vi "Probe_ESR_Verification.vi"() -> ()   [LabVIEW 2020]
uses:
  Instruments/Vector Network Analyzer/Controls/Sparameter cluster.ctl
  Instruments/Vector Network Analyzer/VNA-ZNB/VNA-ZNB.lvclass
  Instruments/Vector Network Analyzer/Vector Network Analyzer.lvclass
  C:/Sandbox/Git_Sandbox/WiSpry Test Framework source code (LV20)/WiSpry Test Framework/Instruments/Instrument.lvclass
  Instruments/Vector Network Analyzer/VNA-Ag87xx/VNA-Ag87xx.lvclass
  Instruments/Vector Network Analyzer/VNA-ENA/VNA-ENA.lvclass
  C:/Sandbox/Git_Sandbox/WiSpry Test Framework source code (LV20)/WiSpry Test Framework/Instruments/Vector Network Analyzer/Vector Network Analyzer.lvclass
  Instruments/Vector Network Analyzer/VNA-FieldFox/VNA-FieldFox.lvclass
  Instruments/Instrument.lvclass/Instrument.ctl
  <vilib>/addons/HF Network Analysis/Support VIs/Read SnP File (SnP).vi
  <vilib>/addons/HF Network Analysis/NI_HFNetworkAnalysis.lvlib
  Instruments/Instrument.lvclass
panel:
  out "Shunt Resistance":cluster{"Frequencies (Hz)":dbl[], dbl[]}[](graph)
  in  "VISA resource name":refnum<visa-resource-name>="GPIB0::24::INSTR"
  in  "Min Loop Delay (ms)":u32=2000
  in  "stop":bool
  in  "VNA ports":bool[](array[boolean])=[TRUE, TRUE, FALSE, FALSE]
  out "error out":errorcluster
  in  "error in (no error)":errorcluster
  out "S parameters":T1[](array[typedef])=[{"Frequency"=100000.0, "S Parameters"=[1.00063102545-0.00317405238764i, -7.98294684912e-06+3.80004461168e-06i, -9.89227074681e-06+6.97421338234e-06i, 1.00037660372-0.00266654479791i]}, {"Frequency"=5412437.5, "S Parameters"=[0.999589465299-0.00884373938232i, 1.79466351697e-05+0.00108431519392i, -4.77312747689e-05+0.00108840175147i, 0.999264902062-0.00912969708227i]}, {"Frequency"=10724875.0, "S Parameters"=[0.999494373608-0.0176199367958i, 4.11591256995e-05+0.00213681933704i, 3.83120105072e-05+0.00214881958037i, 0.999275380418-0.0180876415298i]}, {"Frequency"=16037312.5, "S Parameters"=[0.999282063454-0.0261251603072i, 8.13206404428e-05+0.00319368968947i, 8.47417919346e-05+0.00320723135129i, 0.999053623411-0.0270577569269i]}, {"Frequency"=21349750.0, "S Parameters"=[0.99906596023-0.034829301326i, 0.000151915131114+0.00425103048761i, 0.000150636990312+0.00427010832182i, 0.998740112702-0.0358850792968i]}, {"Frequency"=26662187.5, "S Parameters"=[0.998715362497-0.0435746112421i, 0.000234659139297+0.00531483419357i, 0.000235376905721+0.00533080558281i, 0.998594136554-0.0448224191034i]}, {"Frequency"=31974625.0, "S Parameters"=[0.998281901504-0.0521668079996i, 0.000338128346419+0.00636537125827i, 0.000334413081756+0.00639109675178i, 0.998175718066-0.0537300663822i]}, {"Frequency"=37287062.5, "S Parameters"=[0.997838086619-0.0607938999828i, 0.000461144482836+0.00741328025649i, 0.000459259121093+0.00743917316995i, 0.997503941205-0.0625111061962i]}, {"Frequency"=42599500.0, "S Parameters"=[0.997301968613-0.0694104406755i, 0.000598647928574+0.00846671626162i, 0.000598991319687+0.00849745924638i, 0.996767834563-0.0713509671284i]}, {"Frequency"=47911937.5, "S Parameters"=[0.996738500175-0.0781355874827i, 0.00076500598186+0.00952078341747i, 0.000756830766138+0.00954951785153i, 0.996165848801-0.0802924359967i]}, {"Frequency"=53224375.0, "S Parameters"=[0.995935887891-0.0867413890739i, 0.000935135496371+0.0105724006276i, 0.000930398477704+0.0105994515656i, 0.995431755326-0.0891744067202i]}, {"Frequency"=58536812.5, "S Parameters"=[0.995133720611-0.0953832879489i, 0.00113382618367+0.0116128119096i, 0.00112500139336+0.0116503317168i, 0.99455094616-0.0979411527267i]}, {"Frequency"=63849250.0, "S Parameters"=[0.994282619127-0.104018437494i, 0.00134607137472+0.0126520756157i, 0.00133748264184+0.012683381439i, 0.993711947585-0.106706905878i]}, {"Frequency"=69161687.5, "S Parameters"=[0.993312980895-0.112559684303i, 0.00157379963675+0.0136973250881i, 0.0015692313252+0.0137371922269i, 0.992690963519-0.115458073775i]}, {"Frequency"=74474125.0, "S Parameters"=[0.992169037066-0.121189214253i, 0.00182431843167+0.0147267134348i, 0.00182427780941+0.014777438941i, 0.991560855793-0.124163931681i]}, {"Frequency"=79786562.5, "S Parameters"=[0.991034206753-0.129908888951i, 0.00208671197242+0.0157700205624i, 0.00208852040958+0.0158076067585i, 0.990465792271-0.13280288183i]}, {"Frequency"=85099000.0, "S Parameters"=[0.989888897268-0.138525429622i, 0.00236552862787+0.0167963759004i, 0.00237608265702+0.0168444023872i, 0.98918672108-0.141409756953i]}, {"Frequency"=90411437.5, "S Parameters"=[0.988605222646-0.147144211174i, 0.0026748304552+0.0178246861595i, 0.00268143391082+0.0178659609454i, 0.987792003195-0.150202067637i]}, {"Frequency"=95723875.0, "S Parameters"=[0.987126158904-0.155668326581i, 0.00300270219103+0.018849837706i, 0.00300633583591+0.0188876377234i, 0.98650322677-0.158733542088i]}, {"Frequency"=101036312.5, "S Parameters"=[0.985729529386-0.164429733932i, 0.003342637213+0.019866815485i, 0.00334986844833+0.0199059321685i, 0.985007567168-0.167494141546i]}, {"Frequency"=106348750.0, "S Parameters"=[0.984145047702-0.173009157642i, 0.00370726024826+0.0208751436204i, 0.00370504834329+0.0209018177297i, 0.983494178049-0.176169746823i]}, {"Frequency"=111661187.5, "S Parameters"=[0.982531329981-0.181577975756i, 0.00407539580636+0.0218759411548i, 0.00408254152419+0.0219074554705i, 0.981921526896-0.184855225871i]}, {"Frequency"=116973625.0, "S Parameters"=[0.980942320193-0.190103877786i, 0.00447690972486+0.022883152241i, 0.00446462121407+0.0228866566375i, 0.980236781773-0.193521635504i]}, {"Frequency"=122286062.5, "S Parameters"=[0.979267726477-0.19860375658i, 0.00489476368483+0.0238764594776i, 0.004886375881+0.023872559194i, 0.978522333805-0.202225294481i]}, {"Frequency"=127598500.0, "S Parameters"=[0.97745032036-0.207014881573i, 0.00531411046366+0.0248597210447i, 0.00531499623159+0.0248611893595i, 0.976598530543-0.210843463605i]}, {"Frequency"=132910937.5, "S Parameters"=[0.975642374558-0.215402303724i, 0.00576005483985+0.0258598491544i, 0.00575535538642+0.0258562889893i, 0.974718766285-0.219406816475i]}, {"Frequency"=138223375.0, "S Parameters"=[0.973779428409-0.223714838767i, 0.00620125629282+0.0268525306285i, 0.0062150730737+0.0268593271773i, 0.972777098117-0.228067706274i]}, {"Frequency"=143535812.5, "S Parameters"=[0.971864538252-0.231914322701i, 0.0066698240782+0.0278545247324i, 0.00669008917111+0.0278587055618i, 0.970740525182-0.236637927309i]}, {"Frequency"=148848250.0, "S Parameters"=[0.969858602818-0.24017398174i, 0.00714484521601+0.0288240094733i, 0.00717944034219+0.0288455550671i, 0.968579769524-0.245224863132i]}, {"Frequency"=154160687.5, "S Parameters"=[0.967651604237-0.248352144434i, 0.00765838225549+0.0297911059014i, 0.00768294313807+0.0297998019629i, 0.966448068571-0.253680445193i]}, {"Frequency"=159473125.0, "S Parameters"=[0.965543712114-0.256521744478i, 0.00818962389069+0.0307310624261i, 0.0082211800598+0.0307625609364i, 0.964159725636-0.262205556328i]}, {"Frequency"=164785562.5, "S Parameters"=[0.96335337765-0.264663605956i, 0.00876310221848+0.03166301653i, 0.00877210655779+0.0316950178866i, 0.961821785853-0.270651731496i]}, {"Frequency"=170098000.0, "S Parameters"=[0.961126337593-0.272808308947i, 0.00934062112452+0.0325851442338i, 0.00933990780437+0.032637563282i, 0.959344260473-0.279201035756i]}, {"Frequency"=175410437.5, "S Parameters"=[0.95868103847-0.280857081294i, 0.00993632555241+0.0334996882576i, 0.00992616476105+0.0335484023094i, 0.956752441906-0.287451413347i]}, {"Frequency"=180722875.0, "S Parameters"=[0.956111696266-0.288907064473i, 0.0105479433039+0.0344099917136i, 0.0105194114406+0.0344549228692i, 0.954058536085-0.295745111224i]}, {"Frequency"=186035312.5, "S Parameters"=[0.953438240007-0.297005345647i, 0.011154811883+0.035309936005i, 0.0111504453256+0.0353622915195i, 0.951369766025-0.304053743839i]}, {"Frequency"=191347750.0, "S Parameters"=[0.950854267844-0.305135135687i, 0.0118065287014+0.0362019195547i, 0.0117773805531+0.0362606828664i, 0.948445293457-0.312352376139i]}, {"Frequency"=196660187.5, "S Parameters"=[0.948163629123-0.313306920281i, 0.0124573244177+0.0371009663331i, 0.0124228215186+0.0371566342657i, 0.945697371816-0.320691681687i]}, {"Frequency"=201972625.0, "S Parameters"=[0.945510619226-0.321503691859i, 0.0131130876497+0.0379772095792i, 0.0130861846599+0.0380412858467i, 0.942752796157-0.329091441074i]}, {"Frequency"=207285062.5, "S Parameters"=[0.942720117993-0.329598124505i, 0.0138046739658+0.0388469308322i, 0.0137691724802+0.038916705868i, 0.939877390723-0.337385698885i]}, {"Frequency"=212597500.0, "S Parameters"=[0.939738477428-0.337674230529i, 0.0144851430877+0.0397092340249i, 0.0144560807582+0.0397675182765i, 0.93680182358-0.345504771036i]}, {"Frequency"=217909937.5, "S Parameters"=[0.93663277494-0.345707563034i, 0.0151908676727+0.0405526276046i, 0.0151649299722+0.0406193604774i, 0.933582875935-0.353711316818i]}, {"Frequency"=223222375.0, "S Parameters"=[0.933517598665-0.353872545933i, 0.0159174295466+0.0413924449798i, 0.0159035934482+0.0414574207915i, 0.930330599299-0.361905072381i]}, {"Frequency"=228534812.5, "S Parameters"=[0.93033297528-0.361965447476i, 0.0166747471873+0.0422192563767i, 0.0166489433405+0.0422957168236i, 0.927123433755-0.370150755983i]}, {"Frequency"=233847250.0, "S Parameters"=[0.927088808025-0.370109531166i, 0.0174401322567+0.0430328490142i, 0.0174154172761+0.0431134621313i, 0.923788961735-0.378435441607i]}, {"Frequency"=239159687.5, "S Parameters"=[0.923835292828-0.378306111926i, 0.018223140396+0.0438558269936i, 0.0182121991047+0.0439232862196i, 0.920428121155-0.386655669362i]}, {"Frequency"=244472125.0, "S Parameters"=[0.920371852944-0.386385688171i, 0.0190121292772+0.0446421698344i, 0.0190166229403+0.0447201527773i, 0.916914037433-0.394932787633i]}, {"Frequency"=249784562.5, "S Parameters"=[0.916902278884-0.394458025771i, 0.0198196055669+0.0454280145577i, 0.0198392019368+0.045505608285i, 0.913340158274-0.402934235509i]}, {"Frequency"=255097000.0, "S Parameters"=[0.913274178207-0.402331018193i, 0.02064440953+0.046201470566i, 0.0206499341348+0.0462814568028i, 0.90963607178-0.410919796982i]}, {"Frequency"=260409437.5, "S Parameters"=[0.909443454757-0.410265624646i, 0.0214646749005+0.0469362085321i, 0.0214864653688+0.0470207233435i, 0.905853045196-0.418831053746i]}, {"Frequency"=265721875.0, "S Parameters"=[0.905528988824-0.418142569854i, 0.0223150187518+0.0476575186441i, 0.0223311485529+0.0477642836673i, 0.901908982895-0.426632350287i]}, {"Frequency"=271034312.5, "S Parameters"=[0.901723584779-0.426082738643i, 0.0231902469163+0.0483790402853i, 0.0232004553339+0.0485009765555i, 0.89791245714-0.434590648877i]}, {"Frequency"=276346750.0, "S Parameters"=[0.897712427224-0.433975986603i, 0.0240742237401+0.0490802597868i, 0.0240751967848+0.0492246181039i, 0.893882999092-0.44247426666i]}, {"Frequency"=281659187.5, "S Parameters"=[0.893865687096-0.442023719168i, 0.0249623640111+0.0497794440534i, 0.0249646307093+0.0499333671103i, 0.88985726475-0.450328757258i]}, {"Frequency"=286971625.0, "S Parameters"=[0.889862751082-0.44971670209i, 0.0258712811882+0.050458713556i, 0.0258578159208+0.0506158891927i, 0.885752624932-0.458126842961i]}, {"Frequency"=292284062.5, "S Parameters"=[0.885948665325-0.45743698911i, 0.0267723294974+0.0511306857042i, 0.0267546501657+0.0512938719607i, 0.881755407578-0.465840892567i]}, {"Frequency"=297596500.0, "S Parameters"=[0.882010908203-0.464947823659i, 0.0276911929797+0.0517861331747i, 0.0276624697611+0.0519700884475i, 0.877655277138-0.473393459149i]}, {"Frequency"=302908937.5, "S Parameters"=[0.877895367719-0.472237437836i, 0.0286089085133+0.0524462839516i, 0.0285737476463+0.0526083353161i, 0.873389220201-0.480777133903i]}, {"Frequency"=308221375.0, "S Parameters"=[0.873730319648-0.479579595673i, 0.0295306670691+0.0530839527557i, 0.0295097458178+0.0532290761638i, 0.86908046-0.488190826053i]}, {"Frequency"=313533812.5, "S Parameters"=[0.869502610713-0.48687619568i, 0.0304902651296+0.0537170427797i, 0.0304502934163+0.0538338230389i, 0.864783830391-0.495718273581i]}, {"Frequency"=318846250.0, "S Parameters"=[0.86536131508-0.494041353269i, 0.0314430105507+0.0543631836035i, 0.0314343793546+0.0544412165234i, 0.86043056023-0.50297290057i]}, {"Frequency"=324158687.5, "S Parameters"=[0.861101958051-0.501219109139i, 0.0324163421203+0.0549798985744i, 0.0324408757901+0.0550453222631i, 0.855902533376-0.510362440212i]}, {"Frequency"=329471125.0, "S Parameters"=[0.856790946408-0.508440878483i, 0.0334061528754+0.0556010151243i, 0.0334443069802+0.0556165063967i, 0.851467855791-0.517830817251i]}, {"Frequency"=334783562.5, "S Parameters"=[0.852504965756-0.515638294093i, 0.0344265507048+0.0561953452312i, 0.034472083246+0.0562000701666i, 0.846852096741-0.525172965022i]}, {"Frequency"=340096000.0, "S Parameters"=[0.848223335605-0.522834872411i, 0.0354529947731+0.0567842918775i, 0.0355104835193+0.0567651452848i, 0.842287633675-0.532688661039i]}, {"Frequency"=345408437.5, "S Parameters"=[0.843776876771-0.529849159751i, 0.0364824957151+0.0573676534415i, 0.0365586722173+0.0573231992306i, 0.837600930932-0.539966617959i]}, {"Frequency"=350720875.0, "S Parameters"=[0.839192629354-0.536820222493i, 0.0375118522588+0.0579177012483i, 0.0376174747675+0.0578693578765i, 0.83270253535-0.547033038051i]}, {"Frequency"=356033312.5, "S Parameters"=[0.834445445728-0.543747254366i, 0.0385684217528+0.0584310680257i, 0.0386668668805+0.0583952036463i, 0.827662438937-0.554318170324i]}, {"Frequency"=361345750.0, "S Parameters"=[0.829592983985-0.550741502233i, 0.0396452864452+0.058929027604i, 0.0397361347819+0.0589183368508i, 0.822650176586-0.561367866726i]}, {"Frequency"=366658187.5, "S Parameters"=[0.824564699915-0.557812446697i, 0.0407427716736+0.0594142207705i, 0.0408107962368+0.0593953549477i, 0.817435327165-0.568694712837i]}, {"Frequency"=371970625.0, "S Parameters"=[0.819574977073-0.564915115575i, 0.0418456361+0.0598759028534i, 0.0418988472337+0.0599005185004i, 0.812175410235-0.575744831474i]}, {"Frequency"=377283062.5, "S Parameters"=[0.814388360027-0.572091045977i, 0.0429730034406+0.0603183945285i, 0.0429872678536+0.0603435292067i, 0.806970477432-0.582971207729i]}, {"Frequency"=382595500.0, "S Parameters"=[0.809502852485-0.579172175507i, 0.0441051368128+0.0607466496275i, 0.0440878250853+0.0608084246741i, 0.801815215926-0.59009752885i]}, {"Frequency"=387907937.5, "S Parameters"=[0.804332658222-0.586167701733i, 0.0452336363873+0.0611522577662i, 0.0451849462962+0.0612286388754i, 0.796573022135-0.596995908343i]}, {"Frequency"=393220375.0, "S Parameters"=[0.799157493995-0.593065593031i, 0.0463719042317+0.0615489642622i, 0.0462857416515+0.0616423958993i, 0.791284266201-0.603844152373i]}, {"Frequency"=398532812.5, "S Parameters"=[0.79391205451-0.599924311835i, 0.0475019510099+0.0619496720782i, 0.0474051568781+0.0620315825637i, 0.785991172982-0.610558039527i]}, {"Frequency"=403845250.0, "S Parameters"=[0.788778217704-0.606655185552i, 0.0486411719472+0.0623505265199i, 0.0485377088771+0.0624126725359i, 0.780821444863-0.617192889185i]}, {"Frequency"=409157687.5, "S Parameters"=[0.783530712615-0.613295818833i, 0.0497772098106+0.062698768358i, 0.0496945812296+0.0627570840774i, 0.775486892195-0.623623820526i]}, {"Frequency"=414470125.0, "S Parameters"=[0.77820733929-0.619992321306i, 0.050936074167+0.0630697016741i, 0.0508671483103+0.0630876636642i, 0.770152571985-0.630232778601i]}, {"Frequency"=419782562.5, "S Parameters"=[0.772836148572-0.626504467508i, 0.0521288026674+0.0633783353291i, 0.0520507657099+0.0634041388604i, 0.764596100379-0.636815902177i]}, {"Frequency"=425095000.0, "S Parameters"=[0.767424170262-0.633026435217i, 0.0533043900706+0.0637117627889i, 0.0532559275066+0.0636936884446i, 0.759130623007-0.643352525514i]}, {"Frequency"=430407437.5, "S Parameters"=[0.761997679212-0.639488959115i, 0.0545106689513+0.0639946568128i, 0.0544766884357+0.0639797172283i, 0.753587638453-0.649767373366i]}, {"Frequency"=435719875.0, "S Parameters"=[0.756472262109-0.645944466079i, 0.0557056726007+0.0642909498324i, 0.0557123249982+0.0642243999468i, 0.747934758954-0.656110691818i]}, {"Frequency"=441032312.5, "S Parameters"=[0.750790337166-0.652102929128i, 0.0569155840497+0.0645461079911i, 0.0569475623612+0.0644838826163i, 0.742218207836-0.662221655766i]}, {"Frequency"=446344750.0, "S Parameters"=[0.745143695163-0.658294914948i, 0.0581141944168+0.0647843160559i, 0.0581715513229+0.0647497455839i, 0.736110747732-0.668350272847i]}, {"Frequency"=451657187.5, "S Parameters"=[0.739234247641-0.664462186289i, 0.0593287830504+0.0650134546916i, 0.0593858728144+0.0649575650675i, 0.730268615428-0.674614490715i]}, {"Frequency"=456969625.0, "S Parameters"=[0.733338337278-0.670588208003i, 0.0605640956685+0.0652023065333i, 0.0606018030058+0.0651718625086i, 0.724181204514-0.68086071557i]}, {"Frequency"=462282062.5, "S Parameters"=[0.727323292454-0.677012939928i, 0.0617976955719+0.0653836571187i, 0.0618493121326+0.0653632907481i, 0.71801648867-0.687161677924i]}, {"Frequency"=467594500.0, "S Parameters"=[0.721180102656-0.683338511352i, 0.0630531840805+0.0655317460434i, 0.0630691552869+0.0655237723636i, 0.711877821348-0.693383927429i]}, {"Frequency"=472906937.5, "S Parameters"=[0.715056132992-0.689623185694i, 0.0643249103696+0.0656398062479i, 0.0643039251735+0.0656931443031i, 0.705594951816-0.699579704496i]}, {"Frequency"=478219375.0, "S Parameters"=[0.708901824002-0.695888362785i, 0.065576682043+0.0657625277186i, 0.0655418641159+0.065816331645i, 0.699511120301-0.705688921593i]}, {"Frequency"=483531812.5, "S Parameters"=[0.702643558904-0.702096027427i, 0.0668587222734+0.0658507852596i, 0.0667826774553+0.0659223674517i, 0.693236369102-0.711736379121i]}, {"Frequency"=488844250.0, "S Parameters"=[0.696381949504-0.708338617123i, 0.0681237179335+0.0659217670994i, 0.0680349129524+0.0660057232637i, 0.686905261408-0.717657421781i]}, {"Frequency"=494156687.5, "S Parameters"=[0.69024820324-0.71423661451i, 0.0694065706979+0.066007594938i, 0.0692901344825+0.0660990310715i, 0.680648559345-0.723562997539i]}, {"Frequency"=499469125.0, "S Parameters"=[0.683878992516-0.720069238751i, 0.0706614121248+0.0660506888409i, 0.0705352056018+0.0661621518603i, 0.674314933524-0.729302727123i]}, {"Frequency"=504781562.5, "S Parameters"=[0.67765735774-0.725764776545i, 0.071918876+0.0660959512079i, 0.0717989086346+0.0662032939569i, 0.667972849895-0.734955923686i]}, {"Frequency"=510094000.0, "S Parameters"=[0.671298841094-0.731538902354i, 0.0731693546933+0.0661270859203i, 0.0730695672455+0.066225488051i, 0.66147669786-0.740548360181i]}, {"Frequency"=515406437.5, "S Parameters"=[0.664956361856-0.737217852867i, 0.0744387117538+0.0661166831921i, 0.0743496314046+0.0662153269034i, 0.654988599127-0.746174047555i]}, {"Frequency"=520718875.0, "S Parameters"=[0.658664005375-0.742773372804i, 0.075711147919+0.066103974408i, 0.0756690720924+0.0661833406382i, 0.648442140988-0.751805839216i]}, {"Frequency"=526031312.5, "S Parameters"=[0.652239932201-0.748063076522i, 0.076996186472+0.0660559163416i, 0.0769692504695+0.0661410777289i, 0.641595507546-0.75727104644i]}, {"Frequency"=531343750.0, "S Parameters"=[0.645772802832-0.753308373537i, 0.0782781036799+0.0660001682736i, 0.0782614495057+0.0660720748261i, 0.634837568913-0.762675738101i]}, {"Frequency"=536656187.5, "S Parameters"=[0.639243540198-0.758447584388i, 0.0795380771291+0.0659074629919i, 0.079575528085+0.0659716708719i, 0.627916433614-0.767844158065i]}, {"Frequency"=541968625.0, "S Parameters"=[0.632673662842-0.763543687601i, 0.0808173461883+0.0658173179721i, 0.0808657213996+0.0658693844852i, 0.62073934413-0.773207369049i]}, {"Frequency"=547281062.5, "S Parameters"=[0.626123719122-0.768700052511i, 0.0820963974813+0.0657209933489i, 0.0821853874253+0.0657734103431i, 0.613723284936-0.778585225678i]}, {"Frequency"=552593500.0, "S Parameters"=[0.619462380416-0.773755227441i, 0.0833766785012+0.0655979258002i, 0.0834833371479+0.0656312593138i, 0.606590051175-0.783862312302i]}, {"Frequency"=557905937.5, "S Parameters"=[0.613000813159-0.778868203976i, 0.084668832196+0.0654633464949i, 0.0847912954215+0.0654930092841i, 0.599622462726-0.789366063614i]}, {"Frequency"=563218375.0, "S Parameters"=[0.606264495995-0.783970903666i, 0.0859810577266+0.065285433265i, 0.0861088243739+0.0652928574811i, 0.592390894454-0.794706534192i]}, {"Frequency"=568530812.5, "S Parameters"=[0.599654918058-0.789003711758i, 0.0872746381079+0.0650901480533i, 0.0873966460723+0.0650991877521i, 0.585242834728-0.799845997629i]}, {"Frequency"=573843250.0, "S Parameters"=[0.592907200459-0.794091240443i, 0.0885817038622+0.0648851593623i, 0.0887196137592+0.0648724994204i, 0.577981526664-0.804972752397i]}, {"Frequency"=579155687.5, "S Parameters"=[0.585980944557-0.798980962821i, 0.0898975487383+0.0646487818453i, 0.0900405466608+0.0646137883089i, 0.57074380165-0.810062255945i]}, {"Frequency"=584468125.0, "S Parameters"=[0.579113969756-0.803856885489i, 0.0911973184415+0.0644296738465i, 0.0913529867057+0.0643706386572i, 0.563589247893-0.814943683832i]}, {"Frequency"=589780562.5, "S Parameters"=[0.572218650898-0.808571802939i, 0.0925177960827+0.0641742472972i, 0.0926493258312+0.0640892654375i, 0.556427328877-0.819721753221i]}, {"Frequency"=595093000.0, "S Parameters"=[0.565252888639-0.813310430635i, 0.0938070030138+0.0638961087118i, 0.0939501356548+0.0638102737035i, 0.549129157433-0.824369434062i]}, {"Frequency"=600405437.5, "S Parameters"=[0.558260130511-0.818007086325i, 0.0950905034125+0.0636177573095i, 0.0952452132801+0.0635361352387i, 0.541881907262-0.82902027769i]}, {"Frequency"=605717875.0, "S Parameters"=[0.551383962105-0.82259900329i, 0.0963677361442+0.0633349434215i, 0.0965263194209+0.0632520565912i, 0.534817068005-0.833458140245i]}, {"Frequency"=611030312.5, "S Parameters"=[0.544501299363-0.827095526201i, 0.0976577871601+0.0630390906843i, 0.097793573854+0.06293909167i, 0.527829178505-0.837769904569i]}, {"Frequency"=616342750.0, "S Parameters"=[0.537370454041-0.831504869875i, 0.0989663259905+0.0626738407556i, 0.0990784363786+0.0625815969942i, 0.520459165976-0.842067640028i]}, {"Frequency"=621655187.5, "S Parameters"=[0.530291434527-0.83572301726i, 0.10027766324+0.062296240104i, 0.100345517323+0.0622154231724i, 0.513082454146-0.846164707614i]}, {"Frequency"=626967625.0, "S Parameters"=[0.523123672041-0.839902811715i, 0.101609076916+0.0618859968706i, 0.101638045696+0.061822712959i, 0.505564751847-0.850328107763i]}, {"Frequency"=632280062.5, "S Parameters"=[0.515847197209-0.84404704414i, 0.102931533812+0.0614691329142i, 0.102905571585+0.0613900452211i, 0.497950875324-0.854398869408i]}, {"Frequency"=637592500.0, "S Parameters"=[0.508705354697-0.848129952343i, 0.104234086297+0.0610614772917i, 0.104180095722+0.0609795636739i, 0.490397216695-0.858438578937i]}, {"Frequency"=642904937.5, "S Parameters"=[0.501420465553-0.852238275235i, 0.105564299661+0.060621857435i, 0.105466771499+0.0605304015747i, 0.48277683392-0.862660914991i]}, {"Frequency"=648217375.0, "S Parameters"=[0.494263051028-0.856279265944i, 0.106874050247+0.0601737454206i, 0.106746021727+0.0600669030824i, 0.475319289168-0.866804339773i]}, {"Frequency"=653529812.5, "S Parameters"=[0.487048039027-0.860313760594i, 0.108169091111+0.0597044215349i, 0.108030588973+0.059600832678i, 0.467704078167-0.870848136957i]}, {"Frequency"=658842250.0, "S Parameters"=[0.479739307513-0.864305904978i, 0.109494910474+0.0591891917499i, 0.109327557476+0.0590834061535i, 0.460046560179-0.874880011026i]}, {"Frequency"=664154687.5, "S Parameters"=[0.4723898478-0.868228979692i, 0.110802961896+0.058680468252i, 0.110672893101+0.0585503280393i, 0.452370240397-0.878784751825i]}, {"Frequency"=669467125.0, "S Parameters"=[0.465009728218-0.872039932738i, 0.112121744195+0.0581172327766i, 0.111990627111+0.0580107098431i, 0.44462208069-0.882748168249i]}, {"Frequency"=674779562.5, "S Parameters"=[0.457427954735-0.875872592683i, 0.11341895078+0.057527667223i, 0.11333897457+0.0574317891891i, 0.436731778027-0.886348195179i]}, {"Frequency"=680092000.0, "S Parameters"=[0.449758184396-0.879487925529i, 0.114717579508+0.0568991445274i, 0.114647297665+0.0568042666825i, 0.428868231336-0.89003818492i]}, {"Frequency"=685404437.5, "S Parameters"=[0.442079198894-0.883260295475i, 0.1159895558+0.0563031422455i, 0.115973656461+0.0561961895293i, 0.42112826238-0.893604115276i]}, {"Frequency"=690716875.0, "S Parameters"=[0.434364884014-0.88696288913i, 0.117277631417+0.0556378649597i, 0.117287635135+0.0555592240809i, 0.41312840864-0.897228949146i]}, {"Frequency"=696029312.5, "S Parameters"=[0.426698221326-0.890564220841i, 0.118512794026+0.0550056838551i, 0.118558000746+0.0549291600593i, 0.405340911629-0.900584444494i]}, {"Frequency"=701341750.0, "S Parameters"=[0.419043862782-0.89411839011i, 0.119779031829+0.0543546227086i, 0.119813636212+0.0543036595544i, 0.397662299689-0.90401720617i]}, {"Frequency"=706654187.5, "S Parameters"=[0.411321821766-0.89748210318i, 0.120998937643+0.0536402691663i, 0.121025412774+0.0536114468749i, 0.389887391833-0.907079071441i]}, {"Frequency"=711966625.0, "S Parameters"=[0.403569145007-0.900740740003i, 0.122231629229+0.052938441763i, 0.122236025504+0.0529047760896i, 0.381830567398-0.910205559899i]}, {"Frequency"=717279062.5, "S Parameters"=[0.395641374117-0.903988956131i, 0.123446782356+0.0522106604013i, 0.123453766922+0.0521693747288i, 0.373963517445-0.913074668899i]}, {"Frequency"=722591500.0, "S Parameters"=[0.387831331921-0.907230241407i, 0.124674895368+0.0514288994023i, 0.124639324717+0.0514211048994i, 0.365893722565-0.915999148861i]}, {"Frequency"=727903937.5, "S Parameters"=[0.380034461493-0.910213174666i, 0.125890087398+0.0506791707926i, 0.125814873285+0.0506447136441i, 0.357963742297-0.919020287614i]}, {"Frequency"=733216375.0, "S Parameters"=[0.37222943743-0.913351479019i, 0.127094089869+0.0498896720059i, 0.126959269552+0.0498821328295i, 0.349914632687-0.921997695758i]}, {"Frequency"=738528812.5, "S Parameters"=[0.364502994792-0.916427459124i, 0.128297782903+0.0491211442222i, 0.128134042678+0.0490829576297i, 0.342189336209-0.924948641756i]}, {"Frequency"=743841250.0, "S Parameters"=[0.356864743479-0.91933735348i, 0.129459149935+0.0483269640262i, 0.129273322397+0.0482675448199i, 0.334255270547-0.92774244258i]}, {"Frequency"=749153687.5, "S Parameters"=[0.349405407125-0.92226512687i, 0.130654438931+0.0475458103177i, 0.130473388811+0.0474953498938i, 0.326460167834-0.93053488536i]}, {"Frequency"=754466125.0, "S Parameters"=[0.341870912319-0.925026119787i, 0.131822213094+0.0467545860475i, 0.131642583377+0.046698240513i, 0.318703709334-0.933231204444i]}, {"Frequency"=759778562.5, "S Parameters"=[0.334290069046-0.927511160524i, 0.132971787354+0.0459540862484i, 0.132818146055+0.045893700235i, 0.310806866589-0.935609338275i]}, {"Frequency"=765091000.0, "S Parameters"=[0.326658317141-0.930080741749i, 0.134133596112+0.0451163263279i, 0.134030337884+0.0450541593751i, 0.302872573016-0.938038963092i]}, {"Frequency"=770403437.5, "S Parameters"=[0.318889272112-0.932536771179i, 0.135326970454+0.0442393305939i, 0.135260261728+0.0441894330365i, 0.294836522403-0.940456539207i]}, {"Frequency"=775715875.0, "S Parameters"=[0.31110115001-0.935009380681i, 0.136488653244+0.043352436968i, 0.136435415734+0.0433300137784i, 0.286735317121-0.942729106003i]}, {"Frequency"=781028312.5, "S Parameters"=[0.303187030066-0.937231078137i, 0.137635315492+0.0424341089309i, 0.137647206278+0.0424351121541i, 0.278577345409-0.944976795522i]}, {"Frequency"=786340750.0, "S Parameters"=[0.295454505339-0.939616264127i, 0.13879549029+0.0415051330053i, 0.138817872744+0.0415571861569i, 0.270421561923-0.947134037998i]}, {"Frequency"=791653187.5, "S Parameters"=[0.287553822214-0.941794469701i, 0.13993458601+0.0405965508472i, 0.139998494836+0.040626335971i, 0.262429458723-0.94922210278i]}, {"Frequency"=796965625.0, "S Parameters"=[0.279659265085-0.943845740864i, 0.141031960025+0.039645151318i, 0.141132113166+0.0396940691225i, 0.254332360397-0.951076815641i]}, {"Frequency"=802278062.5, "S Parameters"=[0.271704175382-0.945877455128i, 0.142132806586+0.0386755003422i, 0.142235464911+0.03872967897i, 0.246247395847-0.952856962908i]}, {"Frequency"=807590500.0, "S Parameters"=[0.263808126146-0.947856639006i, 0.143250841601+0.0377017619258i, 0.143355607501+0.0377765985504i, 0.238041281306-0.954671462047i]}, {"Frequency"=812902937.5, "S Parameters"=[0.255822005378-0.949662366132i, 0.144346402016+0.0367181143106i, 0.144412531857+0.0367325274008i, 0.229685215586-0.956291110613i]}, {"Frequency"=818215375.0, "S Parameters"=[0.247703632343-0.951633272918i, 0.145462222438+0.0356511197499i, 0.1454651801+0.0357008644356i, 0.221305092611-0.95801092555i]}, {"Frequency"=823527812.5, "S Parameters"=[0.239645841085-0.953542600096i, 0.146522429769+0.0346328657989i, 0.146534610694+0.034628126227i, 0.213053410669-0.959791930291i]}, {"Frequency"=828840250.0, "S Parameters"=[0.231607003512-0.955444388361i, 0.147593089707+0.0335640760988i, 0.147563031924+0.0335228918968i, 0.204689490621-0.961463012338i]}, {"Frequency"=834152687.5, "S Parameters"=[0.223600745045-0.957414482021i, 0.148678137706+0.0325243396646i, 0.148625846506+0.032429941883i, 0.196561143212-0.963183326779i]}, {"Frequency"=839465125.0, "S Parameters"=[0.215666605825-0.959258163384i, 0.149713421079+0.0314326411463i, 0.14968707016+0.0313311861147i, 0.18820707522-0.964685126725i]}, {"Frequency"=844777562.5, "S Parameters"=[0.20782623822-0.960892930389i, 0.150784166152+0.030364099139i, 0.150721844274+0.0302515539173i, 0.180141420047-0.966277859997i]}, {"Frequency"=850090000.0, "S Parameters"=[0.200051077849-0.962375855075i, 0.151836080788+0.0292660601734i, 0.151768323969+0.0291558805843i, 0.171860245176-0.96744266787i]}, {"Frequency"=855402437.5, "S Parameters"=[0.192192510447-0.963826810986i, 0.152893747077+0.0281769870832i, 0.152807848892+0.0280449464101i, 0.163594587411-0.968754188247i]}, {"Frequency"=860714875.0, "S Parameters"=[0.184130320494-0.965170412097i, 0.153925065254+0.0270457634222i, 0.153848299479+0.0268871586158i, 0.155326758135-0.969824893287i]}, {"Frequency"=866027312.5, "S Parameters"=[0.176105513979-0.966378467951i, 0.154967212215+0.0259007219175i, 0.15486962542+0.0257270975193i, 0.146873700226-0.970996784025i]}, {"Frequency"=871339750.0, "S Parameters"=[0.168009770535-0.967701303539i, 0.156005220252+0.0247016964851i, 0.155917083469+0.0245531320403i, 0.138366349179-0.972056859775i]}, {"Frequency"=876652187.5, "S Parameters"=[0.159769508311-0.968834074513i, 0.15701474064+0.0234670197131i, 0.15693957835+0.0233125299611i, 0.129776118286-0.97297240355i]}, {"Frequency"=881964625.0, "S Parameters"=[0.151361369802-0.969847690592i, 0.158003996432+0.0222189546446i, 0.157940461774+0.0220294887817i, 0.121240263033-0.973687103112i]}, {"Frequency"=887277062.5, "S Parameters"=[0.142906701936-0.970787784384i, 0.158995908119+0.0209336762908i, 0.158927958953+0.02073982447i, 0.112567945121-0.974534410108i]}, {"Frequency"=892589500.0, "S Parameters"=[0.134562169644-0.97162719436i, 0.159978141666+0.0196183262033i, 0.159862552665+0.0194497166122i, 0.103918708708-0.975093251918i]}, {"Frequency"=897901937.5, "S Parameters"=[0.1260309028-0.97243567182i, 0.160890435737+0.0183012042795i, 0.160826310571+0.0181466414902i, 0.0952860647617-0.975559367784i]}, {"Frequency"=903214375.0, "S Parameters"=[0.117476278726-0.973241566019i, 0.161805041466+0.0170145325663i, 0.161705075543+0.0168317971531i, 0.0865753303627-0.97616745311i]}, {"Frequency"=908526812.5, "S Parameters"=[0.108736486073-0.973961479698i, 0.162693296387+0.0156513956653i, 0.162606289854+0.0154790172238i, 0.0779405228756-0.976576887798i]}, {"Frequency"=913839250.0, "S Parameters"=[0.100272543994-0.974810293781i, 0.163515863658+0.0142714356309i, 0.163463154889+0.0141232257608i, 0.0693137148197-0.97712993772i]}, {"Frequency"=919151687.5, "S Parameters"=[0.0916710723802-0.975546262852i, 0.164381987123+0.0128979635354i, 0.164288205657+0.0127186595611i, 0.0608190504754-0.977691747644i]}, {"Frequency"=924464125.0, "S Parameters"=[0.0831020003206-0.976241126626i, 0.165215705143+0.0115028593748i, 0.165126251386+0.0113491368025i, 0.0522746479709-0.978225406778i]}, {"Frequency"=929776562.5, "S Parameters"=[0.0747987569421-0.976948478972i, 0.166037366743+0.0101117733998i, 0.165968524275+0.00996911318224i, 0.0439541539833-0.978673649746i]}, {"Frequency"=935089000.0, "S Parameters"=[0.0665417384361-0.97738055295i, 0.166806617476+0.00873726047156i, 0.166765719161+0.00857444081628i, 0.0358017507244-0.978864720395i]}, {"Frequency"=940401437.5, "S Parameters"=[0.0584765941064-0.977817589043i, 0.167602897837+0.00734309019331i, 0.167567295043+0.0071963036243i, 0.0275523899039-0.978821340425i]}, {"Frequency"=945713875.0, "S Parameters"=[0.050411393978-0.977985188409i, 0.16834248994+0.00597810763871i, 0.168302515992+0.00582322513678i, 0.0194221735938-0.978722323246i]}, {"Frequency"=951026312.5, "S Parameters"=[0.0424877742179-0.978319302501i, 0.1691187338+0.00460311532489i, 0.16907170463+0.00447966566943i, 0.0112377031173-0.978748783543i]}, {"Frequency"=956338750.0, "S Parameters"=[0.0347224526448-0.978423068998i, 0.169844299405+0.00324527958117i, 0.169809214581+0.00312777203096i, 0.00312844680329-0.978631921843i]}, {"Frequency"=961651187.5, "S Parameters"=[0.0268893354297-0.978588896895i, 0.170595941125+0.00186607084483i, 0.17049248574+0.00177602001469i, -0.00494445208392-0.97841022052i]}, {"Frequency"=966963625.0, "S Parameters"=[0.019002863679-0.978527803423i, 0.171323823221+0.000465740509664i, 0.171189790807+0.000380798046211i, -0.0131372833982-0.97821111944i]}, {"Frequency"=972276062.5, "S Parameters"=[0.0111768488751-0.978387565435i, 0.172042195218-0.00100079724546i, 0.171845605321-0.00104965348644i, -0.0213856457888-0.977658173329i]}, {"Frequency"=977588500.0, "S Parameters"=[0.003141906885-0.978230389379i, 0.172777855462-0.00246787462386i, 0.172549211973-0.0025161066966i, -0.0297193631821-0.97712937043i]}, {"Frequency"=982900937.5, "S Parameters"=[-0.00482389513468-0.977869725153i, 0.173479771423-0.00393692683027i, 0.173203118037-0.00401489255514i, -0.0380452199843-0.976618668474i]}, {"Frequency"=988213375.0, "S Parameters"=[-0.0127424409323-0.977566447696i, 0.174170748331-0.00546043952312i, 0.173858505125-0.0054543721585i, -0.0464334289088-0.975832012928i]}, {"Frequency"=993525812.5, "S Parameters"=[-0.0208597685201-0.97706663055i, 0.174882966922-0.0069511534676i, 0.174496386159-0.00696069450891i, -0.0549095952186-0.975207249647i]}, {"Frequency"=998838250.0, "S Parameters"=[-0.0290397744921-0.97653894567i, 0.175537030817-0.00847393639668i, 0.175164943311-0.00846769505805i, -0.0633644395629-0.974428363247i]}, {"Frequency"=1004150687.5, "S Parameters"=[-0.0372430015913-0.976133384975i, 0.176155845926-0.00996730944919i, 0.175803173236-0.00998689203082i, -0.0718420014254-0.97371542929i]}, {"Frequency"=1009463125.0, "S Parameters"=[-0.0456139392387-0.975606535102i, 0.176797889222-0.0115210405176i, 0.176436931363-0.0115328799408i, -0.0803430180295-0.973070278956i]}, {"Frequency"=1014775562.5, "S Parameters"=[-0.0537776278667-0.975187892351i, 0.177353131903-0.0130957739647i, 0.177097029014-0.0130699143057i, -0.0887209952443-0.972201575433i]}, {"Frequency"=1020088000.0, "S Parameters"=[-0.0621171275905-0.974650035298i, 0.177950685899-0.0146933108401i, 0.177709348692-0.0146309909555i, -0.0970268460481-0.971425315364i]}, {"Frequency"=1025400437.5, "S Parameters"=[-0.0702903732027-0.973878080505i, 0.178458330232-0.0162988900562i, 0.178335752097-0.0162220420094i, -0.105204831502-0.970256528632i]}, {"Frequency"=1030712875.0, "S Parameters"=[-0.0785473414386-0.972978434409i, 0.178987374416-0.0179051235305i, 0.178926612594-0.0177820573783i, -0.113519593325-0.969115121756i]}, {"Frequency"=1036025312.5, "S Parameters"=[-0.086721548962-0.9722339253i, 0.179490561916-0.0195102490205i, 0.179504633267-0.0193477914736i, -0.121848433377-0.967845114249i]}, {"Frequency"=1041337750.0, "S Parameters"=[-0.0948706265247-0.971156939769i, 0.180007509858-0.0211481068918i, 0.180016140497-0.0209528003977i, -0.130109289143-0.966696387574i]}, {"Frequency"=1046650187.5, "S Parameters"=[-0.102893854439-0.970306264188i, 0.180460476247-0.0227136210812i, 0.180531053609-0.0224914255151i, -0.138020671656-0.965355346431i]}, {"Frequency"=1051962625.0, "S Parameters"=[-0.110870658769-0.969258354766i, 0.180918118253-0.0242808579739i, 0.181005954062-0.024036881757i, -0.146110366514-0.963982839728i]}, {"Frequency"=1057275062.5, "S Parameters"=[-0.118978987652-0.968110126176i, 0.181359838379-0.0258536260174i, 0.181409799594-0.0256395781014i, -0.154142267698-0.962707295173i]}, {"Frequency"=1062587500.0, "S Parameters"=[-0.126877511106-0.967067497416i, 0.181761030666-0.0274681499271i, 0.181800381643-0.0272906905124i, -0.162234690795-0.961020853611i]}, {"Frequency"=1067899937.5, "S Parameters"=[-0.134850427445-0.965721698628i, 0.182182377257-0.029096299118i, 0.182172106095-0.0289451156502i, -0.17021355985-0.95940750093i]}, {"Frequency"=1073212375.0, "S Parameters"=[-0.14289506813-0.964232229607i, 0.18257364283-0.0307226075298i, 0.182526760809-0.0306851675265i, -0.178183647077-0.957550211151i]}, {"Frequency"=1078524812.5, "S Parameters"=[-0.150901496095-0.962605660377i, 0.182982795646-0.0323711347196i, 0.182867564436-0.0324422315964i, -0.186295732755-0.955881505355i]}, {"Frequency"=1083837250.0, "S Parameters"=[-0.158995026306-0.961096060584i, 0.183336282582-0.0340295048432i, 0.183180276288-0.0341447147549i, -0.19432431561-0.953874398519i]}, {"Frequency"=1089149687.5, "S Parameters"=[-0.167106616731-0.959466935109i, 0.183683067166-0.0356715394231i, 0.183509977277-0.0358854119567i, -0.202296390188-0.952029888861i]}, {"Frequency"=1094462125.0, "S Parameters"=[-0.175285245659-0.957809095021i, 0.184036190999-0.037336488037i, 0.183837705056-0.0376174789181i, -0.210308770732-0.949980534816i]}, {"Frequency"=1099774562.5, "S Parameters"=[-0.183398413231-0.956332635258i, 0.184362773446-0.0389642876932i, 0.184152857512-0.0393010171889i, -0.218281304526-0.948221594681i]}, {"Frequency"=1105087000.0, "S Parameters"=[-0.191346530534-0.954735004124i, 0.184684530329-0.0406149025374i, 0.184499774315-0.0409037148774i, -0.226235631603-0.946288956413i]}, {"Frequency"=1110399437.5, "S Parameters"=[-0.199479622388-0.952888618135i, 0.18496191602-0.0423195154362i, 0.184783437096-0.042620352038i, -0.234168808567-0.944306564111i]}, {"Frequency"=1115711875.0, "S Parameters"=[-0.207466765137-0.950952702969i, 0.185208466755-0.0440401238837i, 0.185046411314-0.0442623397753i, -0.242041574539-0.942146806154i]}, {"Frequency"=1121024312.5, "S Parameters"=[-0.215494288496-0.948833721577i, 0.185409540345-0.0457564882315i, 0.185304412177-0.0459646804074i, -0.249768270689-0.939691213715i]}, {"Frequency"=1126336750.0, "S Parameters"=[-0.223574778834-0.946889691061i, 0.18558728759-0.0474898025428i, 0.185503199448-0.0476038908332i, -0.257595808153-0.937372840518i]}, {"Frequency"=1131649187.5, "S Parameters"=[-0.231364981183-0.944670890997i, 0.185786861169-0.0492352501802i, 0.185720813851-0.0492836904434i, -0.265439396571-0.934967984221i]}, {"Frequency"=1136961625.0, "S Parameters"=[-0.239240819836-0.942441695561i, 0.18595498039-0.0509542313904i, 0.185869009874-0.0509344631961i, -0.273118512005-0.932613613018i]}, {"Frequency"=1142274062.5, "S Parameters"=[-0.247163915028-0.940178398956i, 0.186103627066-0.0526630953833i, 0.186027421612-0.0525873568168i, -0.281008834518-0.930060436845i]}, {"Frequency"=1147586500.0, "S Parameters"=[-0.254929253237-0.938051150661i, 0.186233297762-0.0543310701697i, 0.186164576547-0.0542247378545i, -0.288699457263-0.927363084599i]}, {"Frequency"=1152898937.5, "S Parameters"=[-0.262508546911-0.935613589036i, 0.186319626838-0.0560558619116i, 0.186233854544-0.0559395490441i, -0.296275863759-0.924730349431i]}, {"Frequency"=1158211375.0, "S Parameters"=[-0.270112284945-0.933138345773i, 0.18643342254-0.0577502168723i, 0.186338126819-0.0576705294178i, -0.304035357842-0.922029695919i]}, {"Frequency"=1163523812.5, "S Parameters"=[-0.277747813977-0.930770921704i, 0.186484741992-0.0594832795185i, 0.186422181809-0.059409804576i, -0.311410094041-0.919115735017i]}, {"Frequency"=1168836250.0, "S Parameters"=[-0.285081381204-0.928204834866i, 0.186597499519-0.0612550285402i, 0.186452880461-0.0612230894272i, -0.319243487593-0.916254885645i]}, {"Frequency"=1174148687.5, "S Parameters"=[-0.292744221967-0.925593717609i, 0.18662549039-0.0629910319603i, 0.186502028863-0.0630417189718i, -0.326873342663-0.91315601401i]}, {"Frequency"=1179461125.0, "S Parameters"=[-0.30024302925-0.922931258608i, 0.186673192953-0.0647585601166i, 0.186549900719-0.064866562934i, -0.334692992965-0.910123636021i]}, {"Frequency"=1184773562.5, "S Parameters"=[-0.307854052699-0.920219318803i, 0.18669791396-0.0664957670304i, 0.186551921174-0.0666761010081i, -0.342426230961-0.907238627677i]}, {"Frequency"=1190086000.0, "S Parameters"=[-0.31531507764-0.917828236708i, 0.18673502561-0.0682766370839i, 0.18657135552-0.068472793408i, -0.350109020506-0.90419376968i]}, {"Frequency"=1195398437.5, "S Parameters"=[-0.32266270496-0.915198314845i, 0.186715871673-0.0700318567235i, 0.186556824599-0.0702477297747i, -0.357735994491-0.901154415447i]}, {"Frequency"=1200710875.0, "S Parameters"=[-0.329872390906-0.912355820783i, 0.186673246798-0.0717445391365i, 0.186522302467-0.0719891094297i, -0.365082221167-0.898007580571i]}, {"Frequency"=1206023312.5, "S Parameters"=[-0.337110468749-0.909560855447i, 0.18659291719-0.0735134775419i, 0.1864659508-0.0737105293505i, -0.372583208058-0.894700671771i]}, {"Frequency"=1211335750.0, "S Parameters"=[-0.344377489331-0.906562081765i, 0.186516030489-0.0753142645009i, 0.186351465404-0.0754228182721i, -0.380101755493-0.891271325629i]}, {"Frequency"=1216648187.5, "S Parameters"=[-0.351681346781-0.903744212944i, 0.186404120225-0.0771137642948i, 0.186229537476-0.0771956508478i, -0.387626723951-0.887778602011i]}, {"Frequency"=1221960625.0, "S Parameters"=[-0.35893878944-0.900559319674i, 0.1862653006-0.078885107735i, 0.186069203786-0.078921708408i, -0.395021580098-0.884369491087i]}, {"Frequency"=1227273062.5, "S Parameters"=[-0.366231826432-0.897397621332i, 0.186124101399-0.0806983585234i, 0.185894575472-0.0806711106029i, -0.40245580164-0.880732884259i]}, {"Frequency"=1232585500.0, "S Parameters"=[-0.37348926647-0.894156750998i, 0.185937105463-0.0824833112907i, 0.185670312652-0.0823971011374i, -0.409706664202-0.877117743407i]}, {"Frequency"=1237897937.5, "S Parameters"=[-0.380921309838-0.890793676613i, 0.185754580769-0.0843116351714i, 0.185455930729-0.0841851985815i, -0.417191688069-0.873356838645i]}, {"Frequency"=1243210375.0, "S Parameters"=[-0.38805687314-0.887504479799i, 0.185568707648-0.0860931635351i, 0.185232718951-0.0859275203019i, -0.424522338524-0.869547622111i]}, {"Frequency"=1248522812.5, "S Parameters"=[-0.395279766413-0.884247285274i, 0.185355017297-0.0878671349441i, 0.185010522445-0.0876910171962i, -0.431593295878-0.86583423286i]}, {"Frequency"=1253835250.0, "S Parameters"=[-0.40237003206-0.880689830187i, 0.185119954767-0.0895877450197i, 0.184793426154-0.0894230102492i, -0.438685924628-0.862047127031i]}, {"Frequency"=1259147687.5, "S Parameters"=[-0.40963000602-0.877075031994i, 0.184823635088-0.0913639836105i, 0.184521591693-0.0911672851262i, -0.445786059124-0.858108679916i]}, {"Frequency"=1264460125.0, "S Parameters"=[-0.416760936454-0.873273107918i, 0.184512084445-0.093146495255i, 0.184278639204-0.0929541724264i, -0.452679801834-0.854117458969i]}, {"Frequency"=1269772562.5, "S Parameters"=[-0.424235225776-0.869628820326i, 0.184164425383-0.0949241408868i, 0.184003430671-0.0947002064333i, -0.45968435116-0.850257155117i]}, {"Frequency"=1275085000.0, "S Parameters"=[-0.431465420483-0.865670710202i, 0.183800801403-0.0967131941666i, 0.183722308854-0.0964925399612i, -0.466772712905-0.846327310339i]}, {"Frequency"=1280397437.5, "S Parameters"=[-0.438745804713-0.861969432331i, 0.183439249649-0.0984999178918i, 0.183426476567-0.0982699380398i, -0.473651023068-0.842404523371i]}, {"Frequency"=1285709875.0, "S Parameters"=[-0.445978981909-0.85805907789i, 0.183032917729-0.100281727189i, 0.183067107115-0.100070346488i, -0.48044390275-0.838446592255i]}, {"Frequency"=1291022312.5, "S Parameters"=[-0.453060197564-0.854151303388i, 0.182634881234-0.102085637315i, 0.182715357598-0.101801955601i, -0.487149010904-0.834376594669i]}, {"Frequency"=1296334750.0, "S Parameters"=[-0.460172021543-0.850138479278i, 0.182194277659-0.103821864335i, 0.182328099234-0.103575552808i, -0.493733321669-0.830245043476i]}, {"Frequency"=1301647187.5, "S Parameters"=[-0.467271060797-0.846062257303i, 0.181752950068-0.105559530513i, 0.181886814389-0.105299909781i, -0.500298089329-0.826029006145i]}, {"Frequency"=1306959625.0, "S Parameters"=[-0.47421195208-0.841983836006i, 0.181276735405-0.107318320699i, 0.181418726464-0.107062246878i, -0.507054705592-0.821601424621i]}, {"Frequency"=1312272062.5, "S Parameters"=[-0.481015790942-0.837866103426i, 0.180783070961-0.109048968336i, 0.180945113621-0.108855683414i, -0.513626129586-0.817264161573i]}, {"Frequency"=1317584500.0, "S Parameters"=[-0.487930573326-0.833614890603i, 0.180255645944-0.110788206501i, 0.180373188904-0.11065038382i, -0.520194417178-0.812892877706i]}, {"Frequency"=1322896937.5, "S Parameters"=[-0.494775071372-0.82921625512i, 0.179732274639-0.112541662873i, 0.179767313546-0.112488517928i, -0.52676047493-0.808238640844i]}, {"Frequency"=1328209375.0, "S Parameters"=[-0.501603595576-0.825072679811i, 0.179178341415-0.114300122436i, 0.179201588812-0.114301561051i, -0.5334327775-0.803517221753i]}, {"Frequency"=1333521812.5, "S Parameters"=[-0.508313159371-0.820839571625i, 0.178617100533-0.116057104899i, 0.178629078432-0.116120504323i, -0.540098772841-0.798830503114i]}, {"Frequency"=1338834250.0, "S Parameters"=[-0.51480699753-0.816538017258i, 0.17804740543-0.117774936492i, 0.178033743372-0.117892542883i, -0.546659694321-0.794231333512i]}, {"Frequency"=1344146687.5, "S Parameters"=[-0.52132230033-0.812240631966i, 0.177482465208-0.119461458284i, 0.177425408735-0.119625579272i, -0.553063799052-0.78935089492i]}, {"Frequency"=1349459125.0, "S Parameters"=[-0.527619046441-0.807846947732i, 0.176884837794-0.121122956131i, 0.176853085806-0.121338390931i, -0.559467280262-0.784708194233i]}, {"Frequency"=1354771562.5, "S Parameters"=[-0.53399569692-0.80348504912i, 0.176274613593-0.122764127419i, 0.176244396661-0.122958774872i, -0.565764191309-0.779835348785i]}, {"Frequency"=1360084000.0, "S Parameters"=[-0.540292352547-0.799026921216i, 0.175668508388-0.124446412274i, 0.175648354353-0.124616149871i, -0.572113502418-0.775213967437i]}, {"Frequency"=1365396437.5, "S Parameters"=[-0.546572839127-0.7945960518i, 0.17504647593-0.126085999614i, 0.175054485261-0.126194230621i, -0.578476524535-0.770327394807i]}, {"Frequency"=1370708875.0, "S Parameters"=[-0.552833506558-0.790197389188i, 0.174384218204-0.12777726607i, 0.174413756171-0.127817109688i, -0.584668268487-0.76562656605i]}, {"Frequency"=1376021312.5, "S Parameters"=[-0.558996429641-0.785766512304i, 0.173733037938-0.129436629976i, 0.173747788495-0.129429862139i, -0.590819406954-0.760651904539i]}, {"Frequency"=1381333750.0, "S Parameters"=[-0.565093728119-0.781044633171i, 0.173040081602-0.131109256574i, 0.173086637344-0.131036113818i, -0.596855778687-0.755789190304i]}, {"Frequency"=1386646187.5, "S Parameters"=[-0.571244684912-0.776516418137i, 0.172362244546-0.132787549356i, 0.172395954648-0.132670743472i, -0.602870498265-0.75067318267i]}, {"Frequency"=1391958625.0, "S Parameters"=[-0.577257897364-0.771820183119i, 0.171653512245-0.134451049662i, 0.171718382268-0.13431063908i, -0.608913092267-0.745633843351i]}, {"Frequency"=1397271062.5, "S Parameters"=[-0.583196947891-0.767113463081i, 0.170935807545-0.136134454169i, 0.170978592825-0.135918416516i, -0.61494128952-0.740440806028i]}, {"Frequency"=1402583500.0, "S Parameters"=[-0.589004380507-0.76246928701i, 0.170209602758-0.13781693077i, 0.170250769787-0.137563123394i, -0.62075752102-0.73510981167i]}, {"Frequency"=1407895937.5, "S Parameters"=[-0.594902598895-0.757624991948i, 0.16943461603-0.139424632441i, 0.169495429047-0.139249210341i, -0.626675639475-0.729898097293i]}, {"Frequency"=1413208375.0, "S Parameters"=[-0.600851292858-0.752653499798i, 0.168653952477-0.141123437052i, 0.168688282615-0.140981645257i, -0.632632187156-0.724358859929i]}, {"Frequency"=1418520812.5, "S Parameters"=[-0.60670439877-0.747705480044i, 0.16783471398-0.142815339444i, 0.16789748829-0.142753154156i, -0.638476012355-0.718903271304i]}, {"Frequency"=1423833250.0, "S Parameters"=[-0.612530611194-0.742713476536i, 0.167037327555-0.144508253004i, 0.167074108807-0.144519047161i, -0.644421560985-0.713353674723i]}, {"Frequency"=1429145687.5, "S Parameters"=[-0.618309458885-0.737540647977i, 0.166177963329-0.146202768199i, 0.166239098996-0.146245918058i, -0.650258641864-0.70774085542i]}, {"Frequency"=1434458125.0, "S Parameters"=[-0.623959831002-0.73250110765i, 0.165346404874-0.147887499937i, 0.165386180974-0.147997953653i, -0.656025412437-0.70221046072i]}, {"Frequency"=1439770562.5, "S Parameters"=[-0.629797170625-0.727303121944i, 0.164489799587-0.149562599747i, 0.164523499353-0.149717702713i, -0.661690960132-0.696537348294i]}, {"Frequency"=1445083000.0, "S Parameters"=[-0.635498892784-0.722124864455i, 0.163580897641-0.151197487555i, 0.163646055958-0.151405346872i, -0.667383566886-0.691018895147i]}, {"Frequency"=1450395437.5, "S Parameters"=[-0.641195274328-0.716825327786i, 0.162659006902-0.152765751514i, 0.162768605427-0.152998841544i, -0.672941441109-0.685320702569i]}, {"Frequency"=1455707875.0, "S Parameters"=[-0.64679428973-0.711450476277i, 0.161757836314-0.154400174063i, 0.161841575274-0.154567373352i, -0.678505967575-0.679760084158i]}, {"Frequency"=1461020312.5, "S Parameters"=[-0.652566188608-0.706179564649i, 0.160798174511-0.155989161256i, 0.160885490646-0.156095841345i, -0.683908324213-0.674123019363i]}, {"Frequency"=1466332750.0, "S Parameters"=[-0.65807960988-0.700579696492i, 0.159823232026-0.15760012031i, 0.159863124854-0.15764271261i, -0.689265053837-0.668602240146i]}, {"Frequency"=1471645187.5, "S Parameters"=[-0.66379991479-0.695054784956i, 0.158804894989-0.159212319338i, 0.158835478545-0.159179456592i, -0.694519360333-0.662950456966i]}, {"Frequency"=1476957625.0, "S Parameters"=[-0.6694048882-0.689471405366i, 0.157800070312-0.160799826209i, 0.15778858643-0.160733689428i, -0.699640450558-0.657006804387i]}, {"Frequency"=1482270062.5, "S Parameters"=[-0.674990884635-0.683776999416i, 0.156761110553-0.162390365574i, 0.156705052313-0.162238540549i, -0.704885358665-0.651295667668i]}, {"Frequency"=1487582500.0, "S Parameters"=[-0.680529009434-0.678053108732i, 0.155700251175-0.163946430988i, 0.15567528752-0.163760153528i, -0.709913457916-0.645428528354i]}, {"Frequency"=1492894937.5, "S Parameters"=[-0.685961777492-0.672300992084i, 0.154617775389-0.165530224975i, 0.154562354478-0.165323314899i, -0.714937588939-0.639580745423i]}, {"Frequency"=1498207375.0, "S Parameters"=[-0.691287309283-0.666561458518i, 0.153555067689-0.167099422991i, 0.153481667045-0.166868996571i, -0.719998558489-0.633592951848i]}, {"Frequency"=1503519812.5, "S Parameters"=[-0.696705538784-0.660667244236i, 0.152439816847-0.168622200746i, 0.152404999104-0.16839205995i, -0.724953735908-0.627539686515i]}, {"Frequency"=1508832250.0, "S Parameters"=[-0.70202997644-0.654988625556i, 0.151348252496-0.170177303764i, 0.151326090904-0.169966314417i, -0.729998983437-0.621328708196i]}, {"Frequency"=1514144687.5, "S Parameters"=[-0.7072562977-0.649123877807i, 0.150186379283-0.171745327i, 0.15020834471-0.171557704694i, -0.735088754238-0.61507541087i]}, {"Frequency"=1519457125.0, "S Parameters"=[-0.712393508855-0.643258562635i, 0.148989191647-0.173300899891i, 0.149032204112-0.173138082407i, -0.740154872329-0.608627143605i]}, {"Frequency"=1524769562.5, "S Parameters"=[-0.717391757356-0.637272605891i, 0.147744496198-0.174813932903i, 0.147874819901-0.174660095024i, -0.745137460482-0.602205150853i]}, {"Frequency"=1530082000.0, "S Parameters"=[-0.722407093297-0.631373145921i, 0.146462196421-0.17631654849i, 0.146688194159-0.176196672808i, -0.750108054201-0.59561047901i]}, {"Frequency"=1535394437.5, "S Parameters"=[-0.727165558984-0.625381171789i, 0.145200046703-0.177797518942i, 0.145451292167-0.177666397519i, -0.755244203596-0.58904538455i]}, {"Frequency"=1540706875.0, "S Parameters"=[-0.73200490707-0.619788800781i, 0.143960047312-0.179239113356i, 0.144261632977-0.179088450815i, -0.760173582903-0.582415612387i]}, {"Frequency"=1546019312.5, "S Parameters"=[-0.736717927138-0.614056547397i, 0.142713206996-0.180610519234i, 0.143027344143-0.180503923424i, -0.765020162505-0.575896343394i]}, {"Frequency"=1551331750.0, "S Parameters"=[-0.741219732982-0.608320470377i, 0.141432823548-0.181979655874i, 0.141797266871-0.181817637775i, -0.769727000405-0.569345742783i]}, {"Frequency"=1556644187.5, "S Parameters"=[-0.745678107568-0.602733149406i, 0.140135775762-0.183308746277i, 0.140551168167-0.18318355437i, -0.774433398491-0.562641548562i]}, {"Frequency"=1561956625.0, "S Parameters"=[-0.750170529737-0.596917422313i, 0.138855099876-0.184644376138i, 0.13923283364-0.184530035565i, -0.778864377871-0.556075035965i]}, {"Frequency"=1567269062.5, "S Parameters"=[-0.754537892404-0.59113133679i, 0.137527141915-0.185973459897i, 0.137902004519-0.185852197413i, -0.783461775684-0.549434632561i]}, {"Frequency"=1572581500.0, "S Parameters"=[-0.758873974481-0.585386027947i, 0.136243801166-0.187312828746i, 0.136587593901-0.18718559321i, -0.787814789585-0.542913094443i]}, {"Frequency"=1577893937.5, "S Parameters"=[-0.763101698937-0.579514197821i, 0.134927981168-0.188669734934i, 0.135247668393-0.188548032819i, -0.792185005477-0.536284649616i]}, {"Frequency"=1583206375.0, "S Parameters"=[-0.767329547864-0.573687043728i, 0.133581875402-0.189962495684i, 0.13391599059-0.189866483468i, -0.796423246623-0.529686754686i]}, {"Frequency"=1588518812.5, "S Parameters"=[-0.771652692625-0.567708353014i, 0.132292342955-0.191277640838i, 0.132573990315-0.191231572781i, -0.800666633769-0.523058801586i]}, {"Frequency"=1593831250.0, "S Parameters"=[-0.775858688381-0.561724305154i, 0.130972893774-0.192644175414i, 0.131240752266-0.192612164672i, -0.804767333351-0.516373707421i]}, {"Frequency"=1599143687.5, "S Parameters"=[-0.780075100076-0.55572890889i, 0.129688685048-0.193911801667i, 0.129960525865-0.193940835452i, -0.808809227693-0.509832813518i]}, {"Frequency"=1604456125.0, "S Parameters"=[-0.784233379536-0.549679850891i, 0.128393691882-0.195229980995i, 0.128631214655-0.195241278381i, -0.812821353323-0.503296180657i]}, {"Frequency"=1609768562.5, "S Parameters"=[-0.788333685693-0.543394659055i, 0.127005103086-0.196493937275i, 0.127281663986-0.196532163481i, -0.816633621081-0.496583160223i]}, {"Frequency"=1615081000.0, "S Parameters"=[-0.7924502322-0.537054960022i, 0.125612340762-0.19781057544i, 0.12591899386-0.197815760116i, -0.820451769813-0.489716143635i]}, {"Frequency"=1620393437.5, "S Parameters"=[-0.796546373599-0.530618450235i, 0.124171930727-0.199137120784i, 0.124485787752-0.199098493216i, -0.824469450161-0.48283558273i]}, {"Frequency"=1625705875.0, "S Parameters"=[-0.800509534559-0.524116223043i, 0.12271723714-0.200416196758i, 0.123041529675-0.200358815672i, -0.828104370906-0.475951282305i]}, {"Frequency"=1631018312.5, "S Parameters"=[-0.804586248686-0.517570516664i, 0.121306660781-0.201700388043i, 0.121564036638-0.20160510559i, -0.831879645866-0.469200622571i]}, {"Frequency"=1636330750.0, "S Parameters"=[-0.808558502159-0.511020943718i, 0.119844958703-0.202936865262i, 0.120110591676-0.202838403271i, -0.835578491371-0.462409726403i]}, {"Frequency"=1641643187.5, "S Parameters"=[-0.81255901956-0.504320188087i, 0.118355840741-0.20416160722i, 0.118618560709-0.204021890974i, -0.839235168273-0.455629608131i]}, {"Frequency"=1646955625.0, "S Parameters"=[-0.816420312178-0.497681779347i, 0.116849491793-0.205371632857i, 0.117091985118-0.205196162587i, -0.842693086503-0.448749812815i]}, {"Frequency"=1652268062.5, "S Parameters"=[-0.820254939626-0.491100382505i, 0.115364771666-0.206519589258i, 0.115648879433-0.206344102137i, -0.846134075648-0.442091228179i]}, {"Frequency"=1657580500.0, "S Parameters"=[-0.824079217224-0.484336210841i, 0.113859123756-0.20767055969i, 0.114134194336-0.207508651557i, -0.849486694699-0.435279879619i]}, {"Frequency"=1662892937.5, "S Parameters"=[-0.827845353532-0.477770683878i, 0.112377795669-0.208813758068i, 0.112655887179-0.20866298377i, -0.852793253158-0.428644218416i]}, {"Frequency"=1668205375.0, "S Parameters"=[-0.831603096174-0.470925226688i, 0.110795698093-0.209947204711i, 0.11111201248-0.209812745899i, -0.856036358481-0.421828839083i]}, {"Frequency"=1673517812.5, "S Parameters"=[-0.835296912945-0.464049135976i, 0.109254019542-0.211082771906i, 0.109577357876-0.210984991625i, -0.859130689184-0.415131366841i]}, {"Frequency"=1678830250.0, "S Parameters"=[-0.838983257056-0.457165927485i, 0.10769697355-0.21217318369i, 0.108046525251-0.212169748408i, -0.862226602-0.408345551335i]}, {"Frequency"=1684142687.5, "S Parameters"=[-0.842565343429-0.450227312259i, 0.106128294201-0.213307651306i, 0.106540447107-0.213309951939i, -0.865327249871-0.401534156431i]}, {"Frequency"=1689455125.0, "S Parameters"=[-0.846159449847-0.443317304794i, 0.104636216627-0.214426782436i, 0.105032852378-0.214449156231i, -0.86834819179-0.3947653936i]}, {"Frequency"=1694767562.5, "S Parameters"=[-0.849590269728-0.436500798753i, 0.103115323106-0.215510796731i, 0.103514257338-0.215542720894i, -0.871276206628-0.387976239857i]}, {"Frequency"=1700080000.0, "S Parameters"=[-0.852996200014-0.429642739968i, 0.101534781236-0.2165624753i, 0.101979294585-0.216629167123i, -0.874110055786-0.381109125435i]}, {"Frequency"=1705392437.5, "S Parameters"=[-0.85640183511-0.422814352264i, 0.0999225300463-0.217612528414i, 0.100375438687-0.21767180411i, -0.876897233491-0.374091442284i]}, {"Frequency"=1710704875.0, "S Parameters"=[-0.859471027111-0.415890890879i, 0.0983218058728-0.218676887306i, 0.0987562039159-0.218672357863i, -0.879681889471-0.367079352845i]}, {"Frequency"=1716017312.5, "S Parameters"=[-0.862585222199-0.408913872016i, 0.0967019815475-0.219705974018i, 0.0971052471411-0.2196599297i, -0.882357021178-0.360080324992i]}, {"Frequency"=1721329750.0, "S Parameters"=[-0.865727654475-0.402038747068i, 0.0950522093109-0.22072923585i, 0.0954319804688-0.22065990265i, -0.88497911145-0.352851022689i]}, {"Frequency"=1726642187.5, "S Parameters"=[-0.868632367524-0.395094120055i, 0.093355908422-0.221720077185i, 0.0936832810444-0.221590758427i, -0.887758791721-0.345518257264i]}, {"Frequency"=1731954625.0, "S Parameters"=[-0.871675270172-0.388343699003i, 0.0916633260916-0.22269902134i, 0.0919683923425-0.222517684707i, -0.890396285996-0.338115896542i]}, {"Frequency"=1737267062.5, "S Parameters"=[-0.874564777798-0.381446212285i, 0.0899860455924-0.223636608075i, 0.0902284397957-0.223434505734i, -0.893018323413-0.330775242898i]}, {"Frequency"=1742579500.0, "S Parameters"=[-0.877371752145-0.374675517046i, 0.088310290044-0.224538581542i, 0.088512679822-0.224344364701i, -0.89554436464-0.323421931525i]}, {"Frequency"=1747891937.5, "S Parameters"=[-0.88008347742-0.367987712214i, 0.0865473971666-0.225468807873i, 0.0868126513463-0.225192639316i, -0.898145536231-0.316173413569i]}, {"Frequency"=1753204375.0, "S Parameters"=[-0.882711374262-0.361502604622i, 0.0849062537181-0.226331571338i, 0.0851422656713-0.226053263945i, -0.900477570276-0.308848330914i]}, {"Frequency"=1758516812.5, "S Parameters"=[-0.885280956689-0.354838410864i, 0.0832215674014-0.227204173043i, 0.0834639875591-0.226913360186i, -0.902839310881-0.301586121441i]}, {"Frequency"=1763829250.0, "S Parameters"=[-0.887798198288-0.348223791384i, 0.0814847396466-0.228043376419i, 0.0818032613599-0.227764661785i, -0.905150693928-0.294078097343i]}, {"Frequency"=1769141687.5, "S Parameters"=[-0.890287146952-0.341618052686i, 0.0797443136348-0.228906399774i, 0.0801256458906-0.228624212543i, -0.907444414712-0.286613732649i]}, {"Frequency"=1774454125.0, "S Parameters"=[-0.892740031547-0.33484822677i, 0.0780518872629-0.22972440202i, 0.0785071338826-0.229503614739i, -0.909547320243-0.279193236088i]}, {"Frequency"=1779766562.5, "S Parameters"=[-0.895051992819-0.328172071539i, 0.0763660416604-0.230602782659i, 0.0768880964948-0.230336398754i, -0.911724317811-0.271744804995i]}, {"Frequency"=1785079000.0, "S Parameters"=[-0.897387454966-0.321463465138i, 0.0746421230506-0.231433187227i, 0.0752725056224-0.231165567008i, -0.913694511007-0.264277913494i]}, {"Frequency"=1790391437.5, "S Parameters"=[-0.89972177071-0.314646425689i, 0.0729281344668-0.232256531126i, 0.073577248399-0.232021246038i, -0.915669031713-0.256789789368i]}, {"Frequency"=1795703875.0, "S Parameters"=[-0.901880767445-0.30781290928i, 0.0711789925563-0.233074251558i, 0.071874095598-0.232809561688i, -0.917575737915-0.249371198147i]}, {"Frequency"=1801016312.5, "S Parameters"=[-0.903991451117-0.301108256146i, 0.069471882557-0.233835069382i, 0.0702153795293-0.233626396826i, -0.919331698489-0.241983474266i]}, {"Frequency"=1806328750.0, "S Parameters"=[-0.906047639273-0.294166083607i, 0.0677541122998-0.234634211266i, 0.0684870252365-0.234376298317i, -0.920987718547-0.23454046735i]}, {"Frequency"=1811641187.5, "S Parameters"=[-0.908148184116-0.28719741958i, 0.0659858211205-0.235396903251i, 0.0667239707027-0.235138476774i, -0.922718607814-0.227033090912i]}, {"Frequency"=1816953625.0, "S Parameters"=[-0.910074077852-0.280017002426i, 0.0641838656073-0.236128152462i, 0.0648509910006-0.235908494332i, -0.924260619724-0.219500274183i]}, {"Frequency"=1822266062.5, "S Parameters"=[-0.912106795256-0.272759429227i, 0.0623297390759-0.236887562254i, 0.0630036432985-0.23665730604i, -0.926016540255-0.211835263214i]}, {"Frequency"=1827578500.0, "S Parameters"=[-0.91413019479-0.265447816329i, 0.0604901276334-0.237610871459i, 0.0610994509695-0.237412638132i, -0.927607028927-0.204285855025i]}, {"Frequency"=1832890937.5, "S Parameters"=[-0.916092362566-0.258156512189i, 0.0586206779619-0.238329455099i, 0.059198748592-0.238129155307i, -0.929199848406-0.196609397386i]}, {"Frequency"=1838203375.0, "S Parameters"=[-0.918020930161-0.250750311281i, 0.0567275990624-0.239010407955i, 0.0572807454886-0.238803159993i, -0.930782283392-0.189153207529i]}, {"Frequency"=1843515812.5, "S Parameters"=[-0.919879059819-0.243367779206i, 0.0548698874198-0.239677973842i, 0.0554203471985-0.239480008903i, -0.932257936782-0.181587684438i]}, {"Frequency"=1848828250.0, "S Parameters"=[-0.921682450689-0.235925758201i, 0.0529697003705-0.240264281835i, 0.0535109909771-0.240138030582i, -0.933548419215-0.173985131214i]}, {"Frequency"=1854140687.5, "S Parameters"=[-0.92350580052-0.228572531352i, 0.0510854068463-0.240850975443i, 0.0516498738345-0.240697978335i, -0.93485153732-0.166561596206i]}, {"Frequency"=1859453125.0, "S Parameters"=[-0.925148834619-0.221274980999i, 0.0491914056608-0.241438200632i, 0.0497926624211-0.241278267985i, -0.936121987227-0.159116570877i]}, {"Frequency"=1864765562.5, "S Parameters"=[-0.926775127925-0.213751028374i, 0.0473371544918-0.241946298008i, 0.0479381921599-0.241818881502i, -0.937278586376-0.151697418688i]}, {"Frequency"=1870078000.0, "S Parameters"=[-0.928507317065-0.206168905911i, 0.0454203409628-0.242428279494i, 0.0460838023878-0.242342860752i, -0.938289946583-0.144228789188i]}, {"Frequency"=1875390437.5, "S Parameters"=[-0.929995355471-0.198702010565i, 0.0435487935651-0.242911878133i, 0.0442409392482-0.242815886186i, -0.939343087667-0.136827915451i]}, {"Frequency"=1880702875.0, "S Parameters"=[-0.93142468063-0.191358865011i, 0.0416326742196-0.243393146034i, 0.0424256877506-0.243239782006i, -0.940201798661-0.12946595862i]}, {"Frequency"=1886015312.5, "S Parameters"=[-0.932984624704-0.183791626641i, 0.03976604058-0.243823822821i, 0.0405588600171-0.243704351964i, -0.94126124719-0.121991870196i]}, {"Frequency"=1891327750.0, "S Parameters"=[-0.93428893768-0.176367077654i, 0.0378994468387-0.244291476152i, 0.0387242190444-0.244151882159i, -0.941994162302-0.11482644961i]}, {"Frequency"=1896640187.5, "S Parameters"=[-0.935407297722-0.16892009577i, 0.0361104361457-0.244719393861i, 0.0368996364639-0.244508979092i, -0.942630499157-0.107670121255i]}, {"Frequency"=1901952625.0, "S Parameters"=[-0.936582048829-0.161639972161i, 0.0342648626303-0.245091767662i, 0.0350653504763-0.24487432065i, -0.943204830908-0.100362147965i]}, {"Frequency"=1907265062.5, "S Parameters"=[-0.937691132469-0.154210399756i, 0.0324322995417-0.245475344314i, 0.0332194311936-0.245262015438i, -0.943712746738-0.0931102819837i]}, {"Frequency"=1912577500.0, "S Parameters"=[-0.938771208673-0.146794253282i, 0.030581008472-0.245857623078i, 0.0313134012255-0.245666941686i, -0.944374740193-0.0857055186915i]}, {"Frequency"=1917889937.5, "S Parameters"=[-0.939830381907-0.13944846405i, 0.0286755976581-0.246230817184i, 0.0293933102474-0.246028198912i, -0.944951895089-0.0783306638949i]}, {"Frequency"=1923202375.0, "S Parameters"=[-0.940848724402-0.132026701257i, 0.0267472076707-0.246604988769i, 0.0274706500113-0.246385240283i, -0.945524375779-0.0708222045938i]}, {"Frequency"=1928514812.5, "S Parameters"=[-0.941891621194-0.124755327229i, 0.0248286238844-0.246965498487i, 0.0255076029565-0.246788810641i, -0.946093357447-0.0633640271318i]}, {"Frequency"=1933827250.0, "S Parameters"=[-0.942715513235-0.117417359975i, 0.0229009334403-0.247330386681i, 0.0235698093421-0.247143648711i, -0.946356001177-0.055831703701i]}, {"Frequency"=1939139687.5, "S Parameters"=[-0.943526202436-0.110178487099i, 0.0209509805235-0.24762706834i, 0.0216047634367-0.24750593106i, -0.946692607181-0.0482098698813i]}, {"Frequency"=1944452125.0, "S Parameters"=[-0.944358525052-0.103027844524i, 0.0190332547126-0.247927853798i, 0.0196689830345-0.24782981762i, -0.947005160837-0.0406104025464i]}, {"Frequency"=1949764562.5, "S Parameters"=[-0.945103508841-0.0961195448046i, 0.017130582281-0.248194829206i, 0.0177819599644-0.248090268004i, -0.947281099263-0.033119369168i]}, {"Frequency"=1955077000.0, "S Parameters"=[-0.945658429885-0.0891354734119i, 0.0152358375287-0.248418287456i, 0.0158970664925-0.248327342037i, -0.947440057878-0.0256605511127i]}, {"Frequency"=1960389437.5, "S Parameters"=[-0.946240083247-0.0820038758641i, 0.0133295704583-0.248609188433i, 0.0140120291248-0.248554535471i, -0.947419868755-0.0181263330309i]}, {"Frequency"=1965701875.0, "S Parameters"=[-0.946789543377-0.0749617183656i, 0.0114274206065-0.248782390828i, 0.012102664567-0.248679411399i, -0.947356684067-0.0105402392678i]}, {"Frequency"=1971014312.5, "S Parameters"=[-0.947262895625-0.0680396875416i, 0.00955071649532-0.248956646394i, 0.0102415800258-0.248823334306i, -0.947422441857-0.00306102600926i]}, {"Frequency"=1976326750.0, "S Parameters"=[-0.947523717999-0.0610214662626i, 0.00766057025508-0.249134116075i, 0.00834305524689-0.248955494611i, -0.947171068434+0.00435378457907i]}, {"Frequency"=1981639187.5, "S Parameters"=[-0.947813784009-0.0539290650295i, 0.0058058293127-0.249277242384i, 0.00649202852103-0.249050752314i, -0.946896722271+0.0115566334556i]}, {"Frequency"=1986951625.0, "S Parameters"=[-0.947891252491-0.0468103565773i, 0.00398624313645-0.24942677305i, 0.00461694394321-0.249141807605i, -0.946585195307+0.0188110795858i]}, {"Frequency"=1992264062.5, "S Parameters"=[-0.948188516087-0.0397611048835i, 0.0021494465482-0.249534093711i, 0.00276671682482-0.249239415912i, -0.946253386534+0.026131650018i]}, {"Frequency"=1997576500.0, "S Parameters"=[-0.948191192152-0.0325731012259i, 0.000335236162813-0.249677094319i, 0.000941687043056-0.249366653586i, -0.94586162976+0.0332109496928i]}, {"Frequency"=2002888937.5, "S Parameters"=[-0.94839777785-0.0254174600818i, -0.00152105685869-0.249819850446i, -0.000887125704363-0.249501070701i, -0.94559509056+0.0403349234486i]}, {"Frequency"=2008201375.0, "S Parameters"=[-0.948437962892-0.0181408412764i, -0.00333239316688-0.249987893814i, -0.00272442150402-0.249613506483i, -0.945256375346+0.0474799009667i]}, {"Frequency"=2013513812.5, "S Parameters"=[-0.948588458597-0.0109092618979i, -0.00522854493993-0.250135874517i, -0.00455829111822-0.249764424683i, -0.944907230005+0.05463440513i]}, {"Frequency"=2018826250.0, "S Parameters"=[-0.948589929421-0.00353541792833i, -0.00721467048416-0.250242724423i, -0.00647842387625-0.249853523667i, -0.944545610147+0.0617638374486i]}, {"Frequency"=2024138687.5, "S Parameters"=[-0.948514037909+0.00393910044833i, -0.0091516123707-0.25034383646i, -0.00841019415373-0.249950510505i, -0.944055099632+0.0691012735074i]}, {"Frequency"=2029451125.0, "S Parameters"=[-0.948488793468+0.0114806814349i, -0.0111187733253-0.250394182384i, -0.0103303086273-0.250009461509i, -0.943337273691+0.0763724302754i]}, {"Frequency"=2034763562.5, "S Parameters"=[-0.948456090427+0.0188453899983i, -0.013109141028-0.25046067171i, -0.0122340241327-0.250040750663i, -0.942776499891+0.0837475690384i]}, {"Frequency"=2040076000.0, "S Parameters"=[-0.948105893506+0.0260613240234i, -0.0150404578667-0.250502505429i, -0.014171056949-0.250112602777i, -0.942041394835+0.0910055332484i]}, {"Frequency"=2045388437.5, "S Parameters"=[-0.947727562159+0.0334550583039i, -0.0170104523755-0.250524430339i, -0.0160522835601-0.250123304739i, -0.94117151982+0.0983392415451i]}, {"Frequency"=2050700875.0, "S Parameters"=[-0.947428926141+0.0407105760358i, -0.0188779067769-0.250479935472i, -0.0179554631396-0.250078176099i, -0.94023313241+0.10551152112i]}, {"Frequency"=2056013312.5, "S Parameters"=[-0.947059121995+0.048035520439i, -0.0208020107571-0.250401393124i, -0.0198852683502-0.250030111865i, -0.939222148139+0.112678871068i]}, {"Frequency"=2061325750.0, "S Parameters"=[-0.946571008213+0.0552271817511i, -0.022708762762-0.250324433229i, -0.021836532598-0.249969123899i, -0.938229741728+0.120014324402i]}, {"Frequency"=2066638187.5, "S Parameters"=[-0.946126780125+0.0625566961645i, -0.0246433670464-0.250234314163i, -0.0237727769488-0.249906090609i, -0.937083292973+0.127387555971i]}, {"Frequency"=2071950625.0, "S Parameters"=[-0.945225760149+0.069755459509i, -0.0265621584162-0.250095645362i, -0.0257443601723-0.249804950301i, -0.935862859047+0.134594821151i]}, {"Frequency"=2077263062.5, "S Parameters"=[-0.944348659076+0.076972153884i, -0.0284697540754-0.249967780641i, -0.0276988267746-0.249673491846i, -0.934711753482+0.141806246045i]}, {"Frequency"=2082575500.0, "S Parameters"=[-0.94359363+0.0844193896083i, -0.0304093973066-0.249833796001i, -0.0296518975462-0.249539054016i, -0.93332595244+0.149136029526i]}, {"Frequency"=2087887937.5, "S Parameters"=[-0.9427477837+0.0918534428229i, -0.0323155200565-0.24962936327i, -0.031634513879-0.249399230228i, -0.932007402774+0.156427422235i]}, {"Frequency"=2093200375.0, "S Parameters"=[-0.941918550934+0.0993239003972i, -0.0342569601597-0.249493954989i, -0.033559923857-0.249199486067i, -0.930777321043+0.163725925475i]}, {"Frequency"=2098512812.5, "S Parameters"=[-0.941116029022+0.106637500094i, -0.0361963154431-0.249296753534i, -0.0355188078641-0.249032892124i, -0.929560986242+0.171110862715i]}, {"Frequency"=2103825250.0, "S Parameters"=[-0.940265261325+0.113970822473i, -0.0380704663985-0.249057251249i, -0.0374058796973-0.248754765843i, -0.928261055641+0.17824140362i]}, {"Frequency"=2109137687.5, "S Parameters"=[-0.939415687373+0.121131520553i, -0.04002402139-0.248830766474i, -0.039298764717-0.248497308609i, -0.926761113495+0.185394276194i]}, {"Frequency"=2114450125.0, "S Parameters"=[-0.93844041914+0.128580247818i, -0.041957858345-0.248527371598i, -0.0412239631304-0.248138545897i, -0.925312101187+0.192597340669i]}, {"Frequency"=2119762562.5, "S Parameters"=[-0.937477564365+0.135863344211i, -0.0439383532672-0.248188489891i, -0.0430797359236-0.247831887651i, -0.923758824542+0.199832448702i]}, {"Frequency"=2125075000.0, "S Parameters"=[-0.936352096992+0.143114122783i, -0.0458398312483-0.247898415834i, -0.0450046304245-0.247460404167i, -0.922161021613+0.207050944059i]}, {"Frequency"=2130387437.5, "S Parameters"=[-0.935151094212+0.150294179781i, -0.04771871813-0.247546226114i, -0.0468105737319-0.247098729179i, -0.920494989966+0.214178594991i]}, {"Frequency"=2135699875.0, "S Parameters"=[-0.934035741588+0.157439815691i, -0.0495606475351-0.247187217206i, -0.0485991713443-0.246765611092i, -0.918618023121+0.221366918761i]}, {"Frequency"=2141012312.5, "S Parameters"=[-0.93272733952+0.164565959223i, -0.0514067513923-0.246842723833i, -0.0504427148402-0.246380220638i, -0.916891294275+0.228311108484i]}, {"Frequency"=2146324750.0, "S Parameters"=[-0.931559975804+0.171556981034i, -0.0532145713017-0.246512072448i, -0.0522183830174-0.246035012479i, -0.915149125627+0.235422132352i]}, {"Frequency"=2151637187.5, "S Parameters"=[-0.930199078661+0.178420858136i, -0.0550175247193-0.246230097003i, -0.0540487738179-0.245706777431i, -0.913308350306+0.242297638222i]}, {"Frequency"=2156949625.0, "S Parameters"=[-0.928753093964+0.185261770982i, -0.0568431563632-0.245847722708i, -0.0558273287632-0.245421737357i, -0.911287741973+0.249395344108i]}, {"Frequency"=2162262062.5, "S Parameters"=[-0.927261876372+0.192054178018i, -0.0586459590493-0.245539363841i, -0.0576822535337-0.245052328538i, -0.909329348066+0.256378478867i]}, {"Frequency"=2167574500.0, "S Parameters"=[-0.925642651614+0.198899888799i, -0.0605153048902-0.245118761451i, -0.0595486296932-0.244659068041i, -0.90708865863+0.263574850685i]}, {"Frequency"=2172886937.5, "S Parameters"=[-0.924044506377+0.205745328196i, -0.0623905414967-0.244713300014i, -0.0614986891698-0.244307567714i, -0.904788550693+0.270646242109i]}, {"Frequency"=2178199375.0, "S Parameters"=[-0.922263428583+0.212670938554i, -0.0642685263753-0.244294149569i, -0.0634130671923-0.243908682646i, -0.902551693264+0.277726323192i]}, {"Frequency"=2183511812.5, "S Parameters"=[-0.92058832992+0.219404655516i, -0.0661455637224-0.243833748612i, -0.0652947082305-0.243499564411i, -0.900280869873+0.284966103323i]}, {"Frequency"=2188824250.0, "S Parameters"=[-0.91906630411+0.226272187182i, -0.0679730438402-0.243355275467i, -0.067164215435-0.24302697958i, -0.898061692055+0.292000141773i]}, {"Frequency"=2194136687.5, "S Parameters"=[-0.917387928987+0.232943773024i, -0.0698389039511-0.242860547819i, -0.0690806190743-0.24254898744i, -0.895812883107+0.298888535192i]}, {"Frequency"=2199449125.0, "S Parameters"=[-0.91557438181+0.239547059797i, -0.0716508887028-0.242333186035i, -0.0708887300085-0.242012220304i, -0.893580476059+0.305798273531i]}, {"Frequency"=2204761562.5, "S Parameters"=[-0.913930415766+0.246119938839i, -0.0734412034919-0.241786503128i, -0.0726910530913-0.24147405659i, -0.891058861668+0.312500341588i]}, {"Frequency"=2210074000.0, "S Parameters"=[-0.912075854431+0.252558570253i, -0.0752283076591-0.241282489706i, -0.074433441177-0.240903640868i, -0.888602930306+0.3192195563i]}, {"Frequency"=2215386437.5, "S Parameters"=[-0.910315944342+0.259105057997i, -0.0769647224501-0.240741908063i, -0.0762419125158-0.240307757085i, -0.886128236808+0.325877006579i]}, {"Frequency"=2220698875.0, "S Parameters"=[-0.908397581014+0.265677825133i, -0.0787569175061-0.240190635441i, -0.0780001382892-0.239745234157i, -0.883605052298+0.332668993186i]}, {"Frequency"=2226011312.5, "S Parameters"=[-0.906460202389+0.2722263756i, -0.0805223097083-0.239643197954i, -0.0798271114674-0.239118707351i, -0.880942577412+0.3394214603i]}, {"Frequency"=2231323750.0, "S Parameters"=[-0.904389474667+0.27891973176i, -0.0823141315007-0.239094854534i, -0.0816244920676-0.2385405546i, -0.878339008219+0.346143560958i]}, {"Frequency"=2236636187.5, "S Parameters"=[-0.902407877713+0.285527159369i, -0.0840848015626-0.238611826811i, -0.0834238262943-0.237957156703i, -0.875695923262+0.353042560207i]}, {"Frequency"=2241948625.0, "S Parameters"=[-0.900371066449+0.292244672179i, -0.0859016336265-0.238016624562i, -0.085254029114-0.237339912535i, -0.872912908685+0.35979986415i]}, {"Frequency"=2247261062.5, "S Parameters"=[-0.898038519854+0.298846512213i, -0.0876580693505-0.237406725921i, -0.0870529686355-0.236717300994i, -0.870158243499+0.366429806631i]}, {"Frequency"=2252573500.0, "S Parameters"=[-0.895807255907+0.305469689624i, -0.089430106017-0.23681968795i, -0.0888528839427-0.236107519236i, -0.867284599302+0.373157776183i]}, {"Frequency"=2257885937.5, "S Parameters"=[-0.893358298158+0.312388318193i, -0.0912768677515-0.236121824025i, -0.0906965090359-0.235445302734i, -0.86420210264+0.379990311223i]}, {"Frequency"=2263198375.0, "S Parameters"=[-0.890788396303+0.319175707918i, -0.0930672408215-0.235381673486i, -0.0924705424768-0.234744380064i, -0.860970340115+0.38683122044i]}, {"Frequency"=2268510812.5, "S Parameters"=[-0.888042370553+0.326105165857i, -0.0949089498509-0.234643673618i, -0.0942777184716-0.23400052878i, -0.857789640853+0.393651637191i]}, {"Frequency"=2273823250.0, "S Parameters"=[-0.885347304275+0.333060610134i, -0.0967170809852-0.233846954881i, -0.0960596964585-0.233222300881i, -0.854518573782+0.400397666689i]}, {"Frequency"=2279135687.5, "S Parameters"=[-0.882566983253+0.340200325388i, -0.0984933565595-0.233037673235i, -0.0978417541474-0.232392417838i, -0.851294433786+0.407064162795i]}, {"Frequency"=2284448125.0, "S Parameters"=[-0.87985891368+0.347040591393i, -0.100279593533-0.232249145879i, -0.0995362657638-0.231597259726i, -0.848243250703+0.413672323138i]}, {"Frequency"=2289760562.5, "S Parameters"=[-0.877006738196+0.353907971264i, -0.102013083352-0.231384162335i, -0.101280134769-0.230787341212i, -0.844897881117+0.420096573901i]}, {"Frequency"=2295073000.0, "S Parameters"=[-0.874325177101+0.360688924514i, -0.103768411173-0.230596138359i, -0.102968460605-0.229942368679i, -0.84172852573+0.426421014491i]}, {"Frequency"=2300385437.5, "S Parameters"=[-0.871654053488+0.367257917485i, -0.105379417404-0.229777453232i, -0.104666348199-0.229165644204i, -0.838464004231+0.432619049578i]}, {"Frequency"=2305697875.0, "S Parameters"=[-0.868971041345+0.373738910258i, -0.107036235181-0.228908335906i, -0.10629378014-0.228321228385i, -0.835257926602+0.438648181813i]}, {"Frequency"=2311010312.5, "S Parameters"=[-0.866094595967+0.380307739745i, -0.108741491947-0.228045891574i, -0.107947847678-0.227405407997i, -0.832063653962+0.444809621601i]}, {"Frequency"=2316322750.0, "S Parameters"=[-0.86330827645+0.386622614618i, -0.110358135324-0.227136087943i, -0.109630654946-0.226543435159i, -0.828725170199+0.450936917437i]}, {"Frequency"=2321635187.5, "S Parameters"=[-0.860484891779+0.393096113887i, -0.112035027608-0.226271813702i, -0.111295762372-0.225688910495i, -0.825405327199+0.457014078054i]}, {"Frequency"=2326947625.0, "S Parameters"=[-0.857683734929+0.399388642158i, -0.113648009198-0.225371831616i, -0.11293279544-0.224847701453i, -0.822063300735+0.463061016537i]}, {"Frequency"=2332260062.5, "S Parameters"=[-0.854796668496+0.405552256356i, -0.115237039593-0.224473748495i, -0.114576849284-0.223936174784i, -0.818628331794+0.469301476027i]}, {"Frequency"=2337572500.0, "S Parameters"=[-0.851656804174+0.411572896133i, -0.116833417887-0.22354185808i, -0.116153982514-0.223061182336i, -0.815146955768+0.475266185874i]}, {"Frequency"=2342884937.5, "S Parameters"=[-0.848842245524+0.417637463953i, -0.118456097592-0.222676522203i, -0.117768825372-0.222188760498i, -0.811499102714+0.481343565166i]}, {"Frequency"=2348197375.0, "S Parameters"=[-0.845702992075+0.423812458674i, -0.120018709674-0.22176840938i, -0.119389632723-0.221187947903i, -0.807810860756+0.487217512906i]}, {"Frequency"=2353509812.5, "S Parameters"=[-0.842786395806+0.429602489489i, -0.1215759003-0.22086868974i, -0.120977113812-0.220360602795i, -0.803930562888+0.493468362105i]}, {"Frequency"=2358822250.0, "S Parameters"=[-0.839536321531+0.435671052975i, -0.12320128288-0.219948842526i, -0.122522480362-0.219380244092i, -0.800159048293+0.499649198219i]}, {"Frequency"=2364134687.5, "S Parameters"=[-0.836321459624+0.441649961875i, -0.124755023564-0.218934106572i, -0.124053817709-0.218411076647i, -0.796098936338+0.505907860504i]}, {"Frequency"=2369447125.0, "S Parameters"=[-0.83308656907+0.447813919364i, -0.12632784732-0.217950825902i, -0.125648521867-0.217356250476i, -0.79221143519+0.511924572664i]}, {"Frequency"=2374759562.5, "S Parameters"=[-0.829838292475+0.453902151362i, -0.127926610871-0.216965994044i, -0.127212597238-0.216313143558i, -0.788315577639+0.518105063571i]}, {"Frequency"=2380072000.0, "S Parameters"=[-0.826597219924+0.459904607478i, -0.129534874959-0.215920598512i, -0.128780370787-0.215288932398i, -0.784294157896+0.524222861869i]}, {"Frequency"=2385384437.5, "S Parameters"=[-0.823200912877+0.465976040455i, -0.131053615424-0.214883609722i, -0.130323229279-0.214235582749i, -0.780242540205+0.530169015184i]}, {"Frequency"=2390696875.0, "S Parameters"=[-0.819770866163+0.47200059926i, -0.132630321651-0.2138397313i, -0.131878138804-0.213161120626i, -0.776139491085+0.536106974787i]}, {"Frequency"=2396009312.5, "S Parameters"=[-0.816308975251+0.477819234037i, -0.134102541828-0.212830865392i, -0.133378777426-0.21207866348i, -0.772061631+0.541965845065i]}, {"Frequency"=2401321750.0, "S Parameters"=[-0.812861507655+0.483729829901i, -0.135522346257-0.211793717714i, -0.134842959309-0.211023829559i, -0.767955154918+0.547559136118i]}, {"Frequency"=2406634187.5, "S Parameters"=[-0.80951091953+0.489468301285i, -0.137017776587-0.210743924497i, -0.136313181651-0.210035030491i, -0.763845741458+0.553259247244i]}, {"Frequency"=2411946625.0, "S Parameters"=[-0.805822395911+0.495435323552i, -0.138429988964-0.209685066704i, -0.137764269229-0.20894778774i, -0.759744547711+0.558946050043i]}, {"Frequency"=2417259062.5, "S Parameters"=[-0.802225734813+0.501080142453i, -0.139843438663-0.208610939565i, -0.139169605515-0.207932434465i, -0.755651512195+0.564624212307i]}, {"Frequency"=2422571500.0, "S Parameters"=[-0.798509125561+0.506920346574i, -0.141271779669-0.207522015766i, -0.140644856762-0.206868592983i, -0.751364513827+0.570186562352i]}, {"Frequency"=2427883937.5, "S Parameters"=[-0.794767956778+0.512740913348i, -0.14269785507-0.206438369797i, -0.142096866916-0.205786290855i, -0.747140736871+0.575619184038i]}, {"Frequency"=2433196375.0, "S Parameters"=[-0.790906042808+0.518345527319i, -0.14409242651-0.20532598532i, -0.143498276548-0.204748189398i, -0.742774121732+0.5810639864i]}, {"Frequency"=2438508812.5, "S Parameters"=[-0.786930962343+0.524038574383i, -0.145527250693-0.204186723039i, -0.144916876388-0.203637497248i, -0.7383326533+0.586536173064i]}, {"Frequency"=2443821250.0, "S Parameters"=[-0.783023401726+0.529791899792i, -0.146924425778-0.203078253731i, -0.146354621557-0.202583488107i, -0.734113399358+0.59189315494i]}, {"Frequency"=2449133687.5, "S Parameters"=[-0.779041436725+0.53547864525i, -0.148303306974-0.201942563607i, -0.147742240733-0.201445807335i, -0.72963107809+0.59729301042i]}, {"Frequency"=2454446125.0, "S Parameters"=[-0.775207473512+0.541159272114i, -0.149674533639-0.200852188682i, -0.149144860027-0.200343933852i, -0.725248020407+0.60258692524i]}, {"Frequency"=2459758562.5, "S Parameters"=[-0.77113621712+0.546900540442i, -0.15106846872-0.199692997686i, -0.150543881168-0.19915165765i, -0.720838640774+0.607949322164i]}, {"Frequency"=2465071000.0, "S Parameters"=[-0.767178431875+0.552709356099i, -0.152475840947-0.198495832412i, -0.15202625246-0.197964757448i, -0.71642624101+0.613220285504i]}, {"Frequency"=2470383437.5, "S Parameters"=[-0.7631447044+0.558396633124i, -0.153869094156-0.197298705927i, -0.15345359527-0.196756121505i, -0.711976097885+0.618508601496i]}, {"Frequency"=2475695875.0, "S Parameters"=[-0.758891335284+0.564083168319i, -0.155253582695-0.19613152327i, -0.154857898323-0.195486762331i, -0.707578754564+0.623708503442i]}, {"Frequency"=2481008312.5, "S Parameters"=[-0.754707458856+0.569774698424i, -0.156640917329-0.194913118211i, -0.156300703681-0.194194179385i, -0.702871658644+0.629009157595i]}, {"Frequency"=2486320750.0, "S Parameters"=[-0.750291758798+0.575399226109i, -0.157994380408-0.193703338111i, -0.157690588627-0.192978133405i, -0.698112063416+0.634014743472i]}, {"Frequency"=2491633187.5, "S Parameters"=[-0.746100691922+0.580954385168i, -0.15929563876-0.192448901211i, -0.159040547674-0.191684991951i, -0.693374416552+0.639016180921i]}, {"Frequency"=2496945625.0, "S Parameters"=[-0.742043021818+0.586455780796i, -0.160568090919-0.191240463047i, -0.160364704006-0.190496882493i, -0.688649326609+0.644176403481i]}, {"Frequency"=2502258062.5, "S Parameters"=[-0.737930890056+0.591743001937i, -0.161781868681-0.190077679647i, -0.161586483274-0.189277702346i, -0.684222524351+0.649030564639i]}, {"Frequency"=2507570500.0, "S Parameters"=[-0.733543084694+0.596988149508i, -0.16300588991-0.188933185654i, -0.162802563743-0.188089623618i, -0.67947495043+0.654013180216i]}, {"Frequency"=2512882937.5, "S Parameters"=[-0.729348871175+0.602387429425i, -0.164234699537-0.187675210869i, -0.164035824491-0.186843340615i, -0.674612336849+0.658910573464i]}, {"Frequency"=2518195375.0, "S Parameters"=[-0.725097409615+0.607451511191i, -0.165480564375-0.186469803225i, -0.165196933819-0.185567776968i, -0.669732165374+0.663760291075i]}, {"Frequency"=2523507812.5, "S Parameters"=[-0.720764432404+0.612510959116i, -0.166721064916-0.185217478156i, -0.166424566233-0.184326724064i, -0.664674111773+0.668561757365i]}, {"Frequency"=2528820250.0, "S Parameters"=[-0.716457312977+0.617421920839i, -0.168001867822-0.183939090491i, -0.167600379342-0.183103055066i, -0.659601426591+0.673573703194i]}, {"Frequency"=2534132687.5, "S Parameters"=[-0.712024967002+0.622472387918i, -0.169235807904-0.182634086857i, -0.168814021029-0.181853662377i, -0.654373727024+0.678370311092i]}, {"Frequency"=2539445125.0, "S Parameters"=[-0.707729060138+0.627321738976i, -0.170441938637-0.181361987604i, -0.169948370127-0.180613291569i, -0.649038942668+0.683293714467i]}, {"Frequency"=2544757562.5, "S Parameters"=[-0.703331981998+0.63221242081i, -0.171683480035-0.180130917736i, -0.171120032483-0.179357913541i, -0.643932241946+0.688223044097i]}, {"Frequency"=2550070000.0, "S Parameters"=[-0.698984902427+0.637212257998i, -0.172903921549-0.178888544279i, -0.172337798835-0.178070762125i, -0.638710550382+0.693110033917i]}, {"Frequency"=2555382437.5, "S Parameters"=[-0.694755998369+0.641884108803i, -0.174122429145-0.177625351073i, -0.173556466126-0.176842402999i, -0.633518187252+0.698042337592i]}, {"Frequency"=2560694875.0, "S Parameters"=[-0.69039204841+0.646556181752i, -0.175324309386-0.176309572297i, -0.174855584777-0.175587405648i, -0.628218874288+0.702871693114i]}, {"Frequency"=2566007312.5, "S Parameters"=[-0.685989021081+0.651385721336i, -0.176535024197-0.174978182709i, -0.176145895521-0.174250472893i, -0.62275449341+0.707587230272i]}, {"Frequency"=2571319750.0, "S Parameters"=[-0.681185169583+0.656089118025i, -0.177740845303-0.173657940094i, -0.177424214368-0.172912062759i, -0.617256612809+0.71225584904i]}, {"Frequency"=2576632187.5, "S Parameters"=[-0.676354601313+0.660789865311i, -0.178957371443-0.17227654777i, -0.178707818735-0.1715582637i, -0.611604342772+0.717052176656i]}, {"Frequency"=2581944625.0, "S Parameters"=[-0.671630685899+0.665656133524i, -0.180156150943-0.170888210914i, -0.18000468089-0.1701818106i, -0.605905556873+0.721901383632i]}, {"Frequency"=2587257062.5, "S Parameters"=[-0.666788098479+0.670377999258i, -0.181301996543-0.169522108707i, -0.181150673598-0.168826456419i, -0.6004725816+0.726506631571i]}, {"Frequency"=2592569500.0, "S Parameters"=[-0.662087542799+0.6752715012i, -0.182428990864-0.168167774281i, -0.182344078384-0.167440794297i, -0.595106560016+0.731167923622i]}, {"Frequency"=2597881937.5, "S Parameters"=[-0.657224354621+0.679999365676i, -0.183516506716-0.166739273647i, -0.183486895275-0.166052717986i, -0.589641998545+0.735671274046i]}, {"Frequency"=2603194375.0, "S Parameters"=[-0.652259868366+0.684804947347i, -0.184537930466-0.16538088753i, -0.184549799397-0.164610736287i, -0.584165606903+0.739947031766i]}, {"Frequency"=2608506812.5, "S Parameters"=[-0.647431835217+0.68947582961i, -0.185598280339-0.163872282597i, -0.185618725535-0.163127866293i, -0.578581009834+0.744320179011i]}, {"Frequency"=2613819250.0, "S Parameters"=[-0.642380663496+0.694164764922i, -0.186668884845-0.162419892876i, -0.186609840821-0.161630720064i, -0.573135714797+0.748560259178i]}, {"Frequency"=2619131687.5, "S Parameters"=[-0.637322137142+0.698706061245i, -0.187708244116-0.160974650142i, -0.187586398256-0.160117339894i, -0.567765297795+0.752749535427i]}, {"Frequency"=2624444125.0, "S Parameters"=[-0.63222952579+0.703131000074i, -0.188731122812-0.159499947938i, -0.188516089973-0.158590013766i, -0.562184540656+0.756813049749i]}, {"Frequency"=2629756562.5, "S Parameters"=[-0.627169721698+0.707765861425i, -0.189758342111-0.157992495427i, -0.189480616757-0.157047771135i, -0.556716077437+0.760903505987i]}, {"Frequency"=2635069000.0, "S Parameters"=[-0.622150391231+0.712328704527i, -0.190764344029-0.156496131456i, -0.190456767766-0.155493403135i, -0.551303557041+0.764997433384i]}, {"Frequency"=2640381437.5, "S Parameters"=[-0.617173567341+0.716833084197i, -0.191724375569-0.155002254463i, -0.191387044329-0.153999753493i, -0.545956146856+0.769012243687i]}, {"Frequency"=2645693875.0, "S Parameters"=[-0.612350799801+0.72129410353i, -0.192732526926-0.153536266433i, -0.192344515197-0.152555957046i, -0.540666681577+0.773016325525i]}, {"Frequency"=2651006312.5, "S Parameters"=[-0.607439190355+0.725410719315i, -0.193673859447-0.152123872298i, -0.193310150587-0.151103823116i, -0.535398767907+0.776852591851i]}, {"Frequency"=2656318750.0, "S Parameters"=[-0.602484361943+0.729459376816i, -0.194596926416-0.150741556795i, -0.194242455397-0.149741755486i, -0.530114137941+0.780573511862i]}, {"Frequency"=2661631187.5, "S Parameters"=[-0.597430025213+0.733593429872i, -0.195528780785-0.149276274544i, -0.195243870488-0.148323187367i, -0.524487852488+0.784237537919i]}, {"Frequency"=2666943625.0, "S Parameters"=[-0.592229221221+0.737760214131i, -0.196446878002-0.147763888718i, -0.196249960955-0.146856154207i, -0.518749976388+0.787861569115i]}, {"Frequency"=2672256062.5, "S Parameters"=[-0.586977566885+0.741823681015i, -0.197354295963-0.146312637312i, -0.197175980922-0.145443822315i, -0.51302289767+0.791561867262i]}, {"Frequency"=2677568500.0, "S Parameters"=[-0.581747207502+0.745903226457i, -0.198277909425-0.144840986092i, -0.198153759314-0.144103645944i, -0.507208139067+0.795327347955i]}, {"Frequency"=2682880937.5, "S Parameters"=[-0.576448027289+0.750078564099i, -0.199167865103-0.143348397236i, -0.199090443226-0.142635105693i, -0.501408698655+0.799109603256i]}, {"Frequency"=2688193375.0, "S Parameters"=[-0.571017613218+0.754239486791i, -0.200062310141-0.141845193901i, -0.200007911334-0.141149591406i, -0.495426229893+0.802826531902i]}, {"Frequency"=2693505812.5, "S Parameters"=[-0.565704232917+0.75835763796i, -0.200894190582-0.140354858048i, -0.20092275175-0.139699207625i, -0.489397704007+0.806441695885i]}, {"Frequency"=2698818250.0, "S Parameters"=[-0.560258964099+0.762465595921i, -0.201762938433-0.138807585289i, -0.201846760687-0.138162854088i, -0.483306310661+0.810097057117i]}, {"Frequency"=2704130687.5, "S Parameters"=[-0.554932159073+0.766390306401i, -0.202590338861-0.137283652659i, -0.202693355215-0.136638937877i, -0.477300243275+0.813629599902i]}, {"Frequency"=2709443125.0, "S Parameters"=[-0.549477775332+0.77019225279i, -0.20338137195-0.135758556282i, -0.203523375779-0.135078613954i, -0.471296974537+0.817094145874i]}, {"Frequency"=2714755562.5, "S Parameters"=[-0.543885316087+0.774056491392i, -0.204211312388-0.134166995167i, -0.204333881299-0.133433309679i, -0.465138769741+0.820600940448i]}, {"Frequency"=2720068000.0, "S Parameters"=[-0.538274448482+0.777957970472i, -0.205023096919-0.132535422874i, -0.205178204311-0.131794376555i, -0.458928890503+0.824159940246i]}, {"Frequency"=2725380437.5, "S Parameters"=[-0.532741270232+0.781858374193i, -0.205817373846-0.130979306228i, -0.205978173247-0.130160512435i, -0.452943956382+0.82770995027i]}, {"Frequency"=2730692875.0, "S Parameters"=[-0.527404361707+0.785705935151i, -0.206556082864-0.1293304654i, -0.206804965015-0.128545413549i, -0.44698276414+0.831212864738i]}, {"Frequency"=2736005312.5, "S Parameters"=[-0.522045925385+0.789394066968i, -0.20731012681-0.127829443502i, -0.207567683446-0.126925442248i, -0.441050291302+0.834570541589i]}, {"Frequency"=2741317750.0, "S Parameters"=[-0.516721182264+0.793060077258i, -0.208018261229-0.12624165661i, -0.208328395788-0.125358520669i, -0.435168572633+0.837832345023i]}, {"Frequency"=2746630187.5, "S Parameters"=[-0.511343248781+0.796544267529i, -0.208728733564-0.124672973658i, -0.209077791771-0.123783641938i, -0.429343983369+0.840924734965i]}, {"Frequency"=2751942625.0, "S Parameters"=[-0.506020321891+0.799936330939i, -0.209354003296-0.123137264592i, -0.209760591537-0.122289671308i, -0.423286573+0.843849650052i]}, {"Frequency"=2757255062.5, "S Parameters"=[-0.500593209272+0.803325717271i, -0.210025613115-0.121620374416i, -0.210417802389-0.120720150315i, -0.417267171817+0.846935947783i]}, {"Frequency"=2762567500.0, "S Parameters"=[-0.495048110785+0.806795293234i, -0.210689087005-0.120075392875i, -0.211039254671-0.119174677346i, -0.411162399972+0.84999351849i]}, {"Frequency"=2767879937.5, "S Parameters"=[-0.489533624764+0.810302910561i, -0.211347793971-0.118549586753i, -0.21169197976-0.117636244297i, -0.405040508094+0.852958005023i]}, {"Frequency"=2773192375.0, "S Parameters"=[-0.483801011766+0.813651246247i, -0.211974653506-0.116969004836i, -0.212273889208-0.116053879394i, -0.39886729192+0.855884180016i]}, {"Frequency"=2778504812.5, "S Parameters"=[-0.478117888968+0.817234385659i, -0.212612194553-0.115410205104i, -0.212951538627-0.114469973007i, -0.392687217793+0.858768752471i]}, {"Frequency"=2783817250.0, "S Parameters"=[-0.472209688911+0.820681194263i, -0.213244018596-0.113778412875i, -0.213587953735-0.112810773102i, -0.386233926202+0.861597548805i]}, {"Frequency"=2789129687.5, "S Parameters"=[-0.466434609891+0.824042640661i, -0.213917188094-0.112195626522i, -0.214188992182-0.111214795968i, -0.379913623502+0.864537689318i]}, {"Frequency"=2794442125.0, "S Parameters"=[-0.460655703696+0.827315132089i, -0.214522823041-0.110612219278i, -0.214771827896-0.109608703752i, -0.373671697402+0.867233128412i]}, {"Frequency"=2799754562.5, "S Parameters"=[-0.454719142062+0.830609292031i, -0.215114503152-0.109018626545i, -0.215338199164-0.108031398986i, -0.36725003071+0.869857963297i]}, {"Frequency"=2805067000.0, "S Parameters"=[-0.448664205774+0.833720683821i, -0.215690892631-0.107465720818i, -0.215900416384-0.10644231363i, -0.361011695454+0.872596747671i]}, {"Frequency"=2810379437.5, "S Parameters"=[-0.442576359043+0.83705141113i, -0.216240602771-0.105837826502i, -0.216503013302-0.104838895324i, -0.35474710678+0.87513252689i]}, {"Frequency"=2815691875.0, "S Parameters"=[-0.436535516982+0.840322565068i, -0.216795728634-0.104181031297i, -0.217054662873-0.103235814205i, -0.34838569809+0.877814752609i]}, {"Frequency"=2821004312.5, "S Parameters"=[-0.43054323604+0.843698286287i, -0.217299218166-0.102501106686i, -0.217670092767-0.10163071254i, -0.342236299035+0.880467916341i]}, {"Frequency"=2826316750.0, "S Parameters"=[-0.424722511435+0.84668855186i, -0.217786944853-0.100960873702i, -0.218194239952-0.100101009345i, -0.336359292029+0.883053548765i]}, {"Frequency"=2831629187.5, "S Parameters"=[-0.418662425796+0.849727754042i, -0.218283162001-0.0992672068442i, -0.218761782975-0.0984708701537i, -0.33020716975+0.885463770747i]}, {"Frequency"=2836941625.0, "S Parameters"=[-0.412646047924+0.852625722312i, -0.218679631333-0.0976531148829i, -0.219254415845-0.0969253034824i, -0.324310844702+0.887587591473i]}, {"Frequency"=2842254062.5, "S Parameters"=[-0.406723947435+0.855478135625i, -0.21914587141-0.0960799076166i, -0.219761241129-0.095392134077i, -0.318278755935+0.889742160841i]}, {"Frequency"=2847566500.0, "S Parameters"=[-0.400908914624+0.858301971183i, -0.219579999679-0.0945496008433i, -0.220195169463-0.0938928140109i, -0.312338239284+0.891902704044i]}, {"Frequency"=2852878937.5, "S Parameters"=[-0.395021867485+0.861032723501i, -0.219956199377-0.0930284795407i, -0.220607709624-0.0923357451033i, -0.306486047809+0.893907054202i]}, {"Frequency"=2858191375.0, "S Parameters"=[-0.389245977915+0.863664912305i, -0.220356040077-0.091501655841i, -0.221033672605-0.0907755830213i, -0.300534815757+0.895980003512i]}, {"Frequency"=2863503812.5, "S Parameters"=[-0.383307042754+0.866246970227i, -0.220736048033-0.0899458999938i, -0.221421469791-0.0891875970204i, -0.294495080345+0.898000973903i]}, {"Frequency"=2868816250.0, "S Parameters"=[-0.377247661661+0.868978755368i, -0.22111395371-0.0884306016438i, -0.221913343523-0.0875184378653i, -0.288393625752+0.899914338505i]}, {"Frequency"=2874128687.5, "S Parameters"=[-0.371211801997+0.871620047329i, -0.22151504934-0.0868448728911i, -0.222318589838-0.0858749069913i, -0.282001445997+0.901817893747i]}, {"Frequency"=2879441125.0, "S Parameters"=[-0.365097690314+0.874165263217i, -0.222001404672-0.0852038768002i, -0.222747342601-0.0841551239668i, -0.275559608081+0.903895830014i]}, {"Frequency"=2884753562.5, "S Parameters"=[-0.358941927865+0.876701246638i, -0.222458284319-0.0836432304236i, -0.223159657869-0.0824923889112i, -0.269060231024+0.905715191258i]}, {"Frequency"=2890066000.0, "S Parameters"=[-0.352748207647+0.879100548187i, -0.222887646499-0.0820484064499i, -0.223568577368-0.0808064289112i, -0.262599117175+0.90757442632i]}, {"Frequency"=2895378437.5, "S Parameters"=[-0.346520992234+0.881653740762i, -0.22331638537-0.0804219658735i, -0.223983826601-0.079164839613i, -0.255960465527+0.90939983048i]}, {"Frequency"=2900690875.0, "S Parameters"=[-0.340144647914+0.884049431554i, -0.223761438984-0.078775994659i, -0.224330924255-0.0775318848894i, -0.249184525055+0.911406946912i]}, {"Frequency"=2906003312.5, "S Parameters"=[-0.333901918724+0.886492118964i, -0.224115384078-0.0771486996998i, -0.224672385096-0.0759288704941i, -0.242523766904+0.913149668803i]}, {"Frequency"=2911315750.0, "S Parameters"=[-0.327734746361+0.889033477786i, -0.224521820375-0.0754734364539i, -0.225025996845-0.0743537148205i, -0.235908024267+0.91514936i]}, {"Frequency"=2916628187.5, "S Parameters"=[-0.3213272977+0.891429009722i, -0.224802861805-0.0737859552984i, -0.225341882578-0.0727276863438i, -0.229233549972+0.91695080958i]}, {"Frequency"=2921940625.0, "S Parameters"=[-0.315096134826+0.893651384517i, -0.22506767755-0.0720895677779i, -0.225638574819-0.0711672808329i, -0.22251017938+0.918655928956i]}, {"Frequency"=2927253062.5, "S Parameters"=[-0.308904765345+0.895915746803i, -0.225287923393-0.0703788810883i, -0.22592247765-0.0696080323459i, -0.21580040097+0.920338701054i]}, {"Frequency"=2932565500.0, "S Parameters"=[-0.302633766539+0.898050575555i, -0.225540919261-0.0686836882375i, -0.22612646228-0.0680415648039i, -0.20896331336+0.921869475646i]}, {"Frequency"=2937877937.5, "S Parameters"=[-0.296472074645+0.900119985528i, -0.225703123546-0.0670968788482i, -0.226355495653-0.0664744202387i, -0.202371819886+0.923384544149i]}, {"Frequency"=2943190375.0, "S Parameters"=[-0.290491263289+0.902193641281i, -0.225827224991-0.0654181156503i, -0.226534227922-0.0649336758429i, -0.195590245031+0.924811685633i]}, {"Frequency"=2948502812.5, "S Parameters"=[-0.284551610826+0.904113722698i, -0.225903189502-0.0638581180746i, -0.226669909763-0.0633624980461i, -0.189126105573+0.926231597615i]}, {"Frequency"=2953815250.0, "S Parameters"=[-0.27859093912+0.905948021796i, -0.22603009826-0.0623318965947i, -0.226852128707-0.0617780070849i, -0.182532488944+0.927547868858i]}, {"Frequency"=2959127687.5, "S Parameters"=[-0.272640005925+0.907775735678i, -0.226139615851-0.0607854355302i, -0.227029810053-0.0602206507385i, -0.175820953983+0.928753462399i]}, {"Frequency"=2964440125.0, "S Parameters"=[-0.266632910175+0.909531377887i, -0.226286809269-0.0592654423819i, -0.227254791171-0.058628267917i, -0.168984240688+0.929916107031i]}, {"Frequency"=2969752562.5, "S Parameters"=[-0.260724888391+0.911208121677i, -0.226552032466-0.0577317624781i, -0.227578204556-0.0570756212026i, -0.162304327836+0.930995271013i]}, {"Frequency"=2975065000.0, "S Parameters"=[-0.254804054213+0.912731408847i, -0.226815158261-0.0562110566036i, -0.227888309493-0.0554262704351i, -0.155643775252+0.932095429629i]}, {"Frequency"=2980377437.5, "S Parameters"=[-0.248705917979+0.914277368431i, -0.22708595365-0.0545266100643i, -0.228158103465-0.053719388845i, -0.148754972963+0.933166234204i]}, {"Frequency"=2985689875.0, "S Parameters"=[-0.242384846648+0.915854014637i, -0.227300433872-0.0528931413378i, -0.228439244308-0.051960380114i, -0.141788980516+0.93417491832i]}, {"Frequency"=2991002312.5, "S Parameters"=[-0.236002446313+0.9176386796i, -0.227497448639-0.0512334281441i, -0.22866786057-0.0502454452372i, -0.134851233592+0.935215977816i]}, {"Frequency"=2996314750.0, "S Parameters"=[-0.229633119655+0.91929871728i, -0.227729090271-0.0495526342823i, -0.228868884541-0.0486035223712i, -0.128016443331+0.936350575939i]}, {"Frequency"=3001627187.5, "S Parameters"=[-0.223186931058+0.920815506226i, -0.227921738113-0.0478527319151i, -0.229010086569-0.0469522510455i, -0.12104437216+0.937363544002i]}, {"Frequency"=3006939625.0, "S Parameters"=[-0.216703768425+0.922338410314i, -0.228060844656-0.0462138241984i, -0.229056546276-0.0453095935439i, -0.114235297688+0.938397386558i]}, {"Frequency"=3012252062.5, "S Parameters"=[-0.209986872923+0.924024210726i, -0.228119350094-0.0444813462763i, -0.229153156463-0.0436123785706i, -0.107319560356+0.939345212539i]}, {"Frequency"=3017564500.0, "S Parameters"=[-0.203276674293+0.925446355296i, -0.228153052049-0.0427711674151i, -0.229120272546-0.0419421260372i, -0.100476473298+0.940087747079i]}, {"Frequency"=3022876937.5, "S Parameters"=[-0.196445551982+0.926975929513i, -0.228127007062-0.0410245912559i, -0.229116256449-0.0402819491576i, -0.0933946345642+0.940821056798i]}, {"Frequency"=3028189375.0, "S Parameters"=[-0.18978764767+0.92853291953i, -0.228102406807-0.0393248703992i, -0.229068723072-0.0386180929333i, -0.0865199044034+0.94167949823i]}, {"Frequency"=3033501812.5, "S Parameters"=[-0.182977200426+0.929970644337i, -0.228009785389-0.0376448243584i, -0.229002602987-0.0369245497899i, -0.079701999595+0.942376488741i]}, {"Frequency"=3038814250.0, "S Parameters"=[-0.176444580428+0.931322662023i, -0.227866018424-0.0359878827023i, -0.228852112945-0.0352253942583i, -0.0730429118708+0.942989846446i]}, {"Frequency"=3044126687.5, "S Parameters"=[-0.169932795734+0.93262154577i, -0.227711331957-0.0343739537585i, -0.228760920498-0.0336164652572i, -0.0665221920287+0.943644558714i]}, {"Frequency"=3049439125.0, "S Parameters"=[-0.16354382157+0.934041302009i, -0.227584617195-0.0327921024795i, -0.228635621866-0.0320600520678i, -0.0599193360298+0.944203252762i]}, {"Frequency"=3054751562.5, "S Parameters"=[-0.157413761391+0.935310947669i, -0.227428952867-0.0312403871534i, -0.228550425843-0.0305666663221i, -0.0533456268722+0.944735504697i]}, {"Frequency"=3060064000.0, "S Parameters"=[-0.151257296433+0.936320654203i, -0.227279600328-0.0297844114162i, -0.228435686843-0.0290339069027i, -0.0470629468908+0.945177394718i]}, {"Frequency"=3065376437.5, "S Parameters"=[-0.145003642465+0.937397691956i, -0.227171031972-0.0282601624453i, -0.228346693109-0.0275573294177i, -0.0405526479358+0.945496066877i]}, {"Frequency"=3070688875.0, "S Parameters"=[-0.138732181353+0.938350822295i, -0.22707783736-0.0268043449822i, -0.228348846802-0.0259979780257i, -0.0342016087414+0.945725468058i]}, {"Frequency"=3076001312.5, "S Parameters"=[-0.132608085734+0.939249748895i, -0.227007038335-0.0252407710879i, -0.228309232728-0.0244828075831i, -0.0276934904311+0.945934664428i]}, {"Frequency"=3081313750.0, "S Parameters"=[-0.126382882085+0.940155100361i, -0.226950376978-0.0237424561233i, -0.228256085423-0.0229592833687i, -0.0212072167864+0.946192342135i]}, {"Frequency"=3086626187.5, "S Parameters"=[-0.120108523677+0.941026591366i, -0.226914763032-0.0221890097032i, -0.228218381848-0.0214685081741i, -0.01477260056+0.946435707752i]}, {"Frequency"=3091938625.0, "S Parameters"=[-0.114027384804+0.941874142079i, -0.22682084353-0.0206628813369i, -0.228143868309-0.0199944869074i, -0.00832356111885+0.946632079004i]}, {"Frequency"=3097251062.5, "S Parameters"=[-0.10772627604+0.942639094534i, -0.226683609842-0.0191727590866i, -0.228082770086-0.0184306749143i, -0.0019455608385+0.946757619458i]}, {"Frequency"=3102563500.0, "S Parameters"=[-0.101370311824+0.943248586662i, -0.226575437575-0.0176027194824i, -0.227925068439-0.0169576831876i, 0.00444346363254+0.946726714841i]}, {"Frequency"=3107875937.5, "S Parameters"=[-0.0949961828205+0.943951129315i, -0.226433864866-0.0160678635143i, -0.227766232217-0.0153778121024i, 0.0109349572799+0.946700771719i]}, {"Frequency"=3113188375.0, "S Parameters"=[-0.088410861015+0.944595832841i, -0.22622607441-0.0143956975952i, -0.227642570355-0.0137804614236i, 0.0176053309027+0.946605213992i]}, {"Frequency"=3118500812.5, "S Parameters"=[-0.0816464448404+0.945152662806i, -0.225998694673-0.0128234981284i, -0.227447100957-0.012125475168i, 0.0241442367759+0.946450180482i]}, {"Frequency"=3123813250.0, "S Parameters"=[-0.0749422353547+0.945782774972i, -0.225823614566-0.0111950833699i, -0.227271906596-0.0105054302441i, 0.0308992778147+0.946270337818i]}, {"Frequency"=3129125687.5, "S Parameters"=[-0.0681937143782+0.946262753888i, -0.22556380777-0.00954011626857i, -0.227008743837-0.00887743802076i, 0.0374710468121+0.946070164063i]}, {"Frequency"=3134438125.0, "S Parameters"=[-0.0614472816541+0.946808692374i, -0.225262360077-0.00793092917325i, -0.226793006071-0.00724692024916i, 0.0442115283049+0.945785524185i]}, {"Frequency"=3139750562.5, "S Parameters"=[-0.0546954418608+0.947242561883i, -0.225084225957-0.0063383588565i, -0.226520932438-0.00560643566818i, 0.05084078303+0.945571285296i]}, {"Frequency"=3145063000.0, "S Parameters"=[-0.0482468285456+0.947681688351i, -0.224745839023-0.00485333563993i, -0.226264961939-0.00408485639625i, 0.0573167946465+0.945231865208i]}, {"Frequency"=3150375437.5, "S Parameters"=[-0.0416954585085+0.947945089315i, -0.224474172216-0.0033398190628i, -0.225939512818-0.00259260832581i, 0.0638458587606+0.944920726487i]}, {"Frequency"=3155687875.0, "S Parameters"=[-0.0352442462783+0.948309096751i, -0.224158205218-0.00189506830445i, -0.225613713308-0.00116230791352i, 0.0701783932298+0.944395150986i]}, {"Frequency"=3161000312.5, "S Parameters"=[-0.0287983682322+0.948513698142i, -0.223879486228-0.000464128823219i, -0.225300302173+0.000252566484985i, 0.0765705890067+0.943893634076i]}, {"Frequency"=3166312750.0, "S Parameters"=[-0.0222897878854+0.948779357504i, -0.223562640663+0.000970588780805i, -0.224982140783+0.00166091134056i, 0.0829483023774+0.943393075153i]}, {"Frequency"=3171625187.5, "S Parameters"=[-0.0160035262425+0.948893597906i, -0.223235819877+0.00242632362265i, -0.224694604163+0.00303120187434i, 0.0893261386171+0.942768443409i]}, {"Frequency"=3176937625.0, "S Parameters"=[-0.00962456646699+0.94901841916i, -0.223000104249+0.00390445969955i, -0.224372239375+0.00445429038373i, 0.0955638140009+0.942222168214i]}, {"Frequency"=3182250062.5, "S Parameters"=[-0.00335732330187+0.949186426352i, -0.222708091873+0.00535707209384i, -0.224044931565+0.00578321597408i, 0.101922842178+0.941629853045i]}, {"Frequency"=3187562500.0, "S Parameters"=[0.00302192525317+0.949246640716i, -0.222400048192+0.00681438330842i, -0.223710076306+0.00721094600135i, 0.108223099592+0.940980416624i]}, {"Frequency"=3192874937.5, "S Parameters"=[0.00939079908306+0.949171527228i, -0.22207537834+0.00834648713905i, -0.223383755236+0.00865574855366i, 0.114653149462+0.94024294375i]}, {"Frequency"=3198187375.0, "S Parameters"=[0.0157004779773+0.949148598808i, -0.221761540968+0.00981007779395i, -0.223040858919+0.0100803492101i, 0.12097690689+0.939433961982i]}, {"Frequency"=3203499812.5, "S Parameters"=[0.0220599991473+0.948996411662i, -0.221425371292+0.0112344182311i, -0.222730471626+0.0115504435704i, 0.127385106497+0.938537954834i]}, {"Frequency"=3208812250.0, "S Parameters"=[0.028492526619+0.948794019825i, -0.221048419132+0.0127451586003i, -0.222363051012+0.0130329472152i, 0.133887868797+0.937627260216i]}, {"Frequency"=3214124687.5, "S Parameters"=[0.0350121664256+0.948537710543i, -0.220631833942+0.0142775148391i, -0.222036467764+0.0145730670359i, 0.140535808072+0.936609244414i]}, {"Frequency"=3219437125.0, "S Parameters"=[0.0415557110059+0.948329093772i, -0.220242733942+0.0157565480257i, -0.221735529909+0.0161195759339i, 0.147124735072+0.935555195399i]}, {"Frequency"=3224749562.5, "S Parameters"=[0.0481424467062+0.948026077476i, -0.219862350943+0.0172940365896i, -0.221453270715+0.0176782922667i, 0.15388600327+0.934538619884i]}, {"Frequency"=3230062000.0, "S Parameters"=[0.0547625810469+0.947683282798i, -0.219455384853+0.0187873020323i, -0.221086615947+0.0191953724048i, 0.160680565037+0.933428371449i]}, {"Frequency"=3235374437.5, "S Parameters"=[0.0613970263049+0.947349415668i, -0.219027711544+0.0202680450128i, -0.220744883927+0.0207068219491i, 0.167469485968+0.932193554415i]}, {"Frequency"=3240686875.0, "S Parameters"=[0.0678710037878+0.946832538075i, -0.218568795556+0.0216608995611i, -0.220328253719+0.0221597809344i, 0.174149492479+0.930954047843i]}, {"Frequency"=3245999312.5, "S Parameters"=[0.0744029841427+0.946400777296i, -0.218105046599+0.0231190325397i, -0.219919484308+0.0236243750534i, 0.180767819398+0.929793468056i]}, {"Frequency"=3251311750.0, "S Parameters"=[0.0808516976852+0.945760288966i, -0.217628269015+0.024501974086i, -0.219429030889+0.0250661705368i, 0.187368813231+0.928340236356i]}, {"Frequency"=3256624187.5, "S Parameters"=[0.0872328558042+0.945152473477i, -0.217101343488+0.0258706224646i, -0.218942265549+0.0264350405099i, 0.193941426954+0.927076719307i]}, {"Frequency"=3261936625.0, "S Parameters"=[0.0936864664997+0.944611757267i, -0.216629742462+0.0272915219423i, -0.218364619394+0.0277906973788i, 0.200475114024+0.925663771602i]}, {"Frequency"=3267249062.5, "S Parameters"=[0.100098048332+0.943980823902i, -0.216105386468+0.0286892009667i, -0.217816475958+0.0291798683389i, 0.207129923459+0.924292220298i]}, {"Frequency"=3272561500.0, "S Parameters"=[0.106467656103+0.943303605315i, -0.215547069732+0.0300962967691i, -0.217205684861+0.0305596228244i, 0.213555968672+0.922873787807i]}, {"Frequency"=3277873937.5, "S Parameters"=[0.11291647767+0.942676722827i, -0.215018549828+0.0315087847854i, -0.216602845345+0.0319757063554i, 0.220050947239+0.921337542426i]}, {"Frequency"=3283186375.0, "S Parameters"=[0.11930248483+0.94194284961i, -0.214478235445+0.0328901455309i, -0.216014350081+0.033326495924i, 0.226553965197+0.919809813825i]}, {"Frequency"=3288498812.5, "S Parameters"=[0.125541751388+0.941141715366i, -0.21396577198+0.0343037811122i, -0.215398959811+0.0346974508992i, 0.23293196196+0.918209495745i]}, {"Frequency"=3293811250.0, "S Parameters"=[0.131837850992+0.940431656467i, -0.213357228723+0.0356813473522i, -0.214823167833+0.0360715475459i, 0.239221122901+0.916632026857i]}, {"Frequency"=3299123687.5, "S Parameters"=[0.138077679796+0.939502348644i, -0.212803255985+0.0370339734086i, -0.21424508653+0.0374144295698i, 0.245541667095+0.915015654867i]}, {"Frequency"=3304436125.0, "S Parameters"=[0.144345233522+0.938561013923i, -0.212216414119+0.0383551743039i, -0.213701239633+0.0387114534867i, 0.251818574076+0.913232075502i]}, {"Frequency"=3309748562.5, "S Parameters"=[0.15063548474+0.937690429582i, -0.211666986366+0.0397046968663i, -0.213178616932+0.0400282508023i, 0.258210753958+0.911311895436i]}, {"Frequency"=3315061000.0, "S Parameters"=[0.156909235376+0.936718751194i, -0.211081993591+0.0410519435993i, -0.212672466514+0.0413463205481i, 0.264584052823+0.909542922534i]}, {"Frequency"=3320373437.5, "S Parameters"=[0.163358745844+0.935542176153i, -0.21054361638+0.0424418604192i, -0.212158863895+0.0426355278381i, 0.270967083366+0.907533943562i]}, {"Frequency"=3325685875.0, "S Parameters"=[0.169880721339+0.934419877076i, -0.209947034299+0.0437704653799i, -0.211602524699+0.0439702392858i, 0.277507246724+0.90549076839i]}, {"Frequency"=3330998312.5, "S Parameters"=[0.176322069966+0.933186811514i, -0.209389546378+0.0451533041624i, -0.211072649836+0.0452637831225i, 0.284003197277+0.903466656399i]}, {"Frequency"=3336310750.0, "S Parameters"=[0.182746932864+0.932054074301i, -0.208732787991+0.046483925371i, -0.210551453975+0.0466057239727i, 0.290424228115+0.901399799195i]}, {"Frequency"=3341623187.5, "S Parameters"=[0.189081603834+0.930685795175i, -0.208099987281+0.0477810846771i, -0.209941012664+0.0478879964332i, 0.296855761279+0.899228303346i]}, {"Frequency"=3346935625.0, "S Parameters"=[0.195376832838+0.9293563557i, -0.207487237346+0.0490721563995i, -0.209302089235+0.0491782362714i, 0.303101504154+0.897230455182i]}, {"Frequency"=3352248062.5, "S Parameters"=[0.2016766202+0.927999461527i, -0.206816279574+0.0503503957821i, -0.208661318938+0.0504308463182i, 0.309410390937+0.89499902942i]}, {"Frequency"=3357560500.0, "S Parameters"=[0.207910871518+0.926583222883i, -0.206149926048+0.0515891663128i, -0.207923725397+0.0517442438891i, 0.315641715886+0.892921696179i]}, {"Frequency"=3362872937.5, "S Parameters"=[0.21437998325+0.925155700385i, -0.205430724447+0.0528391153747i, -0.207188913512+0.0530745112771i, 0.321968432573+0.890784204083i]}, {"Frequency"=3368185375.0, "S Parameters"=[0.220645930983+0.923742233366i, -0.204739535336+0.0541290552563i, -0.206392785119+0.0543810813938i, 0.328207359688+0.888567104249i]}, {"Frequency"=3373497812.5, "S Parameters"=[0.22679824834+0.922166705219i, -0.204017270903+0.0553983618358i, -0.205667528742+0.0556567564076i, 0.334338419261+0.886388136659i]}, {"Frequency"=3378810250.0, "S Parameters"=[0.233109366142+0.920722580944i, -0.203289077051+0.0567103066734i, -0.204900109016+0.0569646834111i, 0.340420221024+0.8842188908i]}, {"Frequency"=3384122687.5, "S Parameters"=[0.239180063791+0.919169949803i, -0.202549005758+0.0579180375794i, -0.204114093934+0.0582009600529i, 0.346424845434+0.881982969641i]}, {"Frequency"=3389435125.0, "S Parameters"=[0.245325815667+0.917673831001i, -0.201814604191+0.0591635122116i, -0.203326590358+0.059436042206i, 0.352408702825+0.879695385837i]}, {"Frequency"=3394747562.5, "S Parameters"=[0.251377424083+0.916095919309i, -0.20113726191+0.0603654899174i, -0.202679933314+0.0606637149964i, 0.35819918481+0.87735863602i]}, {"Frequency"=3400060000.0, "S Parameters"=[0.257350696659+0.914463220352i, -0.200397863901+0.0615321044873i, -0.201896116027+0.0618371491038i, 0.36405636205+0.874903664958i]}, {"Frequency"=3405372437.5, "S Parameters"=[0.263191209931+0.912785148282i, -0.199696744332+0.0627112188055i, -0.201202509055+0.0629191130445i, 0.369840092933+0.872410813431i]}, {"Frequency"=3410684875.0, "S Parameters"=[0.269107369973+0.911010624797i, -0.198988678111+0.0638394737947i, -0.200530713282+0.0640221768699i, 0.375607750607+0.86991954082i]}, {"Frequency"=3415997312.5, "S Parameters"=[0.275268587307+0.909221399308i, -0.198302149003+0.065065346878i, -0.199808753311+0.0651359574914i, 0.381559175529+0.86726320603i]}, {"Frequency"=3421309750.0, "S Parameters"=[0.281315129966+0.907424157899i, -0.197554541708+0.066231048136i, -0.199102772358+0.0662618250909i, 0.387490841094+0.864524440731i]}, {"Frequency"=3426622187.5, "S Parameters"=[0.287370395582+0.905485208133i, -0.196796092754+0.0673418763474i, -0.198414362067+0.0673638556989i, 0.393404135548+0.861799441437i]}, {"Frequency"=3431934625.0, "S Parameters"=[0.29350743926+0.903548532921i, -0.196057842662+0.0685420212739i, -0.197682241611+0.0685034492453i, 0.399534267279+0.859055262672i]}, {"Frequency"=3437247062.5, "S Parameters"=[0.299646164154+0.901331153535i, -0.195302074691+0.0696517852313i, -0.196942397416+0.0695972985088i, 0.405597885277+0.855920278175i]}, {"Frequency"=3442559500.0, "S Parameters"=[0.305677299349+0.899069435304i, -0.194523539641+0.0707409561027i, -0.196097977274+0.0707324445028i, 0.411562716536+0.852960902399i]}, {"Frequency"=3447871937.5, "S Parameters"=[0.311747115769+0.896860971202i, -0.193762762769+0.0718245396277i, -0.195314389004+0.0718069965488i, 0.417577787683+0.849903540914i]}, {"Frequency"=3453184375.0, "S Parameters"=[0.317905590621+0.894644090065i, -0.192917346246+0.0729227575086i, -0.19448321162+0.0729306423957i, 0.423725842475+0.846801754479i]}, {"Frequency"=3458496812.5, "S Parameters"=[0.324003737875+0.892475611837i, -0.192088766162+0.0740168171051i, -0.193645596399+0.0740494827545i, 0.429703901084+0.843772997219i]}, {"Frequency"=3463809250.0, "S Parameters"=[0.329967215125+0.890298868887i, -0.191282350155+0.0750945332055i, -0.192829543838+0.0751588975705i, 0.435754869686+0.840687748541i]}, {"Frequency"=3469121687.5, "S Parameters"=[0.335946150256+0.888014839603i, -0.190389462881+0.0762177432403i, -0.191985086301+0.0762592164549i, 0.441792670429+0.837472224846i]}, {"Frequency"=3474434125.0, "S Parameters"=[0.341757719126+0.885805853398i, -0.18959299304+0.0772599060481i, -0.191156506612+0.0773248703216i, 0.447589465272+0.83443147046i]}, {"Frequency"=3479746562.5, "S Parameters"=[0.347528202547+0.883362876769i, -0.188754763374+0.0783323925248i, -0.190310049501+0.0783489242358i, 0.45333407242+0.831258861746i]}, {"Frequency"=3485059000.0, "S Parameters"=[0.353333521429+0.88109913725i, -0.18793333545+0.0793768091448i, -0.189536831183+0.0793609474377i, 0.459063556126+0.827986076792i]}, {"Frequency"=3490371437.5, "S Parameters"=[0.3589072292+0.87879182245i, -0.187176096632+0.0803803866898i, -0.188745180672+0.0803144319724i, 0.464702329599+0.824796130265i]}, {"Frequency"=3495683875.0, "S Parameters"=[0.36432545137+0.876326983285i, -0.186440334328+0.0813413141961i, -0.188014040409+0.0812227294126i, 0.469985293315+0.821658569627i]}, {"Frequency"=3500996312.5, "S Parameters"=[0.369834067002+0.873909394601i, -0.185693524986+0.0822838658691i, -0.187324294478+0.0821731356299i, 0.475344554528+0.818493647428i]}, {"Frequency"=3506308750.0, "S Parameters"=[0.37549688373+0.871392711712i, -0.184951317298+0.0832591537931i, -0.186576738483+0.0831258076611i, 0.480641892378+0.815266614971i]}, {"Frequency"=3511621187.5, "S Parameters"=[0.381085136204+0.868961027513i, -0.184223056607+0.0842648897397i, -0.185829952668+0.0840937404388i, 0.486051329387+0.812076148473i]}, {"Frequency"=3516933625.0, "S Parameters"=[0.386782788505+0.866311332434i, -0.183457465475+0.0852791332148i, -0.185048739295+0.0851061328409i, 0.491475225588+0.808761421419i]}, {"Frequency"=3522246062.5, "S Parameters"=[0.392477543602+0.863556651979i, -0.182673940816+0.0862692694288i, -0.184210840691+0.0861514842657i, 0.496736480273+0.805395707572i]}, {"Frequency"=3527558500.0, "S Parameters"=[0.39825221074+0.860638055839i, -0.181864241059+0.0872663329277i, -0.183399845184+0.0871582920579i, 0.50200499743+0.801892627431i]}, {"Frequency"=3532870937.5, "S Parameters"=[0.404142812532+0.85755715036i, -0.181036483191+0.0882420239759i, -0.182514430447+0.0881606539327i, 0.507304940518+0.79833186628i]}, {"Frequency"=3538183375.0, "S Parameters"=[0.41020092476+0.854492301554i, -0.180238961066+0.0891923763895i, -0.181640431772+0.0891399368895i, 0.512620817559+0.794757216673i]}, {"Frequency"=3543495812.5, "S Parameters"=[0.416177229781+0.851401842081i, -0.179405999476+0.0901208688234i, -0.180791956134+0.0900401279385i, 0.51789245229+0.791043198707i]}, {"Frequency"=3548808250.0, "S Parameters"=[0.422245837072+0.848486278634i, -0.178600423758+0.0910417953134i, -0.179975695368+0.0909882745163i, 0.523188738509+0.787549530039i]}, {"Frequency"=3554120687.5, "S Parameters"=[0.428001781615+0.845432373368i, -0.177832594247+0.091926276011i, -0.179170982921+0.0918385727463i, 0.528277922764+0.784007272641i]}, {"Frequency"=3559433125.0, "S Parameters"=[0.433786968274+0.842424285616i, -0.177094214519+0.0928479893142i, -0.178413048417+0.0927269304851i, 0.533353043501+0.780592980824i]}, {"Frequency"=3564745562.5, "S Parameters"=[0.439464064898+0.839464402945i, -0.176347886303+0.0938169231154i, -0.177685780983+0.0936470443902i, 0.538182749983+0.777180753771i]}, {"Frequency"=3570058000.0, "S Parameters"=[0.444996803007+0.836402889274i, -0.175608867313+0.0948079124483i, -0.177024837013+0.094591397527i, 0.543149618572+0.773579511538i]}, {"Frequency"=3575370437.5, "S Parameters"=[0.450250970547+0.833554625051i, -0.174923004775+0.0957828883386i, -0.176373996+0.0954884760345i, 0.548028094789+0.770044595134i]}, {"Frequency"=3580682875.0, "S Parameters"=[0.45547385794+0.830637531397i, -0.17425949799+0.0967990096288i, -0.175683354835+0.0964275482584i, 0.552848576495+0.76666286501i]}, {"Frequency"=3585995312.5, "S Parameters"=[0.460493484799+0.827878573998i, -0.173559706223+0.0978053120845i, -0.175035464465+0.0973615452524i, 0.557624807624+0.763151534804i]}, {"Frequency"=3591307750.0, "S Parameters"=[0.465306272194+0.825153422498i, -0.172859905482+0.0988055822659i, -0.174405669765+0.0983334693703i, 0.562283409865+0.759611258424i]}, {"Frequency"=3596620187.5, "S Parameters"=[0.470179320152+0.822651309183i, -0.172145732391+0.0997956529471i, -0.173761999085+0.0993135626158i, 0.56699717038+0.75615134989i]}, {"Frequency"=3601932625.0, "S Parameters"=[0.474973599187+0.820080296452i, -0.171453690602+0.100802477321i, -0.173100322001+0.100368516093i, 0.571713571381+0.752616166894i]}, {"Frequency"=3607245062.5, "S Parameters"=[0.479479213792+0.817496670852i, -0.170760258176+0.101864061625i, -0.172349098208+0.101446612673i, 0.576410625626+0.749159329379i]}, {"Frequency"=3612557500.0, "S Parameters"=[0.484120389624+0.81480286936i, -0.169995943589+0.102962661651i, -0.171548976207+0.102553510049i, 0.581179038166+0.745481914535i]}, {"Frequency"=3617869937.5, "S Parameters"=[0.488860050577+0.811843716054i, -0.169157651499+0.104098333272i, -0.170694254794+0.10372722509i, 0.586027900488+0.741591706427i]}, {"Frequency"=3623182375.0, "S Parameters"=[0.493669430352+0.808919675691i, -0.168334761663+0.105209823028i, -0.169789010336+0.104950659479i, 0.590845804242+0.737557096521i]}, {"Frequency"=3628494812.5, "S Parameters"=[0.498654922322+0.805825593168i, -0.167455144833+0.106381502586i, -0.168830790629+0.106122941753i, 0.595844781877+0.733537129259i]}, {"Frequency"=3633807250.0, "S Parameters"=[0.504021504275+0.802749014633i, -0.16650864459+0.107523884987i, -0.167848261604+0.107331918512i, 0.600951321622+0.729433266572i]}, {"Frequency"=3639119687.5, "S Parameters"=[0.509326938242+0.799680852205i, -0.165566808489+0.108712741375i, -0.166865746453+0.108500890073i, 0.606379346373+0.725357147285i]}, {"Frequency"=3644432125.0, "S Parameters"=[0.514743091075+0.796564285779i, -0.164604857781+0.109842776883i, -0.165841802574+0.109630443599i, 0.611398827595+0.721446169315i]}, {"Frequency"=3649744562.5, "S Parameters"=[0.520233958445+0.79325927637i, -0.163581674267+0.11098734274i, -0.164783958926+0.110727071584i, 0.616510904721+0.717478345447i]}, {"Frequency"=3655057000.0, "S Parameters"=[0.525743561873+0.789770881002i, -0.162525193885+0.1120986544i, -0.163717499972+0.111821782011i, 0.62150108484+0.713418462631i]}, {"Frequency"=3660369437.5, "S Parameters"=[0.531087312895+0.786189648905i, -0.161421162344+0.113129210792i, -0.162643148695+0.112817863606i, 0.626404498812+0.709193448334i]}, {"Frequency"=3665681875.0, "S Parameters"=[0.536695530243+0.782504298265i, -0.160306394411+0.114186100803i, -0.161510851179+0.11377582023i, 0.631492426333+0.704967622131i]}, {"Frequency"=3670994312.5, "S Parameters"=[0.542248611282+0.778753937273i, -0.159159467544+0.115241422768i, -0.160374879097+0.11470057407i, 0.636643582899+0.700572539056i]}, {"Frequency"=3676306750.0, "S Parameters"=[0.547829133769+0.775010540555i, -0.157994715675+0.116185085227i, -0.159201551932+0.115597629884i, 0.64148853089+0.696283036669i]}, {"Frequency"=3681619187.5, "S Parameters"=[0.55349263944+0.771083999016i, -0.156800595862+0.117081663004i, -0.158026752548+0.116465026875i, 0.646431362989+0.691950601929i]}, {"Frequency"=3686931625.0, "S Parameters"=[0.559058853242+0.76742835625i, -0.155619182813+0.117906044143i, -0.156831501779+0.11731124619i, 0.651357438954+0.687583360795i]}, {"Frequency"=3692244062.5, "S Parameters"=[0.564428367255+0.763692311589i, -0.154432035709+0.118704046906i, -0.155687318291+0.11808665745i, 0.65621052556+0.683221626173i]}, {"Frequency"=3697556500.0, "S Parameters"=[0.569582063838+0.759972557223i, -0.153303432688+0.119457852536i, -0.154576048007+0.11886151364i, 0.660899071315+0.678842018669i]}, {"Frequency"=3702868937.5, "S Parameters"=[0.574568983508+0.755990782754i, -0.15217212733+0.12021129959i, -0.153446217803+0.119637526283i, 0.665403379849+0.674281012854i]}, {"Frequency"=3708181375.0, "S Parameters"=[0.579606643+0.752010954498i, -0.151017114917+0.120930310225i, -0.152303100359+0.120448666198i, 0.6698600833+0.669638821038i]}, {"Frequency"=3713493812.5, "S Parameters"=[0.584694836299+0.748064281049i, -0.149884060378+0.121697794381i, -0.151188343978+0.121233761687i, 0.674437684342+0.664797713368i]}, {"Frequency"=3718806250.0, "S Parameters"=[0.589669121197+0.743972147293i, -0.14875820971+0.122434283724i, -0.150037193826+0.122019021186i, 0.678971961565+0.66009016724i]}, {"Frequency"=3724118687.5, "S Parameters"=[0.59488048148+0.739853519705i, -0.147638987601+0.123223371356i, -0.148862531843+0.122824929043i, 0.683617338121+0.655362374244i]}, {"Frequency"=3729431125.0, "S Parameters"=[0.600017399804+0.735991464862i, -0.146528138719+0.124026387248i, -0.147730461599+0.123616199495i, 0.688240207864+0.650635889691i]}, {"Frequency"=3734743562.5, "S Parameters"=[0.605132050145+0.732091373731i, -0.145364798292+0.124770990997i, -0.14660332962+0.124406420532i, 0.692745930371+0.645983175794i]}, {"Frequency"=3740056000.0, "S Parameters"=[0.61008054056+0.72813344386i, -0.144291716041+0.125517604249i, -0.145491889216+0.125125372427i, 0.697065668927+0.641533141311i]}, {"Frequency"=3745368437.5, "S Parameters"=[0.615038163487+0.724034794657i, -0.143163677698+0.126229982929i, -0.144379541037+0.125856157171i, 0.701275885046+0.636930354928i]}, {"Frequency"=3750680875.0, "S Parameters"=[0.619821570192+0.719944448115i, -0.142080949633+0.126946494397i, -0.143276858268+0.126469442521i, 0.705441362632+0.632396731837i]}, {"Frequency"=3755993312.5, "S Parameters"=[0.624633458687+0.715719468179i, -0.140975202208+0.127633831751i, -0.142189808618+0.127133190102i, 0.709526325602+0.627525572444i]}, {"Frequency"=3761305750.0, "S Parameters"=[0.629434067895+0.711564621896i, -0.139881844979+0.128345241951i, -0.141055880501+0.127745849174i, 0.713708748443+0.622686279352i]}, {"Frequency"=3766618187.5, "S Parameters"=[0.634254058225+0.707256353236i, -0.138797989875+0.129003980876i, -0.139924404865+0.12838154755i, 0.717859610068+0.61792257836i]}, {"Frequency"=3771930625.0, "S Parameters"=[0.639154893623+0.703172597258i, -0.13765926067+0.12961308814i, -0.138778388073+0.129008760562i, 0.72201098972+0.612989890562i]}, {"Frequency"=3777243062.5, "S Parameters"=[0.643895797242+0.699138906648i, -0.136515768961+0.130261468711i, -0.137605191013+0.129671887108i, 0.726184475222+0.607972493805i]}, {"Frequency"=3782555500.0, "S Parameters"=[0.648461306969+0.695084808164i, -0.135376325847+0.130905838722i, -0.136437946959+0.130301527386i, 0.730445273039+0.603106293091i]}, {"Frequency"=3787867937.5, "S Parameters"=[0.65269598091+0.691042104417i, -0.134232836434+0.131534732377i, -0.135239107342+0.130886652334i, 0.734470414137+0.597958688522i]}, {"Frequency"=3793180375.0, "S Parameters"=[0.656874541373+0.687014893276i, -0.133064206182+0.132110728041i, -0.134052121756+0.131497751437i, 0.738466784557+0.592748225992i]}, {"Frequency"=3798492812.5, "S Parameters"=[0.660971869642+0.68306735476i, -0.131966706593+0.132712659036i, -0.132924839215+0.132098906504i, 0.742594099892+0.587527034508i]}, {"Frequency"=3803805250.0, "S Parameters"=[0.665040399292+0.679052676912i, -0.130832121952+0.133276869872i, -0.131778975409+0.132702322452i, 0.746583574359+0.582157267045i]}, {"Frequency"=3809117687.5, "S Parameters"=[0.669049471755+0.675161410377i, -0.129679874779+0.133862306i, -0.130645969896+0.133310053729i, 0.750688809324+0.57674818688i]}, {"Frequency"=3814430125.0, "S Parameters"=[0.673144808285+0.671240724833i, -0.128575571437+0.134439429182i, -0.129505168114+0.133879254174i, 0.754953344215+0.571503322923i]}, {"Frequency"=3819742562.5, "S Parameters"=[0.677228756962+0.667409779366i, -0.127423730069+0.13503272559i, -0.128376389176+0.134492133122i, 0.759133034395+0.566189161338i]}, {"Frequency"=3825055000.0, "S Parameters"=[0.681309858151+0.663481921753i, -0.126319901254+0.135636644955i, -0.127272116222+0.135084145582i, 0.763457940643+0.561045295324i]}, {"Frequency"=3830367437.5, "S Parameters"=[0.685182720145+0.659618451444i, -0.125153443059+0.136220099902i, -0.126151924979+0.135644542501i, 0.767325947468+0.555965370819i]}, {"Frequency"=3835679875.0, "S Parameters"=[0.68916340033+0.655475251537i, -0.124098973472+0.136821174409i, -0.125081921497+0.136210478487i, 0.771332802887+0.550901352874i]}, {"Frequency"=3840992312.5, "S Parameters"=[0.693221153534+0.651132665176i, -0.122944048351+0.137419944085i, -0.123942154498+0.136803741964i, 0.775169243261+0.545607924121i]}, {"Frequency"=3846304750.0, "S Parameters"=[0.697306628029+0.646522403237i, -0.121824944116+0.137986834037i, -0.122789366388+0.13732281701i, 0.778868098604+0.540518683766i]}, {"Frequency"=3851617187.5, "S Parameters"=[0.701507829009+0.641764826867i, -0.120691247189+0.13852075495i, -0.121608574721+0.137832246973i, 0.782450679045+0.535353971979i]}, {"Frequency"=3856929625.0, "S Parameters"=[0.705839640326+0.636951030748i, -0.119509065059+0.139052361105i, -0.120421141667+0.138355346437i, 0.786148785269+0.530086998915i]}, {"Frequency"=3862242062.5, "S Parameters"=[0.710307845362+0.631925455685i, -0.118299107487+0.139559626876i, -0.119187028045+0.138861877548i, 0.78968015389+0.524901476655i]}, {"Frequency"=3867554500.0, "S Parameters"=[0.71496135568+0.626900064558i, -0.11709361968+0.140063261981i, -0.117956703518+0.139367987531i, 0.793221666316+0.519728761911i]}, {"Frequency"=3872866937.5, "S Parameters"=[0.719478674836+0.621707781381i, -0.115844424766+0.140514862613i, -0.116702237392+0.139884502527i, 0.796559627206+0.514566578135i]}, {"Frequency"=3878179375.0, "S Parameters"=[0.723896419748+0.61638884254i, -0.114624034238+0.140967480303i, -0.11541889359+0.140328652727i, 0.799937316325+0.509293509011i]}, {"Frequency"=3883491812.5, "S Parameters"=[0.7283958439+0.610940844948i, -0.113394206676+0.141409374409i, -0.114142157256+0.140815200581i, 0.803169464895+0.504044206147i]}, {"Frequency"=3888804250.0, "S Parameters"=[0.732771637015+0.605447455409i, -0.112154523675+0.141824955365i, -0.112900158844+0.141299820415i, 0.806341350727+0.498522951083i]}, {"Frequency"=3894116687.5, "S Parameters"=[0.737040917063+0.600034149083i, -0.110912999704+0.142198739334i, -0.111642021553+0.141692632259i, 0.809341379451+0.493057137543i]}, {"Frequency"=3899429125.0, "S Parameters"=[0.741604733191+0.594687732858i, -0.109715915336+0.142571747228i, -0.110406612264+0.142092761255i, 0.812649117498+0.487662851206i]}, {"Frequency"=3904741562.5, "S Parameters"=[0.745835685238+0.589537956298i, -0.108534000539+0.142917111842i, -0.109178250676+0.142400112943i, 0.816001508162+0.482300974842i]}, {"Frequency"=3910054000.0, "S Parameters"=[0.750088394983+0.584651019962i, -0.107350283893+0.143266884467i, -0.107975612309+0.142725376921i, 0.819233675665+0.477013879804i]}, {"Frequency"=3915366437.5, "S Parameters"=[0.754174712011+0.57979854514i, -0.106176136996+0.143587797932i, -0.106821892967+0.143054086265i, 0.822636430717+0.471867566512i]}, {"Frequency"=3920678875.0, "S Parameters"=[0.758082099713+0.575029967227i, -0.105006484735+0.143931864512i, -0.105630047773+0.143340435562i, 0.825829832693+0.466612193116i]}, {"Frequency"=3925991312.5, "S Parameters"=[0.761836518101+0.570146516025i, -0.10384702787+0.144279701065i, -0.104446927118+0.143635909171i, 0.828958561843+0.461226508338i]}, {"Frequency"=3931303750.0, "S Parameters"=[0.765504939888+0.565230316025i, -0.102697906303+0.144613360352i, -0.103281004899+0.14391987701i, 0.831936434121+0.455943688473i]}, {"Frequency"=3936616187.5, "S Parameters"=[0.769094999515+0.560265554293i, -0.101573024674+0.144938350618i, -0.102115034206+0.144188502204i, 0.83496447939+0.450420721073i]}, {"Frequency"=3941928625.0, "S Parameters"=[0.77272684391+0.55534723751i, -0.100418871736+0.14524070689i, -0.100951933509+0.144445284976i, 0.837975252033+0.444764659083i]}, {"Frequency"=3947241062.5, "S Parameters"=[0.77632466688+0.550490688964i, -0.0992650968707+0.145503792603i, -0.099812721352+0.144675563665i, 0.840864626651+0.43930400619i]}, {"Frequency"=3952553500.0, "S Parameters"=[0.779998647708+0.545691511535i, -0.0981287511199+0.145762682494i, -0.0987063369745+0.144914004765i, 0.843764879389+0.433892772025i]}, {"Frequency"=3957865937.5, "S Parameters"=[0.783389162236+0.540689252242i, -0.0969727624289+0.146031336441i, -0.0975551353529+0.145174988697i, 0.846647321761+0.428427628614i]}, {"Frequency"=3963178375.0, "S Parameters"=[0.786885208723+0.535683265205i, -0.0958286268493+0.146263441671i, -0.0964343502136+0.145428565134i, 0.849171660638+0.422994608358i]}, {"Frequency"=3968490812.5, "S Parameters"=[0.790240071518+0.530503397117i, -0.0946883223316+0.146483579985i, -0.0953003975696+0.145688448152i, 0.851848486417+0.417409107205i]}, {"Frequency"=3973803250.0, "S Parameters"=[0.793569654693+0.525265168413i, -0.0935309698913+0.146722706463i, -0.0941570256962+0.145975889765i, 0.854382347948+0.411790904673i]}, {"Frequency"=3979115687.5, "S Parameters"=[0.796969929501+0.519806633219i, -0.0924181988761+0.146942930038i, -0.0930395934538+0.146251414162i, 0.856805690934+0.406153281729i]}, {"Frequency"=3984428125.0, "S Parameters"=[0.800344192768+0.514404759713i, -0.0912949200982+0.147182900629i, -0.0919113685464+0.146511795502i, 0.859256272068+0.40035860948i]}, {"Frequency"=3989740562.5, "S Parameters"=[0.803880754619+0.508962902192i, -0.0901748393424+0.147386316636i, -0.0907778729415+0.146814363599i, 0.861886909247+0.394615172461i]}, {"Frequency"=3995053000.0, "S Parameters"=[0.807327931414+0.503920954056i, -0.089083107309+0.147587508803i, -0.0896651968004+0.147017232293i, 0.864486183134+0.388970699215i]}, {"Frequency"=4000365437.5, "S Parameters"=[0.810715821067+0.498997479249i, -0.088004340504+0.147774555439i, -0.0885693788158+0.147206535505i, 0.867228982003+0.383555875015i]}, {"Frequency"=4005677875.0, "S Parameters"=[0.813846784278+0.494139986446i, -0.0869392514269+0.148001028235i, -0.087446138385+0.147375104607i, 0.869893059203+0.37801245398i]}, {"Frequency"=4010990312.5, "S Parameters"=[0.816991718248+0.489222944375i, -0.0858132863592+0.148199051883i, -0.0863251052583+0.147570972449i, 0.872342348802+0.372492699669i]}, {"Frequency"=4016302750.0, "S Parameters"=[0.819859266593+0.484173244197i, -0.0847443733596+0.1484016856i, -0.085181586639+0.147720992747i, 0.874871726765+0.366988677274i]}, {"Frequency"=4021615187.5, "S Parameters"=[0.822729730909+0.479066521303i, -0.0836589899774+0.148558324885i, -0.0840608205722+0.147863135954i, 0.877255082745+0.361272877085i]}, {"Frequency"=4026927625.0, "S Parameters"=[0.825717621109+0.473908501412i, -0.0825667625824+0.148772994607i, -0.0829129772942+0.148065214336i, 0.879483137738+0.355235191237i]}, {"Frequency"=4032240062.5, "S Parameters"=[0.828621660504+0.468624292891i, -0.0814910889978+0.148933390549i, -0.0817675247966+0.148205655856i, 0.88178949544+0.349327808182i]}, {"Frequency"=4037552500.0, "S Parameters"=[0.831611679214+0.463413238004i, -0.0803865695681+0.149121503037i, -0.0806553016999+0.148341167928i, 0.884254339025+0.343371035898i]}, {"Frequency"=4042864937.5, "S Parameters"=[0.834665802248+0.458220464789i, -0.079300493479+0.149282600681i, -0.0795485345892+0.148510341003i, 0.88650500459+0.337528829209i]}, {"Frequency"=4048177375.0, "S Parameters"=[0.837483812557+0.452984996557i, -0.0782535180216+0.149453374105i, -0.0784882993047+0.148664396201i, 0.888727655271+0.331721338409i]}, {"Frequency"=4053489812.5, "S Parameters"=[0.840355006898+0.447493505157i, -0.0771902721082+0.149615990991i, -0.077438554933+0.148834432957i, 0.890816942197+0.325890254749i]}, {"Frequency"=4058802250.0, "S Parameters"=[0.843263115925+0.441948622093i, -0.0761523906175+0.149777385735i, -0.0764314258895+0.14904059604i, 0.892868219472+0.320083038363i]}, {"Frequency"=4064114687.5, "S Parameters"=[0.846011656017+0.436175233872i, -0.0750418354677+0.149977776747i, -0.0753782954983+0.149232274291i, 0.89463725522+0.313991727654i]}, {"Frequency"=4069427125.0, "S Parameters"=[0.848977061677+0.430121389979i, -0.0739490087322+0.150168417092i, -0.0743084992669+0.149445019758i, 0.896587789669+0.307868538172i]}, {"Frequency"=4074739562.5, "S Parameters"=[0.851893576695+0.423896015145i, -0.0728204534781+0.150348473874i, -0.0731955592324+0.149661225886i, 0.898468027476+0.301608791525i]}, {"Frequency"=4080052000.0, "S Parameters"=[0.855091954136+0.417629637186i, -0.0716921233522+0.150587826434i, -0.0720785945096+0.149886214989i, 0.900527506814+0.295092917289i]}, {"Frequency"=4085364437.5, "S Parameters"=[0.858339439506+0.411357338589i, -0.0705459971022+0.15076673566i, -0.0709366380217+0.150102495525i, 0.902607501726+0.288821893547i]}, {"Frequency"=4090676875.0, "S Parameters"=[0.861413589857+0.405251341082i, -0.069369550676+0.150944087049i, -0.0697761156557+0.150228894946i, 0.904804704478+0.282429845085i]}, {"Frequency"=4095989312.5, "S Parameters"=[0.864389933848+0.399224806675i, -0.0682039865506+0.151088946557i, -0.0686140057956+0.150347263115i, 0.906864405774+0.276159670934i]}, {"Frequency"=4101301750.0, "S Parameters"=[0.867106714051+0.393175863148i, -0.0670395915083+0.151168347032i, -0.0674300619153+0.15046191548i, 0.908710906913+0.270042573361i]}, {"Frequency"=4106614187.5, "S Parameters"=[0.86982806026+0.387041550335i, -0.06587179981+0.151205203495i, -0.0662221921848+0.150458144523i, 0.910568847353+0.263713403624i]}, {"Frequency"=4111926625.0, "S Parameters"=[0.872377034401+0.380780369289i, -0.06470321+0.151239250333i, -0.0650022154952+0.150499341878i, 0.912263575477+0.257159822846i]}, {"Frequency"=4117239062.5, "S Parameters"=[0.875031359393+0.374556870059i, -0.063525133257+0.151251205108i, -0.0637795664593+0.150505173222i, 0.91398040721+0.250406949952i]}, {"Frequency"=4122551500.0, "S Parameters"=[0.877602942251+0.368298818858i, -0.0623312950293+0.151233106561i, -0.0625144626089+0.150526081293i, 0.915680533569+0.243549107092i]}, {"Frequency"=4127863937.5, "S Parameters"=[0.880182407212+0.362372231098i, -0.0611375039667+0.151181256193i, -0.0613163367321+0.15051893339i, 0.917463279403+0.236706488427i]}, {"Frequency"=4133176375.0, "S Parameters"=[0.882562840992+0.356597654901i, -0.0600222326028+0.151147007267i, -0.0601111991474+0.150467256361i, 0.919408639177+0.230094048076i]}, {"Frequency"=4138488812.5, "S Parameters"=[0.884854343269+0.350888128492i, -0.0588967119818+0.151068858743i, -0.0589427356121+0.150400913536i, 0.921073498505+0.223527738587i]}, {"Frequency"=4143801250.0, "S Parameters"=[0.887224951861+0.345326909485i, -0.0578158174581+0.150950078289i, -0.0578438011988+0.150349523051i, 0.922721822959+0.217049532256i]}, {"Frequency"=4149113687.5, "S Parameters"=[0.889292841719+0.33991899162i, -0.0566955881346+0.150875903315i, -0.0567480624835+0.150240972024i, 0.924133213667+0.210668137313i]}, {"Frequency"=4154426125.0, "S Parameters"=[0.891270693714+0.334570487129i, -0.0556741645044+0.150758545589i, -0.0557250378972+0.150155029146i, 0.925487425107+0.204343383433i]}, {"Frequency"=4159738562.5, "S Parameters"=[0.89337470986+0.329049335965i, -0.054652254352+0.15065086028i, -0.0547241860529+0.150048419437i, 0.926827304433+0.19785127636i]}, {"Frequency"=4165051000.0, "S Parameters"=[0.895447258541+0.323414170622i, -0.0536076631319+0.150570365875i, -0.0537237669595+0.149914613159i, 0.92818054539+0.191413441033i]}, {"Frequency"=4170363437.5, "S Parameters"=[0.897641490669+0.317842936829i, -0.0526020934595+0.150485991647i, -0.0526921226418+0.149811198759i, 0.929689148223+0.185149296082i]}, {"Frequency"=4175675875.0, "S Parameters"=[0.899729585946+0.31227692698i, -0.0516200425453+0.150428676402i, -0.0517386090656+0.149713554239i, 0.931153496738+0.178690458335i]}, {"Frequency"=4180988312.5, "S Parameters"=[0.901831566405+0.306723194479i, -0.0505999282982+0.150360786978i, -0.0507276514617+0.14959582887i, 0.932585974193+0.172501412358i]}, {"Frequency"=4186300750.0, "S Parameters"=[0.903736970481+0.301173321119i, -0.0496286775986+0.150286146162i, -0.0497414070795+0.149498757904i, 0.933824099369+0.166524992989i]}, {"Frequency"=4191613187.5, "S Parameters"=[0.905412376554+0.295396806057i, -0.0486764932719+0.150200580253i, -0.0487466402852+0.149378101256i, 0.934878540389+0.160562169243i]}, {"Frequency"=4196925625.0, "S Parameters"=[0.907128708844+0.289547656359i, -0.0476695044032+0.150121666697i, -0.0477817080823+0.14929280924i, 0.935747086493+0.154562046741i]}, {"Frequency"=4202238062.5, "S Parameters"=[0.908750358203+0.283550377972i, -0.0467107119855+0.150006104818i, -0.0467892371764+0.149205240381i, 0.936414102852+0.148635814125i]}, {"Frequency"=4207550500.0, "S Parameters"=[0.910349840512+0.277195556671i, -0.0457234766078+0.14990198322i, -0.0457669151056+0.149145453557i, 0.937027681866+0.142583189522i]}, {"Frequency"=4212862937.5, "S Parameters"=[0.912123711848+0.271018504727i, -0.0447350239787+0.149803744851i, -0.0448013747537+0.149040454001i, 0.937631854728+0.136359381329i]}, {"Frequency"=4218175375.0, "S Parameters"=[0.913945290692+0.264710615256i, -0.0437536236277+0.14971282195i, -0.0438350700686+0.149028107144i, 0.938306746927+0.130249384665i]}, {"Frequency"=4223487812.5, "S Parameters"=[0.915684977203+0.258335792156i, -0.0427354751907+0.149670316754i, -0.0428154808879+0.149004238155i, 0.939049678476+0.12405621918i]}, {"Frequency"=4228800250.0, "S Parameters"=[0.917331920439+0.252060919781i, -0.0417377350606+0.149558032697i, -0.0418197050445+0.148940871798i, 0.939813430449+0.118194957746i]}, {"Frequency"=4234112687.5, "S Parameters"=[0.919081515816+0.245607261962i, -0.0407689929668+0.149502633179i, -0.0408162954376+0.148926860241i, 0.940541058144+0.112064633546i]}, {"Frequency"=4239425125.0, "S Parameters"=[0.920732718418+0.239192210253i, -0.0397524357831+0.14944981993i, -0.0398215173139+0.14891571935i, 0.941296770645+0.105985979282i]}, {"Frequency"=4244737562.5, "S Parameters"=[0.92240746578+0.232957226216i, -0.0387704876977+0.149407226622i, -0.0388440934554+0.148876528342i, 0.941877948071+0.0998916583037i]}, {"Frequency"=4250050000.0, "S Parameters"=[0.923982157741+0.226584355623i, -0.0377725822546+0.14938260934i, -0.0378635859352+0.148845486434i, 0.942520085857+0.0938562659606i]}, {"Frequency"=4255362437.5, "S Parameters"=[0.92566806218+0.220219168048i, -0.036733900411+0.14933979273i, -0.0368646695858+0.148825691606i, 0.943163992474+0.087683228664i]}, {"Frequency"=4260674875.0, "S Parameters"=[0.927324305382+0.213808531156i, -0.0356762692828+0.149319342589i, -0.0357488475904+0.148766104318i, 0.944031937212+0.081434682371i]}, {"Frequency"=4265987312.5, "S Parameters"=[0.929021903095+0.207531781821i, -0.0345542670009+0.149227810953i, -0.0346329526144+0.148667721316i, 0.944859567929+0.0750899833063i]}, {"Frequency"=4271299750.0, "S Parameters"=[0.9306633358+0.201266075211i, -0.0334074089092+0.14912100425i, -0.0335111653755+0.148559603771i, 0.945570128724+0.0687906679269i]}, {"Frequency"=4276612187.5, "S Parameters"=[0.932107878526+0.194974285787i, -0.0323006853506+0.148951461496i, -0.0323392511555+0.148361746729i, 0.946375067754+0.06273134678i]}, {"Frequency"=4281924625.0, "S Parameters"=[0.933418353233+0.188577080252i, -0.0311444784759+0.148725502081i, -0.0311943277104+0.14815431759i, 0.946970557152+0.0567579595623i]}, {"Frequency"=4287237062.5, "S Parameters"=[0.934736313373+0.182246543402i, -0.0300334769517+0.148497418976i, -0.0300542607486+0.14790815101i, 0.947325751867+0.0507034144837i]}, {"Frequency"=4292549500.0, "S Parameters"=[0.93598029322+0.175827032369i, -0.0289597016882+0.148191265917i, -0.0289316408843+0.147584226216i, 0.947686949694+0.0446628824584i]}, {"Frequency"=4297861937.5, "S Parameters"=[0.937183465588+0.169409910041i, -0.0278942105481+0.147867777953i, -0.0278396031471+0.147295658792i, 0.947802148331+0.0385371263697i]}, {"Frequency"=4303174375.0, "S Parameters"=[0.938437221127+0.163018909042i, -0.0268345631308+0.14753934143i, -0.0267977045377+0.146988418664i, 0.948053864453+0.0324571281467i]}, {"Frequency"=4308486812.5, "S Parameters"=[0.939654680596+0.15665123596i, -0.0258590391548+0.147221171866i, -0.0257966380878+0.146664632303i, 0.948301567633+0.0264106405853i]}, {"Frequency"=4313799250.0, "S Parameters"=[0.940753956646+0.150251796326i, -0.0248511587458+0.146867256157i, -0.0247796202607+0.146359013339i, 0.94859364073+0.0202820335105i]}, {"Frequency"=4319111687.5, "S Parameters"=[0.941837536083+0.143843094285i, -0.0239016976211+0.14651324319i, -0.0238326756793+0.145996939578i, 0.948794391582+0.0141621379308i]}, {"Frequency"=4324424125.0, "S Parameters"=[0.942916917543+0.137460922715i, -0.0229399386712+0.146174353556i, -0.0228716711786+0.14566768758i, 0.948880540739+0.00803226062228i]}, {"Frequency"=4329736562.5, "S Parameters"=[0.943900494564+0.13106514041i, -0.0219804744497+0.145863342423i, -0.021931306975+0.145337009966i, 0.948911232981+0.0017421134033i]}, {"Frequency"=4335049000.0, "S Parameters"=[0.944857776074+0.124732098737i, -0.0210712282112+0.145523810457i, -0.0210083722526+0.145005973279i, 0.94894332141-0.00453282812385i]}, {"Frequency"=4340361437.5, "S Parameters"=[0.945690834833+0.118455486505i, -0.0201533299102+0.145169779856i, -0.0200894807611+0.144662757648i, 0.948934561145-0.0107578617853i]}, {"Frequency"=4345673875.0, "S Parameters"=[0.946512578332+0.112225496186i, -0.0192354494342+0.144878908222i, -0.0191848245286+0.14434309239i, 0.948765903272-0.0172811229952i]}, {"Frequency"=4350986312.5, "S Parameters"=[0.947258421994+0.106142664704i, -0.0183467512398+0.144552761319i, -0.0182998162195+0.144039689523i, 0.948680410845-0.0236924006431i]}, {"Frequency"=4356298750.0, "S Parameters"=[0.948023173437+0.100134500101i, -0.0174512603853+0.144203107463i, -0.0174195238977+0.143715712684i, 0.948512538731-0.0301597337526i]}, {"Frequency"=4361611187.5, "S Parameters"=[0.948636922216+0.094261337171i, -0.0165603333242+0.143852695211i, -0.016502226644+0.143365772486i, 0.948418965829-0.0365449761777i]}, {"Frequency"=4366923625.0, "S Parameters"=[0.949320052968+0.0883935226201i, -0.0156681977641+0.143514322562i, -0.0156275914684+0.143042102552i, 0.948123599283-0.0430028324032i]}, {"Frequency"=4372236062.5, "S Parameters"=[0.949800839567+0.0824289785239i, -0.0147831743161+0.143130164549i, -0.0147394615483+0.14269626772i, 0.947778117387-0.0493950389654i]}, {"Frequency"=4377548500.0, "S Parameters"=[0.950214925755+0.0764712149342i, -0.0139227166815+0.142746173141i, -0.0138582917062+0.142350139647i, 0.947311002687-0.055792371225i]}, {"Frequency"=4382860937.5, "S Parameters"=[0.950588861071+0.0704410714646i, -0.0130887038433+0.142382217614i, -0.0129763732253+0.142029538838i, 0.946769525297-0.0623171112408i]}, {"Frequency"=4388173375.0, "S Parameters"=[0.950992330639+0.0644130428504i, -0.0122606107989+0.14200362428i, -0.0121519280611+0.141676403705i, 0.946211031965-0.068805339929i]}, {"Frequency"=4393485812.5, "S Parameters"=[0.951376465135+0.0583484429243i, -0.0114354693304+0.141651480274i, -0.011323363864+0.141359088306i, 0.945644754923-0.0752806252567i]}, {"Frequency"=4398798250.0, "S Parameters"=[0.951664752317+0.0522124333985i, -0.0106194655683+0.141314154409i, -0.0105036572128+0.141000067695i, 0.945102223568-0.0816216232165i]}, {"Frequency"=4404110687.5, "S Parameters"=[0.951994934234+0.0461026273143i, -0.0098503358985+0.14093393645i, -0.00971060755067+0.140647297279i, 0.944547438158-0.0878120787759i]}, {"Frequency"=4409423125.0, "S Parameters"=[0.952133744042+0.0397560604146i, -0.00905442358361+0.140553103703i, -0.00891196040108+0.140275065123i, 0.943946353422-0.0940572296063i]}, {"Frequency"=4414735562.5, "S Parameters"=[0.952379876009+0.0333309535545i, -0.00830326975206+0.140212155047i, -0.00813171256282+0.139929151841i, 0.943282779327-0.100224428505i]}, {"Frequency"=4420048000.0, "S Parameters"=[0.952557731135+0.0267057280161i, -0.00751958950035+0.139890658526i, -0.00732621493888+0.139603262987i, 0.942653382024-0.106505940796i]}, {"Frequency"=4425360437.5, "S Parameters"=[0.952669974603+0.0201007225109i, -0.00676922958257+0.13960121243i, -0.00649908168296+0.139264886267i, 0.941962623816-0.112575283277i]}, {"Frequency"=4430672875.0, "S Parameters"=[0.952652974509+0.0132294177987i, -0.00595144308275+0.139308835956i, -0.00564390610553+0.138923306265i, 0.941168752263-0.118774406243i]}, {"Frequency"=4435985312.5, "S Parameters"=[0.952725943504+0.00643367729874i, -0.00513267037642+0.139015975387i, -0.0048106510777+0.138612378518i, 0.940314811217-0.124965508407i]}, {"Frequency"=4441297750.0, "S Parameters"=[0.95274241751-0.000313969150566i, -0.00433024124054+0.138710998297i, -0.00397654647849+0.138242276995i, 0.93958529972-0.131090944119i]}, {"Frequency"=4446610187.5, "S Parameters"=[0.95260175505-0.00715024074228i, -0.00349417457254+0.138399926912i, -0.00317347695889+0.137919062842i, 0.938752036714-0.137162559991i]}, {"Frequency"=4451922625.0, "S Parameters"=[0.95247493163-0.0137733427494i, -0.0026913886949+0.138098472032i, -0.00236577646838+0.13758513455i, 0.937926229068-0.143106824405i]}, {"Frequency"=4457235062.5, "S Parameters"=[0.952440574967-0.0204468643089i, -0.00182068227345+0.137770782246i, -0.00153843757877+0.137287764837i, 0.937070497583-0.149053667269i]}, {"Frequency"=4462547500.0, "S Parameters"=[0.952298405733-0.0271099440516i, -0.00092555619956+0.137396267914i, -0.00065203376853+0.13694205752i, 0.93598649598-0.155027121319i]}, {"Frequency"=4467859937.5, "S Parameters"=[0.952118700813-0.0336395468013i, -2.81139298593e-05+0.13697674168i, 0.000195897784946+0.136603569803i, 0.934931235442-0.161026165935i]}, {"Frequency"=4473172375.0, "S Parameters"=[0.951966577658-0.0401309982118i, 0.000832048015369+0.136590777372i, 0.00103272062412+0.136238221144i, 0.933799004903-0.16721430597i]}, {"Frequency"=4478484812.5, "S Parameters"=[0.951679679808-0.0464924339438i, 0.00170167723125+0.136158808216i, 0.00187948609725+0.13584784936i, 0.932668326373-0.173400589207i]}, {"Frequency"=4483797250.0, "S Parameters"=[0.951503872076-0.0528005805264i, 0.00255867693957+0.13574196581i, 0.002708648005+0.135479494566i, 0.931380090002-0.179642800931i]}, {"Frequency"=4489109687.5, "S Parameters"=[0.951362785414-0.0588972013349i, 0.00336644057385+0.135346554557i, 0.00349778514797+0.135100291322i, 0.930241719352-0.185800871161i]}, {"Frequency"=4494422125.0, "S Parameters"=[0.95108932788-0.0650733794219i, 0.0041924770536+0.134932253625i, 0.00431179238652+0.134688545508i, 0.929064253316-0.192001735563i]}, {"Frequency"=4499734562.5, "S Parameters"=[0.950843009171-0.0710486362823i, 0.00498230235385+0.134516651839i, 0.00511410825226+0.1343107831i, 0.927938872763-0.198174855045i]}, {"Frequency"=4505047000.0, "S Parameters"=[0.950462397104-0.0769122726115i, 0.00576285135114+0.134100633787i, 0.00589141384667+0.13389369484i, 0.926667757008-0.204304522392i]}, {"Frequency"=4510359437.5, "S Parameters"=[0.950071219315-0.0830186501916i, 0.0065639555728+0.133672474182i, 0.00674353014459+0.133461799966i, 0.925520884128-0.210557206315i]}, {"Frequency"=4515671875.0, "S Parameters"=[0.949590489473-0.0891619858612i, 0.0073527588188+0.133219704921i, 0.00757718232025+0.133008950805i, 0.924178950486-0.216856601649i]}, {"Frequency"=4520984312.5, "S Parameters"=[0.949085469744-0.0953339352583i, 0.00815666000023+0.132794139416i, 0.0084268243097+0.132570912458i, 0.922880005174-0.2232742038i]}, {"Frequency"=4526296750.0, "S Parameters"=[0.948477577071-0.101624595491i, 0.00900889513227+0.132357569631i, 0.00929288102047+0.132108299291i, 0.92146230598-0.229614081735i]}, {"Frequency"=4531609187.5, "S Parameters"=[0.947665413596-0.108131349272i, 0.00986151451447+0.131888688694i, 0.010162766862+0.13163142036i, 0.920053106739-0.235968662525i]}, {"Frequency"=4536921625.0, "S Parameters"=[0.94678989897-0.11458182645i, 0.0106885679992+0.131381089105i, 0.0109942499455+0.131115401359i, 0.918503096892-0.242251580319i]}, {"Frequency"=4542234062.5, "S Parameters"=[0.946019432962-0.121277004031i, 0.0115203068752+0.130860302643i, 0.0118529705666+0.130590957384i, 0.916935463416-0.248548712291i]}, {"Frequency"=4547546500.0, "S Parameters"=[0.945119475022-0.12800910953i, 0.0123254963088+0.130314208661i, 0.012683728004+0.130030539255i, 0.915332874409-0.254792019107i]}, {"Frequency"=4552858937.5, "S Parameters"=[0.944180431749-0.134590197198i, 0.0131173275558+0.129718071141i, 0.013464891001+0.129455936478i, 0.913504700251-0.26090626442i]}, {"Frequency"=4558171375.0, "S Parameters"=[0.943252121084-0.141364738289i, 0.0139300787704+0.129118387008i, 0.0142481276022+0.12886974337i, 0.911801979583-0.26716498063i]}, {"Frequency"=4563483812.5, "S Parameters"=[0.942342797214-0.148109083308i, 0.014742271568+0.128500295475i, 0.0150173664096+0.128273415855i, 0.90995128635-0.273472300003i]}, {"Frequency"=4568796250.0, "S Parameters"=[0.941384072675-0.154744799491i, 0.0154788185042+0.127858340755i, 0.0157312735418+0.127667081547i, 0.907924516272-0.279710126789i]}, {"Frequency"=4574108687.5, "S Parameters"=[0.940443309994-0.16124256243i, 0.0162001270465+0.127196502339i, 0.0164443990031+0.127032340566i, 0.905952390272-0.285935868005i]}, {"Frequency"=4579421125.0, "S Parameters"=[0.939395856024-0.167756894479i, 0.0169107502605+0.126562533768i, 0.0171461078647+0.126393393268i, 0.903974138072-0.292350571505i]}, {"Frequency"=4584733562.5, "S Parameters"=[0.938330677294-0.173992585419i, 0.017568639349+0.125907882803i, 0.0177928396754+0.125723481667i, 0.9018523083-0.298642091289i]}, {"Frequency"=4590046000.0, "S Parameters"=[0.937418466057-0.180084697267i, 0.0181989697054+0.125264786i, 0.0184294745635+0.125083977521i, 0.899853926055-0.304904739691i]}, {"Frequency"=4595358437.5, "S Parameters"=[0.936359512757-0.186105650839i, 0.018765955858+0.124653669039i, 0.0190047546707+0.124454822611i, 0.897835978393-0.311050510291i]}, {"Frequency"=4600670875.0, "S Parameters"=[0.935417150199-0.191873905356i, 0.0193002558932+0.124056331235i, 0.0195336878839+0.123882313427i, 0.895739105815-0.317140643412i]}, {"Frequency"=4605983312.5, "S Parameters"=[0.934396155512-0.197514997214i, 0.0198185900188+0.123487889201i, 0.0200831364801+0.123337097968i, 0.893685308986-0.323092341117i]}, {"Frequency"=4611295750.0, "S Parameters"=[0.933317562026-0.203068018435i, 0.0203593542052+0.122960190033i, 0.0206200146969+0.122787253871i, 0.891759605535-0.329159543125i]}, {"Frequency"=4616608187.5, "S Parameters"=[0.932119090145-0.208573886855i, 0.0209192722709+0.122402904961i, 0.0211987420677+0.122288689077i, 0.889681655222-0.33509191894i]}, {"Frequency"=4621920625.0, "S Parameters"=[0.930591745164-0.214206407928i, 0.0215045970631+0.121898745823i, 0.021783286424+0.121756283701i, 0.887497229236-0.340810384969i]}, {"Frequency"=4627233062.5, "S Parameters"=[0.929065969517-0.21997725022i, 0.0220694063028+0.121339205318i, 0.0223702023141+0.121232741021i, 0.885337881986-0.346469181807i]}, {"Frequency"=4632545500.0, "S Parameters"=[0.927591711462-0.225778104039i, 0.0226741552761+0.120782322499i, 0.0229603049198+0.120722448416i, 0.883069479406-0.352120233479i]}, {"Frequency"=4637857937.5, "S Parameters"=[0.926015204605-0.23181868331i, 0.0232770118261+0.120247205607i, 0.0235687695362+0.120185069331i, 0.880876852143-0.357747355705i]}, {"Frequency"=4643170375.0, "S Parameters"=[0.924409179617-0.237950006994i, 0.0238941384246+0.119695270367i, 0.0242013157889+0.119655090529i, 0.878742204714-0.363222957803i]}, {"Frequency"=4648482812.5, "S Parameters"=[0.922787538851-0.244062476627i, 0.0244833494702+0.119141002582i, 0.024780805137+0.119099078577i, 0.876506703795-0.368685846518i]}, {"Frequency"=4653795250.0, "S Parameters"=[0.921094865689-0.250331217305i, 0.0250747849198+0.118599090668i, 0.0253749440774+0.118586624494i, 0.874226103357-0.374034298335i]}, {"Frequency"=4659107687.5, "S Parameters"=[0.919310305144-0.256560694958i, 0.0256692832598+0.118035106013i, 0.0259823040963+0.118001237694i, 0.871874135343-0.379387491788i]}, {"Frequency"=4664420125.0, "S Parameters"=[0.917315599913-0.263026723165i, 0.0262607637213+0.117470634571i, 0.0265951926219+0.117439319892i, 0.869401413627-0.384875245507i]}, {"Frequency"=4669732562.5, "S Parameters"=[0.915451973043-0.269509449147i, 0.0268792515825+0.116886632764i, 0.0272306617991+0.116822704915i, 0.866780928471-0.390413611485i]}, {"Frequency"=4675045000.0, "S Parameters"=[0.913597870117-0.276054909749i, 0.0274632543118+0.116293122952i, 0.0278673750127+0.116235939861i, 0.864061734543-0.396009658056i]}, {"Frequency"=4680357437.5, "S Parameters"=[0.911612852529-0.28254408864i, 0.0280633757674+0.11568519651i, 0.0285002326805+0.115611300888i, 0.86125099075-0.401824299246i]}, {"Frequency"=4685669875.0, "S Parameters"=[0.909703433041-0.288976602927i, 0.0286360506874+0.115111841077i, 0.0291050410293+0.115026978224i, 0.858404274134-0.407718512202i]}, {"Frequency"=4690982312.5, "S Parameters"=[0.907924789336-0.295220597919i, 0.029173009797+0.114490092713i, 0.0296785266379+0.114400307143i, 0.855509030969-0.41362316422i]}, {"Frequency"=4696294750.0, "S Parameters"=[0.906193829209-0.301441187574i, 0.0297346066756+0.113875691138i, 0.0302482982257+0.113746527321i, 0.852478738544-0.419817968881i]}, {"Frequency"=4701607187.5, "S Parameters"=[0.90448277238-0.307352257911i, 0.0302591547072+0.113231673167i, 0.0307511426605+0.113098757719i, 0.849428229538-0.42581590421i]}, {"Frequency"=4706919625.0, "S Parameters"=[0.902548154432-0.313086491939i, 0.0307776929549+0.112585646623i, 0.0312491297251+0.1124626107i, 0.846350137032-0.43184901894i]}, {"Frequency"=4712232062.5, "S Parameters"=[0.900516389757-0.318843105105i, 0.0312704553171+0.111931250126i, 0.031697740978+0.111779894467i, 0.843166733268-0.437995301534i]}, {"Frequency"=4717544500.0, "S Parameters"=[0.898412720756-0.324544617956i, 0.0317990921911+0.111236974952i, 0.0321469019759+0.111107904985i, 0.839690224846-0.444165717582i]}, {"Frequency"=4722856937.5, "S Parameters"=[0.896177219326-0.330438396877i, 0.0322879437543+0.110576692458i, 0.0325913393152+0.110430473765i, 0.836387283059-0.450489191688i]}, {"Frequency"=4728169375.0, "S Parameters"=[0.89417325403-0.336177383599i, 0.0327745623505+0.109842771025i, 0.0330274620703+0.109729071505i, 0.83292414276-0.456714871312i]}, {"Frequency"=4733481812.5, "S Parameters"=[0.892121910882-0.341941980197i, 0.0332114792236+0.109152687849i, 0.0334219413806+0.109058643719i, 0.829623495554-0.462953601605i]}, {"Frequency"=4738794250.0, "S Parameters"=[0.889982470455-0.347686518168i, 0.0336289128043+0.108476354677i, 0.0337909884926+0.108399159558i, 0.826352608219-0.469054286178i]}, {"Frequency"=4744106687.5, "S Parameters"=[0.887822486355-0.353209335658i, 0.0339722280131+0.107847151453i, 0.034123260326+0.10776374481i, 0.823121010945-0.474916873033i]}, {"Frequency"=4749419125.0, "S Parameters"=[0.885332408719-0.358778687915i, 0.0343338370213+0.107247889546i, 0.034500167699+0.107151069537i, 0.819934661526-0.480671190453i]}, {"Frequency"=4754731562.5, "S Parameters"=[0.882873744747-0.364472819322i, 0.0346755584075+0.106626767638i, 0.0348541027507+0.106529674959i, 0.81641875337-0.486198538836i]}, {"Frequency"=4760044000.0, "S Parameters"=[0.880183111272-0.370212331275i, 0.035026553234+0.105994621349i, 0.0352215758966+0.105932996534i, 0.813006401762-0.49170050825i]}, {"Frequency"=4765356437.5, "S Parameters"=[0.877377861619-0.375937839683i, 0.035339210295+0.10543260374i, 0.035580397888+0.105378236171i, 0.809510037324-0.497215753126i]}, {"Frequency"=4770668875.0, "S Parameters"=[0.874433275364-0.381809144402i, 0.0356976934519+0.104875174732i, 0.0359646493446+0.104842471927i, 0.805981228134-0.502566823277i]}, {"Frequency"=4775981312.5, "S Parameters"=[0.871536735724-0.387909168782i, 0.0360654462972+0.104329301633i, 0.0364039802868+0.104322705633i, 0.802504293909-0.507823122621i]}, {"Frequency"=4781293750.0, "S Parameters"=[0.868664505904-0.394055974406i, 0.0364310389975+0.103785716648i, 0.036796528618+0.10380246776i, 0.79886498823-0.513065156205i]}, {"Frequency"=4786606187.5, "S Parameters"=[0.865838561013-0.400049649088i, 0.0368158310364+0.103280147198i, 0.037209649244+0.103310136101i, 0.795393418017-0.518315263624i]}, {"Frequency"=4791918625.0, "S Parameters"=[0.863053466579-0.405957393568i, 0.0372154000018+0.10278585014i, 0.0376180696976+0.102842400037i, 0.792051147754-0.523346632506i]}, {"Frequency"=4797231062.5, "S Parameters"=[0.860066264272-0.411531365802i, 0.0376016339101+0.102287857449i, 0.0380050505957+0.102335942698i, 0.788628032057-0.528431582273i]}, {"Frequency"=4802543500.0, "S Parameters"=[0.857084901438-0.417261185933i, 0.0379998783936+0.10179883242i, 0.038394293787+0.101842504167i, 0.785110252527-0.533317762979i]}, {"Frequency"=4807855937.5, "S Parameters"=[0.854057457699-0.423141036992i, 0.0384275697372+0.101300402364i, 0.0388069668331+0.101334862883i, 0.781575253971-0.53816598991i]}, {"Frequency"=4813168375.0, "S Parameters"=[0.851198028864-0.429008838956i, 0.0389129382338+0.100761831709i, 0.0392742346806+0.100815349119i, 0.777890068559-0.543341209097i]}, {"Frequency"=4818480812.5, "S Parameters"=[0.848413261467-0.435020429669i, 0.0394254424234+0.100198195153i, 0.0397549623089+0.100240915344i, 0.774294249555-0.548584590449i]}, {"Frequency"=4823793250.0, "S Parameters"=[0.845678130389-0.440701197394i, 0.0399124497752+0.0996155722056i, 0.0402170767081+0.0996442067979i, 0.770873049139-0.553835486974i]}, {"Frequency"=4829105687.5, "S Parameters"=[0.843060214119-0.44651825706i, 0.040435644457+0.0989930346797i, 0.0407131346589+0.0990374709746i, 0.767394611355-0.55901468948i]}, {"Frequency"=4834418125.0, "S Parameters"=[0.840312092999-0.452002567931i, 0.0409179865766+0.0983568833593i, 0.0411693935749+0.0983777410816i, 0.76406706436-0.564104462184i]}, {"Frequency"=4839730562.5, "S Parameters"=[0.837396996461-0.457427125215i, 0.0413683379196+0.0977044282327i, 0.041630146141+0.097736598021i, 0.760699895823-0.569107956617i]}, {"Frequency"=4845043000.0, "S Parameters"=[0.834454475945-0.462886329825i, 0.0418455886361+0.097044574952i, 0.0420914965511+0.0970802364893i, 0.757350609238-0.573852802963i]}, {"Frequency"=4850355437.5, "S Parameters"=[0.831503515099-0.468181192944i, 0.0422861223013+0.0963848925939i, 0.0425355971825+0.0963972035026i, 0.753896982233-0.578680829739i]}, {"Frequency"=4855667875.0, "S Parameters"=[0.828414480353-0.473674891047i, 0.042693617187+0.0956893322915i, 0.0429657771573+0.0957197310346i, 0.750322517664-0.583391740646i]}, {"Frequency"=4860980312.5, "S Parameters"=[0.825231235062-0.47909573668i, 0.0430765620433+0.0949595302027i, 0.0433846188449+0.0950145125975i, 0.746800278835-0.587930864664i]}, {"Frequency"=4866292750.0, "S Parameters"=[0.82212076351-0.484730801567i, 0.0434265692836+0.0942442614469i, 0.0437480917669+0.0942918108823i, 0.743211214024-0.592606031415i]}, {"Frequency"=4871605187.5, "S Parameters"=[0.819044585227-0.490372448966i, 0.0437849402091+0.093524841585i, 0.0441255651086+0.0935984530213i, 0.739727792677-0.59723270424i]}, {"Frequency"=4876917625.0, "S Parameters"=[0.815943139068-0.495717490545i, 0.0441294673578+0.0928086278193i, 0.0444654782688+0.0928626903591i, 0.736138291752-0.602009260946i]}, {"Frequency"=4882230062.5, "S Parameters"=[0.812821685958-0.501089940855i, 0.044422252049+0.0920926799865i, 0.044736556576+0.0921486567199i, 0.732590226089-0.606747606734i]}, {"Frequency"=4887542500.0, "S Parameters"=[0.809542099784-0.506360804962i, 0.0447162665484+0.0914079173523i, 0.0450100568752+0.0914770708585i, 0.728894479025-0.61115837848i]}, {"Frequency"=4892854937.5, "S Parameters"=[0.805938576906-0.5115304857i, 0.0450118902134+0.0907076461189i, 0.0453013850689+0.0907801889512i, 0.724840458255-0.615600602919i]}, {"Frequency"=4898167375.0, "S Parameters"=[0.802387787169-0.516794810273i, 0.0453317727793+0.0900018873846i, 0.0455832321185+0.0900967413971i, 0.720690606692-0.620083679719i]}, {"Frequency"=4903479812.5, "S Parameters"=[0.799030298559-0.522139862222i, 0.0456505313592+0.089272605334i, 0.0458821989806+0.0893964067307i, 0.716259417754-0.624699870018i]}, {"Frequency"=4908792250.0, "S Parameters"=[0.795724398604-0.527567682205i, 0.0459500166063+0.0885073805001i, 0.0461630830491+0.0886833478222i, 0.712079744776-0.629580123154i]}, {"Frequency"=4914104687.5, "S Parameters"=[0.792408853825-0.532811265018i, 0.0462205934247+0.0877766214147i, 0.0464362487378+0.0879430965782i, 0.707827971035-0.634548381709i]}, {"Frequency"=4919417125.0, "S Parameters"=[0.78923579359-0.53788733426i, 0.046444205886+0.0869958560738i, 0.0466764149603+0.0871788833013i, 0.703655520131-0.639498630312i]}, {"Frequency"=4924729562.5, "S Parameters"=[0.785889563419-0.542869210882i, 0.0466468481905+0.0862453715611i, 0.0468819593306+0.0864512449024i, 0.699381073582-0.644339308043i]}, {"Frequency"=4930042000.0, "S Parameters"=[0.782364525558-0.547784353124i, 0.0468403138297+0.0854938735344i, 0.0471099717721+0.0857287650061i, 0.694912128787-0.649083686454i]}, {"Frequency"=4935354437.5, "S Parameters"=[0.778597817252-0.552610890856i, 0.0469965684515+0.084764199992i, 0.0473024656875+0.0849924792654i, 0.690264236334-0.65385704999i]}, {"Frequency"=4940666875.0, "S Parameters"=[0.77465330083-0.557619671036i, 0.0471211896909+0.0840572782708i, 0.0474481384068+0.0842871378078i, 0.685575704411-0.658570290289i]}, {"Frequency"=4945979312.5, "S Parameters"=[0.77063659941-0.562666752983i, 0.0472063415399+0.0834070733879i, 0.0475566702102+0.0836207669137i, 0.680939046268-0.663315112949i]}, {"Frequency"=4951291750.0, "S Parameters"=[0.766449270701-0.567809641582i, 0.0472782666995+0.0827805937714i, 0.0476419934184+0.0829857083441i, 0.67602040803-0.667841100167i]}, {"Frequency"=4956604187.5, "S Parameters"=[0.762247807811-0.573159730536i, 0.0473545652641+0.0821717364093i, 0.047760396812+0.0823564089443i, 0.671316893753-0.672384869483i]}, {"Frequency"=4961916625.0, "S Parameters"=[0.758227333553-0.57860666374i, 0.0474403107246+0.0816026695718i, 0.0478383099143+0.0817566802102i, 0.666671444981-0.677095584326i]}, {"Frequency"=4967229062.5, "S Parameters"=[0.753994518627-0.583902294496i, 0.0475632591332+0.0810687262993i, 0.047923362334+0.0811668845894i, 0.66204008127-0.681709746955i]}, {"Frequency"=4972541500.0, "S Parameters"=[0.74952319809-0.589130082723i, 0.0476955384426+0.0805693751085i, 0.0480356239204+0.0805997449566i, 0.657515845167-0.686006051006i]}, {"Frequency"=4977853937.5, "S Parameters"=[0.744812616062-0.594317756348i, 0.0478981908299+0.0800722425472i, 0.0481862118637+0.0800486422045i, 0.65290423097-0.690072202689i]}, {"Frequency"=4983166375.0, "S Parameters"=[0.739972360601-0.599702850547i, 0.0481573003607+0.0795169215166i, 0.0484128835538+0.0794936243645i, 0.648072201216-0.694082416661i]}, {"Frequency"=4988478812.5, "S Parameters"=[0.735205316283-0.605152169288i, 0.0484377529109+0.0789578303154i, 0.0486543127979+0.0789368940809i, 0.643061491435-0.698236238659i]}, {"Frequency"=4993791250.0, "S Parameters"=[0.730682724736-0.610632733902i, 0.0487301568003+0.0783695895258i, 0.0489068899461+0.0783598344944i, 0.638240335016-0.702543511067i]}, {"Frequency"=4999103687.5, "S Parameters"=[0.726527103459-0.61607672285i, 0.0490280137285+0.0777399768098i, 0.049200471419+0.0777817759514i, 0.63363483499-0.70707929659i]}, {"Frequency"=5004416125.0, "S Parameters"=[0.722709808916-0.621461566447i, 0.0493355463751+0.0770808165443i, 0.0494944351927+0.0771519950366i, 0.628971604733-0.711388167483i]}, {"Frequency"=5009728562.5, "S Parameters"=[0.718902782763-0.62642045158i, 0.0496118853713+0.0763424243543i, 0.0497939672858+0.0764515947623i, 0.624489937212-0.71583075928i]}, {"Frequency"=5015041000.0, "S Parameters"=[0.715093966512-0.631224694311i, 0.0498673759875+0.0755783971418i, 0.0500572221316+0.0756949264247i, 0.619925892233-0.719830842879i]}, {"Frequency"=5020353437.5, "S Parameters"=[0.711314005135-0.635733515793i, 0.0500436000077+0.0747604421323i, 0.0502731035269+0.0749435324815i, 0.615301456062-0.724147698086i]}, {"Frequency"=5025665875.0, "S Parameters"=[0.707295743497-0.640187218984i, 0.0501942761779+0.0739802527894i, 0.0504322622922+0.0742048887075i, 0.610643135178-0.728181899974i]}, {"Frequency"=5030978312.5, "S Parameters"=[0.703281708739-0.644557466459i, 0.0502973154008+0.0731957941279i, 0.0505588654595+0.0734469034191i, 0.605695032556-0.73222566521i]}, {"Frequency"=5036290750.0, "S Parameters"=[0.699311899451-0.648792639995i, 0.0503586627088+0.0724250537098i, 0.0506391043983+0.0726992671586i, 0.600605940432-0.736342033963i]}, {"Frequency"=5041603187.5, "S Parameters"=[0.695319536058-0.653340061064i, 0.050385911735+0.0717093426544i, 0.0506908247688+0.0719834743127i, 0.595623735713-0.740458865771i]}, {"Frequency"=5046915625.0, "S Parameters"=[0.691450610935-0.657633074257i, 0.0503927335091+0.0710072889252i, 0.0506888967118+0.0712813216524i, 0.590617119789-0.74452060289i]}, {"Frequency"=5052228062.5, "S Parameters"=[0.687481460127-0.661878313316i, 0.050375906336+0.070323134079i, 0.0506635132288+0.0705564653657i, 0.585727252159-0.748631012594i]}, {"Frequency"=5057540500.0, "S Parameters"=[0.683312698641-0.665916260354i, 0.0503561558488+0.0696770558934i, 0.050637082435+0.0698596383891i, 0.580944333601-0.752535615627i]}, {"Frequency"=5062852937.5, "S Parameters"=[0.678998497834-0.669855164573i, 0.0503258242012+0.0690004550065i, 0.0505862465952+0.0691458919292i, 0.576194900059-0.756271715519i]}, {"Frequency"=5068165375.0, "S Parameters"=[0.674168299892-0.67403378918i, 0.0502969774942+0.0683859066418i, 0.0505200257465+0.0684632207661i, 0.571234481569-0.759879524442i]}, {"Frequency"=5073477812.5, "S Parameters"=[0.669120333313-0.678306484579i, 0.0503050177553+0.0677616146113i, 0.0505030074492+0.0678257871252i, 0.566046800139-0.763156949042i]}, {"Frequency"=5078790250.0, "S Parameters"=[0.664025568892-0.682952638553i, 0.0503588213565+0.0671685028277i, 0.0505046406659+0.0672236830918i, 0.560712037762-0.766724972335i]}, {"Frequency"=5084102687.5, "S Parameters"=[0.658975936453-0.687827717577i, 0.0503737378208+0.0665476812083i, 0.0505310361752+0.0666140294595i, 0.555569800238-0.770336145668i]}, {"Frequency"=5089415125.0, "S Parameters"=[0.654159950638-0.692807393525i, 0.0504193601059+0.0659556320728i, 0.0505766069945+0.0660627777557i, 0.550512487568-0.774073690899i]}, {"Frequency"=5094727562.5, "S Parameters"=[0.649402932475-0.697754681939i, 0.0504896037199+0.0653558855108i, 0.0506382728381+0.0654703403963i, 0.54586340491-0.777739577835i]}, {"Frequency"=5100040000.0, "S Parameters"=[0.644706950297-0.702536590337i, 0.0505729925539+0.0647481067562i, 0.0507380429377+0.0648966613257i, 0.54150571927-0.781405199598i]}, {"Frequency"=5105352437.5, "S Parameters"=[0.639867043283-0.706926566266i, 0.0506325187869+0.0640577954815i, 0.0508190023942+0.0642599347903i, 0.537102432603-0.784668139236i]}, {"Frequency"=5110664875.0, "S Parameters"=[0.634895847844-0.711303614765i, 0.050685705744+0.0633849565806i, 0.0508767379065+0.0636161669392i, 0.532524877577-0.787796531086i]}, {"Frequency"=5115977312.5, "S Parameters"=[0.629670609702-0.715642205508i, 0.0507089658294+0.0626841289285i, 0.0509180667744+0.0629413657724i, 0.52772864698-0.790791224903i]}, {"Frequency"=5121289750.0, "S Parameters"=[0.624346169176-0.719832739936i, 0.0506934812717+0.0619649901687i, 0.0509149110646+0.0622497950911i, 0.522569793802-0.793882551849i]}, {"Frequency"=5126602187.5, "S Parameters"=[0.619263480718-0.72423246101i, 0.0506418541585+0.0612831980224i, 0.0508675696862+0.0615846346561i, 0.517360357459-0.79707384212i]}, {"Frequency"=5131914625.0, "S Parameters"=[0.614494869087-0.72862343772i, 0.0505602130604+0.0605973574674i, 0.0508031385617+0.0609101532026i, 0.511989073144-0.800254605336i]}, {"Frequency"=5137227062.5, "S Parameters"=[0.61002540592-0.732892874661i, 0.0504369762175+0.0599286287385i, 0.0506736568616+0.0602600696714i, 0.506629206207-0.803657066294i]}, {"Frequency"=5142539500.0, "S Parameters"=[0.605570256464-0.736875123051i, 0.050310196571+0.0593076935049i, 0.050559275975+0.059622605697i, 0.501419328381-0.807150068587i]}, {"Frequency"=5147851937.5, "S Parameters"=[0.601067955764-0.740675555705i, 0.0502083709749+0.0586977999703i, 0.0504506011905+0.0589743906987i, 0.496143356068-0.81056113457i]}, {"Frequency"=5153164375.0, "S Parameters"=[0.596519132348-0.744050314691i, 0.0500956096428+0.0581184566958i, 0.0502827529418+0.0583520151697i, 0.490818158946-0.813676462401i]}, {"Frequency"=5158476812.5, "S Parameters"=[0.591507465219-0.747536911787i, 0.0499701045812+0.057544964545i, 0.0501545289254+0.0577421937093i, 0.485145301211-0.816457620761i]}, {"Frequency"=5163789250.0, "S Parameters"=[0.586560273503-0.751080124254i, 0.0498947057506+0.0569642270487i, 0.0500381803608+0.0571488201382i, 0.479147907426-0.819423243211i]}, {"Frequency"=5169101687.5, "S Parameters"=[0.581517034679-0.754775552466i, 0.0498292300659+0.0563840765545i, 0.0499577859736+0.0565620650545i, 0.473093925318-0.822573638245i]}, {"Frequency"=5174414125.0, "S Parameters"=[0.576577450569-0.758687752424i, 0.0497630617713+0.0557739355373i, 0.0498594541624+0.0559668763338i, 0.46709875723-0.825796522601i]}, {"Frequency"=5179726562.5, "S Parameters"=[0.571899141334-0.762716272733i, 0.0496933821863+0.0551770471197i, 0.049784606714+0.0553758180992i, 0.46131850354-0.829277696437i]}, {"Frequency"=5185039000.0, "S Parameters"=[0.567433750115-0.766631517566i, 0.0496120101131+0.0545497234453i, 0.0497327053706+0.0547593387001i, 0.4557981196-0.832929567067i]}, {"Frequency"=5190351437.5, "S Parameters"=[0.562615318629-0.770462895462i, 0.0495135275264+0.0539192828197i, 0.0496365432126+0.0541391209869i, 0.450503682615-0.836203222139i]}, {"Frequency"=5195663875.0, "S Parameters"=[0.557821957479-0.773738888926i, 0.0493867156157+0.0533038277346i, 0.0495320559261+0.0535419212179i, 0.445438968165-0.839211802414i]}, {"Frequency"=5200976312.5, "S Parameters"=[0.552519600896-0.777200743124i, 0.049248057647+0.0526886195945i, 0.0493870275645+0.0529386129532i, 0.440222488713-0.841908490361i]}, {"Frequency"=5206288750.0, "S Parameters"=[0.546972494494-0.780592173515i, 0.049086843661+0.0520994727501i, 0.0492333963593+0.0523713010716i, 0.434870761921-0.844519065104i]}, {"Frequency"=5211601187.5, "S Parameters"=[0.541156914369-0.784285102066i, 0.0489385601442+0.0514876637176i, 0.0491029487278+0.0517578009695i, 0.429306355885-0.84711902758i]}, {"Frequency"=5216913625.0, "S Parameters"=[0.535334478315-0.78827688115i, 0.0487059643833+0.0508557820553i, 0.0489244421622+0.0511367586911i, 0.42349147716-0.849615171814i]}, {"Frequency"=5222226062.5, "S Parameters"=[0.529465184839-0.792238099098i, 0.0484946812475+0.0502514479367i, 0.0487071653229+0.050531287884i, 0.417636341889-0.852329545898i]}, {"Frequency"=5227538500.0, "S Parameters"=[0.523903967836-0.79620067943i, 0.0482681832688+0.0496827864327i, 0.0484811997817+0.0499539196653i, 0.411957319867-0.855097297739i]}, {"Frequency"=5232850937.5, "S Parameters"=[0.517981021905-0.800029543011i, 0.0480404322198+0.0491246379118i, 0.0482745775341+0.0493647363977i, 0.406148369712-0.857948466182i]}, {"Frequency"=5238163375.0, "S Parameters"=[0.512331068495-0.803573582504i, 0.0478115716641+0.0485756871312i, 0.0480447570706+0.0487793041226i, 0.400436249785-0.860542737865i]}, {"Frequency"=5243475812.5, "S Parameters"=[0.506193165704-0.806854624024i, 0.0475909192772+0.0480208901151i, 0.0478148061592+0.0481971979206i, 0.394435901757-0.863063722023i]}, {"Frequency"=5248788250.0, "S Parameters"=[0.500117169499-0.810257595564i, 0.0473704370853+0.0474751963281i, 0.0475850736546+0.047624550948i, 0.388151120356-0.865213901902i]}, {"Frequency"=5254100687.5, "S Parameters"=[0.494039101132-0.813672993286i, 0.0471243041211+0.046915287284i, 0.0472823137339+0.0470435763419i, 0.381624165345-0.867444429849i]}, {"Frequency"=5259413125.0, "S Parameters"=[0.488039714865-0.817282371439i, 0.0468397029005+0.0463723265384i, 0.0469745572892+0.0465020122226i, 0.374853167632-0.87001460394i]}, {"Frequency"=5264725562.5, "S Parameters"=[0.482294027941-0.821054976343i, 0.0465572403576+0.0458088299929i, 0.0466570950584+0.0459553215831i, 0.367857443429-0.872754587599i]}, {"Frequency"=5270038000.0, "S Parameters"=[0.476912496258-0.824798374713i, 0.0462754293985+0.0452655158938i, 0.0463501625466+0.0454508106407i, 0.361266157635-0.875894262205i]}, {"Frequency"=5275350437.5, "S Parameters"=[0.471700770644-0.828269930781i, 0.0459421725923+0.0447166408243i, 0.0460089493541+0.0449182840637i, 0.354980553255-0.878995763685i]}, {"Frequency"=5280662875.0, "S Parameters"=[0.466598260142-0.831414882591i, 0.0455891894517+0.0442185583758i, 0.0456568581539+0.0444308751401i, 0.34890552027-0.881818441475i]}, {"Frequency"=5285975312.5, "S Parameters"=[0.461282816788-0.834297493752i, 0.045231293602+0.0437543880289i, 0.0452784762321+0.04400088525i, 0.342912954644-0.88443450223i]}, {"Frequency"=5291287750.0, "S Parameters"=[0.455729970257-0.836808351695i, 0.0448657842996+0.0433188600103i, 0.0449116279187+0.0435856351902i, 0.337028654145-0.886629174077i]}, {"Frequency"=5296600187.5, "S Parameters"=[0.449951756739-0.839473872461i, 0.0444737504523+0.0429132918527i, 0.0445230171183+0.0431868992804i, 0.331170644095-0.888570226311i]}, {"Frequency"=5301912625.0, "S Parameters"=[0.444068730737-0.841949615125i, 0.0441066239385+0.0425331701132i, 0.0441384268042+0.0428069749203i, 0.325137377239-0.890463846045i]}, {"Frequency"=5307225062.5, "S Parameters"=[0.438019934877-0.844836432604i, 0.0437113202825+0.0421706734713i, 0.0437494051259+0.0424437020028i, 0.319004787034-0.892330612377i]}, {"Frequency"=5312537500.0, "S Parameters"=[0.43232986578-0.847717554174i, 0.0433367287903+0.0418225739887i, 0.0433649783505+0.0421014359896i, 0.313021106946-0.894066771402i]}, {"Frequency"=5317849937.5, "S Parameters"=[0.426641043131-0.850407877506i, 0.0429457324116+0.0414534975586i, 0.0429869781742+0.0417214872425i, 0.307187966664-0.895981314886i]}, {"Frequency"=5323162375.0, "S Parameters"=[0.42089375403-0.853089563179i, 0.0425236549173+0.041148113526i, 0.0425879374899+0.0413861333783i, 0.301722708729-0.897742606253i]}, {"Frequency"=5328474812.5, "S Parameters"=[0.414886124146-0.855376115947i, 0.0421068010368+0.0408917909851i, 0.0421740973832+0.04111618166i, 0.296413866688-0.899249120461i]}, {"Frequency"=5333787250.0, "S Parameters"=[0.408743855222-0.857714391015i, 0.0417118948037+0.0407063842902i, 0.0418036173621+0.0409142422774i, 0.29070723434-0.900564252556i]}, {"Frequency"=5339099687.5, "S Parameters"=[0.402507293628-0.859977023893i, 0.0413777972767+0.0405588209396i, 0.0414579164262+0.0407337623364i, 0.284938545307-0.90148182303i]}, {"Frequency"=5344412125.0, "S Parameters"=[0.395973525902-0.862286270083i, 0.0410719841998+0.0404306197001i, 0.0411357260576+0.0405838595676i, 0.278889962913-0.902520058812i]}, {"Frequency"=5349724562.5, "S Parameters"=[0.3896294628-0.865133694897i, 0.0407974607404+0.0403284328605i, 0.0408616657173+0.0404780496324i, 0.27278232339-0.903769394233i]}, {"Frequency"=5355037000.0, "S Parameters"=[0.383676494478-0.867915436603i, 0.0405965544962+0.0402137029483i, 0.0406329699092+0.0403634447345i, 0.266630209554-0.905347453399i]}, {"Frequency"=5360349437.5, "S Parameters"=[0.377750548045-0.87085164419i, 0.0404136851383+0.0400604605162i, 0.0404487176695+0.0402162668919i, 0.260606134835-0.907209888903i]}, {"Frequency"=5365661875.0, "S Parameters"=[0.372166828542-0.873433512827i, 0.0402840555975+0.0399105336363i, 0.0402890514485+0.0400976048721i, 0.254889164022-0.909237555308i]}, {"Frequency"=5370974312.5, "S Parameters"=[0.366632842899-0.875651814671i, 0.0401772308696+0.0397091761611i, 0.0401633934911+0.0399316474233i, 0.249252552974-0.911117085136i]}, {"Frequency"=5376286750.0, "S Parameters"=[0.360805942836-0.877513787536i, 0.0400418179141+0.0394884868072i, 0.0400084255904+0.0397404426916i, 0.243750056854-0.912738843524i]}, {"Frequency"=5381599187.5, "S Parameters"=[0.354875134208-0.879135867223i, 0.039946635303+0.0392732805241i, 0.0399162968048+0.0395500436722i, 0.238144101934-0.913889532141i]}, {"Frequency"=5386911625.0, "S Parameters"=[0.348676264858-0.880912063154i, 0.0398078257764+0.0389772406226i, 0.039765614068+0.0392533500233i, 0.23247514564-0.915060521064i]}, {"Frequency"=5392224062.5, "S Parameters"=[0.342484857134-0.882834586486i, 0.0396387255871+0.0386918269818i, 0.0395729987632+0.0389862081296i, 0.226551632335-0.916179535289i]}, {"Frequency"=5397536500.0, "S Parameters"=[0.336413432163-0.8849433031i, 0.0394371395243+0.0384345656388i, 0.0393782341193+0.0387252147361i, 0.220699701037-0.917338373706i]}, {"Frequency"=5402848937.5, "S Parameters"=[0.330525407525-0.886977209512i, 0.0392142520197+0.0381909468251i, 0.0391532188906+0.0384979764921i, 0.214731614854-0.918718091553i]}, {"Frequency"=5408161375.0, "S Parameters"=[0.324599533425-0.888925827768i, 0.0390099689092+0.0379877317284i, 0.038946905758+0.0382969308566i, 0.209088973125-0.920079870917i]}, {"Frequency"=5413473812.5, "S Parameters"=[0.318691682929-0.890659261118i, 0.0388239549673+0.037819449583i, 0.0387886964833+0.0381185998963i, 0.203595368689-0.921273966445i]}, {"Frequency"=5418786250.0, "S Parameters"=[0.312605625428-0.892441740536i, 0.0386785061078+0.0376379228462i, 0.0386750804994+0.0379218708845i, 0.197975979728-0.922324629456i]}, {"Frequency"=5424098687.5, "S Parameters"=[0.306418826692-0.894149525608i, 0.038528662146+0.0374906003535i, 0.0385549599486+0.0377583782277i, 0.192353001985-0.923014745179i]}, {"Frequency"=5429411125.0, "S Parameters"=[0.300005288766-0.895758783709i, 0.0384293806372+0.0373536491369i, 0.0384747828934+0.0376075824862i, 0.186415943186-0.923561893353i]}, {"Frequency"=5434723562.5, "S Parameters"=[0.293520692586-0.897532123091i, 0.0383769840127+0.0372215855426i, 0.0384255648719+0.0374380933975i, 0.180384758547-0.924208227748i]}, {"Frequency"=5440036000.0, "S Parameters"=[0.287194171463-0.899547780289i, 0.0383603711867+0.037084889525i, 0.0384170460348+0.037273140802i, 0.174280200645-0.924818516592i]}, {"Frequency"=5445348437.5, "S Parameters"=[0.281013579301-0.901647786355i, 0.0384326397694+0.0368877107677i, 0.0384841204431+0.0370615469487i, 0.168124211651-0.925665251591i]}, {"Frequency"=5450660875.0, "S Parameters"=[0.275474083429-0.903764681746i, 0.0384870509398+0.0366158499318i, 0.0385368020479+0.0368158723496i, 0.162036661575-0.926924575288i]}, {"Frequency"=5455973312.5, "S Parameters"=[0.270130305674-0.905707457096i, 0.0385521810904+0.0363303552079i, 0.0385701967427+0.0365513190206i, 0.156333152785-0.928278881551i]}, {"Frequency"=5461285750.0, "S Parameters"=[0.264879011794-0.907449205239i, 0.0386307243613+0.0360146679048i, 0.0386349353135+0.036247760814i, 0.150817727712-0.929450684544i]}, {"Frequency"=5466598187.5, "S Parameters"=[0.259459863878-0.908981389685i, 0.038748708699+0.0356557985028i, 0.0387109827506+0.0359128056249i, 0.145391285508-0.930446760926i]}, {"Frequency"=5471910625.0, "S Parameters"=[0.253762440145-0.910481026763i, 0.0388547464031+0.0352107488963i, 0.0387844389431+0.035471281788i, 0.139797901822-0.931276302755i]}, {"Frequency"=5477223062.5, "S Parameters"=[0.247957478612-0.912001546839i, 0.0389201220006+0.0347289181784i, 0.0388473759199+0.0349910367677i, 0.133923636459-0.932029278231i]}, {"Frequency"=5482535500.0, "S Parameters"=[0.241996988648-0.913742845114i, 0.0389583288947+0.0341691345712i, 0.0388638590402+0.0344311507146i, 0.127721571366-0.932812594271i]}, {"Frequency"=5487847937.5, "S Parameters"=[0.236192566196-0.9155564091i, 0.0389588696977+0.0335690032277i, 0.0388334063193+0.0338531675718i, 0.12125185727-0.93376981169i]}, {"Frequency"=5493160375.0, "S Parameters"=[0.230303722618-0.917465956234i, 0.0389156523731+0.0329342154594i, 0.0387819545292+0.0332184880485i, 0.11507535739-0.935036176015i]}, {"Frequency"=5498472812.5, "S Parameters"=[0.224451896183-0.919284211861i, 0.0388210870784+0.0322375837877i, 0.0386856270854+0.0325204400931i, 0.108959746798-0.936317901894i]}, {"Frequency"=5503785250.0, "S Parameters"=[0.218503893881-0.920893224982i, 0.0385991068302+0.0314927047656i, 0.0384873392456+0.0317916985269i, 0.10265288978-0.937422910615i]}, {"Frequency"=5509097687.5, "S Parameters"=[0.212203497411-0.922483825105i, 0.0383244037538+0.0307983148513i, 0.0382260975705+0.0310822457449i, 0.0964913403477-0.938354455548i]}, {"Frequency"=5514410125.0, "S Parameters"=[0.205646637233-0.924022615449i, 0.037956330433+0.0300870496409i, 0.0378855404776+0.0303624457696i, 0.0899644604457-0.939061783171i]}, {"Frequency"=5519722562.5, "S Parameters"=[0.198875703519-0.925303914475i, 0.0375000845684+0.0294484694844i, 0.0374492908001+0.0297065030357i, 0.0834811505861-0.939479406953i]}, {"Frequency"=5525035000.0, "S Parameters"=[0.19185207375-0.926909205124i, 0.0370375736522+0.0288621895999i, 0.0370052252775+0.0291008157942i, 0.0767013557651-0.940072600398i]}, {"Frequency"=5530347437.5, "S Parameters"=[0.184634758088-0.928691918858i, 0.0365307539684+0.0282958118739i, 0.0365105509702+0.0285307124823i, 0.0697651609-0.9407039597i]}, {"Frequency"=5535659875.0, "S Parameters"=[0.177656386525-0.930541911113i, 0.0360073906847+0.0277818353297i, 0.0359960800283+0.0280013792233i, 0.0628596707105-0.941622703135i]}, {"Frequency"=5540972312.5, "S Parameters"=[0.170903904279-0.932376290049i, 0.0354657117566+0.0273007471718i, 0.0354449773732+0.0275116609692i, 0.0561745846102-0.942618982495i]}, {"Frequency"=5546284750.0, "S Parameters"=[0.164293923345-0.934049883392i, 0.0348884718286+0.0268542624185i, 0.034864012746+0.027073869885i, 0.0497560616319-0.943673760375i]}, {"Frequency"=5551597187.5, "S Parameters"=[0.15777441658-0.935265481768i, 0.0342904153208+0.0264768440158i, 0.0342550115395+0.0266838639815i, 0.0435888264516-0.944523283346i]}, {"Frequency"=5556909625.0, "S Parameters"=[0.151084358645-0.936292100699i, 0.0336928349629+0.026127292909i, 0.0336422288753+0.026321911289i, 0.0373933551651-0.94503597087i]}, {"Frequency"=5562222062.5, "S Parameters"=[0.144229369111-0.93733199332i, 0.0330953754916+0.0258005441749i, 0.033018014797+0.0260047791514i, 0.0311137179726-0.945120298306i]}, {"Frequency"=5567534500.0, "S Parameters"=[0.137248420326-0.938318861174i, 0.032461496109+0.0255050899265i, 0.0323789075386+0.0256983190816i, 0.024743156588-0.944971460101i]}, {"Frequency"=5572846937.5, "S Parameters"=[0.13037923831-0.939350611899i, 0.031846079049+0.0252442340058i, 0.0317536052162+0.0254341123332i, 0.0180623543965-0.944656412926i]}, {"Frequency"=5578159375.0, "S Parameters"=[0.12383074501-0.940445140613i, 0.0312326674571+0.0249976839348i, 0.0311080656347+0.0251915838798i, 0.011375200984-0.944563166165i]}, {"Frequency"=5583471812.5, "S Parameters"=[0.117461591956-0.941275410692i, 0.0305905568997+0.0247967151462i, 0.0304521858929+0.0249875060542i, 0.00473303847101-0.944504264586i]}, {"Frequency"=5588784250.0, "S Parameters"=[0.111229296784-0.941995436839i, 0.029947246954+0.0246570660409i, 0.0297908479339+0.0248470277138i, -0.0014929217706-0.944411049075i]}, {"Frequency"=5594096687.5, "S Parameters"=[0.105102250824-0.942520219171i, 0.0293152075383+0.0245977355099i, 0.0291568318683+0.024793681042i, -0.00760308106734-0.94438215011i]}, {"Frequency"=5599409125.0, "S Parameters"=[0.0988959196006-0.942812306038i, 0.0287157199539+0.0245614159004i, 0.0285480212826+0.0247588742838i, -0.013820031604-0.943958993078i]}, {"Frequency"=5604721562.5, "S Parameters"=[0.0928916345809-0.943016391405i, 0.0281416992474+0.0245965934194i, 0.0279873371159+0.0248030906454i, -0.0198872963016-0.943421127451i]}, {"Frequency"=5610034000.0, "S Parameters"=[0.0867623230527-0.943093373627i, 0.0276371055937+0.0246476366464i, 0.0274866067068+0.0248539727074i, -0.0261795937665-0.942761218917i]}, {"Frequency"=5615346437.5, "S Parameters"=[0.0803205771365-0.943346485781i, 0.0272011320081+0.024680680853i, 0.0270531486231+0.0248998768489i, -0.0326742801621-0.942286994852i]}, {"Frequency"=5620658875.0, "S Parameters"=[0.0738433778301-0.94346684989i, 0.0268055738137+0.0247240339316i, 0.0266619546381+0.0249444686257i, -0.0392971021204-0.941901445892i]}, {"Frequency"=5625971312.5, "S Parameters"=[0.0675345178262-0.944068754226i, 0.0264676266294+0.0247442630022i, 0.0263321176721+0.0249630250973i, -0.0457812743247-0.941671395267i]}, {"Frequency"=5631283750.0, "S Parameters"=[0.0613550943956-0.944452221068i, 0.0261527837177+0.0247129183129i, 0.0260124691964+0.0249429868563i, -0.0519791957229-0.941753576333i]}, {"Frequency"=5636596187.5, "S Parameters"=[0.0550729158098-0.94455772675i, 0.0258354408621+0.0246499307136i, 0.0256956833063+0.0248704428175i, -0.0580224101696-0.94184613543i]}, {"Frequency"=5641908625.0, "S Parameters"=[0.0487933080243-0.944628277478i, 0.0254959646446+0.0245344384267i, 0.0253748401747+0.0247602814866i, -0.0637046510629-0.941787395794i]}, {"Frequency"=5647221062.5, "S Parameters"=[0.042202990724-0.944521945654i, 0.0251595059275+0.0244071458008i, 0.0250075265295+0.0246138965691i, -0.0692921183138-0.941462407752i]}, {"Frequency"=5652533500.0, "S Parameters"=[0.0352030586792-0.944393669813i, 0.0247616174912+0.0242523330675i, 0.0246169994827+0.0244466143861i, -0.0750884698183-0.94086388224i]}, {"Frequency"=5657845937.5, "S Parameters"=[0.0282267979501-0.94454445149i, 0.0243187523373+0.0240887236073i, 0.0241743872326+0.0242561167619i, -0.0809405344688-0.940051943242i]}, {"Frequency"=5663158375.0, "S Parameters"=[0.0210822552511-0.944609253564i, 0.023829817649+0.0239529779687i, 0.0236616016709+0.0241017908631i, -0.0870218252418-0.939342963259i]}, {"Frequency"=5668470812.5, "S Parameters"=[0.0138666741545-0.944785502386i, 0.0233218386366+0.0238578850525i, 0.0231572303772+0.0240013909614i, -0.0933285765545-0.938683274033i]}, {"Frequency"=5673783250.0, "S Parameters"=[0.00669959172527-0.945019153554i, 0.0228260405146+0.0237753110775i, 0.022651817442+0.0239091094717i, -0.0995926979052-0.938102620363i]}, {"Frequency"=5679095687.5, "S Parameters"=[-0.000413995120628-0.945081537092i, 0.022269229262+0.0237195865883i, 0.0220887661891+0.0238484418795i, -0.105803086467-0.937464024322i]}, {"Frequency"=5684408125.0, "S Parameters"=[-0.00750925237465-0.945032416719i, 0.021720760652+0.0236975946953i, 0.0215305233925+0.0238316147246i, -0.112213130241-0.936679935509i]}, {"Frequency"=5689720562.5, "S Parameters"=[-0.0145395946656-0.944940794547i, 0.0211561461445+0.023711599956i, 0.020974516473+0.0238479037422i, -0.118594229248-0.935628389418i]}, {"Frequency"=5695033000.0, "S Parameters"=[-0.0214730063191-0.944684135639i, 0.0206040639738+0.0237548505929i, 0.0204002373411+0.0239042905795i, -0.125046445346-0.934361203032i]}, {"Frequency"=5700345437.5, "S Parameters"=[-0.0281547964961-0.944277784049i, 0.020012180897+0.0238403833064i, 0.0198070578902+0.0239858686798i, -0.131458790684-0.933036566304i]}, {"Frequency"=5705657875.0, "S Parameters"=[-0.0349326385885-0.943859603519i, 0.0194178945387+0.0239801622726i, 0.0192231047385+0.0241423605884i, -0.138115188476-0.93150883684i]}, {"Frequency"=5710970312.5, "S Parameters"=[-0.0415190073073-0.943501969465i, 0.0188366176717+0.0241877055186i, 0.0186578599963+0.0243454799986i, -0.14477020784-0.929934022497i]}, {"Frequency"=5716282750.0, "S Parameters"=[-0.0479734098436-0.943162573774i, 0.0183187313792+0.0244521459686i, 0.0181255657396+0.0246162479081i, -0.151535824544-0.928808183758i]}, {"Frequency"=5721595187.5, "S Parameters"=[-0.0540891624019-0.942695239581i, 0.0178384280055+0.0247483758718i, 0.017638485331+0.0249005177006i, -0.158031257664-0.927606717291i]}, {"Frequency"=5726907625.0, "S Parameters"=[-0.0600412270729-0.941801832064i, 0.0173842319094+0.0250876630603i, 0.0171859599637+0.0252282216865i, -0.164250673325-0.926485407947i]}, {"Frequency"=5732220062.5, "S Parameters"=[-0.0659810123962-0.940897508154i, 0.016988687943+0.0254895298947i, 0.0167813141399+0.0256194592279i, -0.170181049809-0.925203446275i]}, {"Frequency"=5737532500.0, "S Parameters"=[-0.0719582012181-0.939729801521i, 0.0166954189461+0.0259266586905i, 0.0164938900188+0.0260299994465i, -0.175904091064-0.923762527181i]}, {"Frequency"=5742844937.5, "S Parameters"=[-0.0780582369137-0.938650551272i, 0.0164821788035+0.0263454666624i, 0.0162682764542+0.0264192019764i, -0.1816228397-0.922206893095i]}, {"Frequency"=5748157375.0, "S Parameters"=[-0.084144778898-0.93746190337i, 0.0163600575853+0.0267599849183i, 0.0161419559993+0.0268260526785i, -0.187288173721-0.920397103504i]}, {"Frequency"=5753469812.5, "S Parameters"=[-0.090316967751-0.936487735986i, 0.0163286568485+0.0271296730025i, 0.0161047580096+0.0271853797023i, -0.193007702469-0.918724037019i]}, {"Frequency"=5758782250.0, "S Parameters"=[-0.0964186501012-0.935326120503i, 0.0163745429221+0.0274565321167i, 0.0161506180626+0.0274954983881i, -0.198600906813-0.91706906328i]}, {"Frequency"=5764094687.5, "S Parameters"=[-0.102660797107-0.934306315479i, 0.0165122893494+0.0276715043217i, 0.0162821449886+0.0277162366199i, -0.204088517584-0.915648108961i]}, {"Frequency"=5769407125.0, "S Parameters"=[-0.108931320995-0.933293591933i, 0.0166757622062+0.0277599651989i, 0.0164379417837+0.0278150853829i, -0.209540752447-0.914072300489i]}, {"Frequency"=5774719562.5, "S Parameters"=[-0.115353367485-0.932321256235i, 0.0168411599854+0.0277412132677i, 0.0165936022408+0.0277997726005i, -0.215035168918-0.912626475901i]}, {"Frequency"=5780032000.0, "S Parameters"=[-0.12183977359-0.931327788982i, 0.016986037706+0.027592976008i, 0.0167194873187+0.0276683559987i, -0.220617161901-0.911221560205i]}, {"Frequency"=5785344437.5, "S Parameters"=[-0.128379360556-0.930452465889i, 0.0170223219388+0.027345427639i, 0.0167626028314+0.0274289304422i, -0.22636748296-0.909756929016i]}, {"Frequency"=5790656875.0, "S Parameters"=[-0.134912138886-0.92971211331i, 0.0169770086291+0.0270652125827i, 0.0167146362085+0.0271675158712i, -0.232228203453-0.908150109352i]}, {"Frequency"=5795969312.5, "S Parameters"=[-0.141545005823-0.928934398103i, 0.016861320105+0.0267392103887i, 0.0165955958371+0.0268507577317i, -0.238055112609-0.906522040774i]}, {"Frequency"=5801281750.0, "S Parameters"=[-0.148159396707-0.928327300844i, 0.0166168269608+0.0263964174248i, 0.0163684966243+0.026519256958i, -0.244279219404-0.90504932955i]}, {"Frequency"=5806594187.5, "S Parameters"=[-0.154718787048-0.927774308135i, 0.0162932614296+0.0260914215698i, 0.0160449568543+0.026210492724i, -0.250568942574-0.903682358105i]}, {"Frequency"=5811906625.0, "S Parameters"=[-0.161084653888-0.927111847567i, 0.0159157399945+0.0258024988305i, 0.0156718578237+0.0259153948799i, -0.256805803425-0.902383254643i]}, {"Frequency"=5817219062.5, "S Parameters"=[-0.167490677932-0.926221030586i, 0.0154752485347+0.0255480609244i, 0.0152358689588+0.0256247005246i, -0.263042541608-0.901086048006i]}, {"Frequency"=5822531500.0, "S Parameters"=[-0.173724779842-0.925360416714i, 0.0149697503721+0.0253438384343i, 0.0147491114565+0.0253937432705i, -0.2691401634-0.899544202959i]}, {"Frequency"=5827843937.5, "S Parameters"=[-0.180152865394-0.924381720437i, 0.0144374910353+0.0251781858148i, 0.014221022305+0.0252054082834i, -0.275246742861-0.897910731241i]}, {"Frequency"=5833156375.0, "S Parameters"=[-0.186462599032-0.923220177719i, 0.013898039296+0.0250706926292i, 0.0136877076179+0.0250850555417i, -0.281359121847-0.89603278508i]}, {"Frequency"=5838468812.5, "S Parameters"=[-0.19265255472-0.922188880524i, 0.0133501569491+0.0250033319591i, 0.0131429282841+0.0250015092137i, -0.287475518021-0.89411829402i]}, {"Frequency"=5843781250.0, "S Parameters"=[-0.198820902832-0.921010864625i, 0.0127636802865+0.0249993659231i, 0.0125695992723+0.0249611604901i, -0.293591630146-0.892160416944i]}, {"Frequency"=5849093687.5, "S Parameters"=[-0.205045585361-0.919698518466i, 0.0121890826501+0.0250322889526i, 0.0119957033824+0.0249787072674i, -0.299810406028-0.890345581855i]}, {"Frequency"=5854406125.0, "S Parameters"=[-0.2111399805-0.918274769984i, 0.0116101675247+0.0250976793445i, 0.0114278968706+0.0250344017832i, -0.305781097633-0.888219594069i]}, {"Frequency"=5859718562.5, "S Parameters"=[-0.217488263557-0.916757429566i, 0.0110533669032+0.025183915836i, 0.0108406016041+0.0251264089298i, -0.311809494925-0.886232659466i]}, {"Frequency"=5865031000.0, "S Parameters"=[-0.223996003542-0.915221271421i, 0.010477869088+0.0253287053701i, 0.0102601590327+0.0252550277459i, -0.317919029569-0.883925670474i]}, {"Frequency"=5870343437.5, "S Parameters"=[-0.230470785646-0.913459622801i, 0.00993944444398+0.0254983397189i, 0.00971622120589+0.0254253607644i, -0.32407374299-0.881536375113i]}, {"Frequency"=5875655875.0, "S Parameters"=[-0.237020958285-0.911631358929i, 0.009446976948+0.0257010690748i, 0.00920656278683+0.0256124154669i, -0.33020622173-0.879003967855i]}, {"Frequency"=5880968312.5, "S Parameters"=[-0.243778791777-0.909589341322i, 0.00897910395136+0.0258792534816i, 0.00871658003998+0.0258051618305i, -0.336408434831-0.876338927917i]}, {"Frequency"=5886280750.0, "S Parameters"=[-0.250483439469-0.907641554137i, 0.00849876398554+0.0260720041137i, 0.00822119140498+0.0260057563934i, -0.342654637865-0.873401243424i]}, {"Frequency"=5891593187.5, "S Parameters"=[-0.257086292413-0.905654499465i, 0.00803496924236+0.0262755790258i, 0.00774592138852+0.0262172605558i, -0.34889262408-0.870679867462i]}, {"Frequency"=5896905625.0, "S Parameters"=[-0.263717825584-0.903543049526i, 0.00755127069323+0.0264834989951i, 0.00726162605864+0.026426873422i, -0.355095606957-0.867997728432i]}, {"Frequency"=5902218062.5, "S Parameters"=[-0.270164406946-0.901571798815i, 0.00706024760089+0.0266897107524i, 0.00677575376817+0.0266252873217i, -0.361158903747-0.865365666908i]}, {"Frequency"=5907530500.0, "S Parameters"=[-0.276630475068-0.899571319602i, 0.00653756537417+0.0269538134769i, 0.00628847408744+0.0268766371488i, -0.367116502162-0.862697881935i]}, {"Frequency"=5912842937.5, "S Parameters"=[-0.282974892875-0.897528115981i, 0.00605509190628+0.0272280280682i, 0.00582374309529+0.0271426472359i, -0.372949349373-0.860124490636i]}, {"Frequency"=5918155375.0, "S Parameters"=[-0.289161238302-0.895606359648i, 0.00559466609051+0.0275258048501i, 0.00539033637914+0.0274342879652i, -0.378862776834-0.857461867027i]}, {"Frequency"=5923467812.5, "S Parameters"=[-0.295215631698-0.893616458558i, 0.00517918459831+0.0278451534804i, 0.00496445015067+0.0277382578191i, -0.384590968658-0.854632274026i]}, {"Frequency"=5928780250.0, "S Parameters"=[-0.30108439414-0.891608880576i, 0.00475262632388+0.0281479636719i, 0.00455600762864+0.0280245391697i, -0.390446739091-0.851882989148i]}, {"Frequency"=5934092687.5, "S Parameters"=[-0.306814544982-0.889628058609i, 0.00432694468858+0.0284724553076i, 0.00413736973052+0.0283372393445i, -0.396276822047-0.849230378967i]}, {"Frequency"=5939405125.0, "S Parameters"=[-0.312433810802-0.887591504118i, 0.00391032186455+0.0288065107845i, 0.00372980064598+0.0286680697797i, -0.40187282015-0.846538175725i]}, {"Frequency"=5944717562.5, "S Parameters"=[-0.318085319203-0.885589991789i, 0.00353118279137+0.0291635860036i, 0.00334738151937+0.0290032516671i, -0.407449845105-0.843848207951i]}, {"Frequency"=5950030000.0, "S Parameters"=[-0.323558326927-0.883484854828i, 0.00314478109261+0.0295122871825i, 0.00295350428362+0.0293573396521i, -0.412934123209-0.841036507688i]}, {"Frequency"=5955342437.5, "S Parameters"=[-0.329105680244-0.881281348345i, 0.00277623238177+0.0298575435578i, 0.00258203887816+0.029677730396i, -0.418266733494-0.838171440061i]}, {"Frequency"=5960654875.0, "S Parameters"=[-0.334720974575-0.878900371549i, 0.00240814173233+0.0301953541144i, 0.00221652518493+0.0300154302073i, -0.423759242319-0.83518525265i]}, {"Frequency"=5965967312.5, "S Parameters"=[-0.340397606589-0.876371294549i, 0.00204079000063+0.0305465734973i, 0.00183169914536+0.0303420334556i, -0.429128324489-0.832092354498i]}, {"Frequency"=5971279750.0, "S Parameters"=[-0.346082971904-0.87364586435i, 0.00168110469482+0.0308999595386i, 0.00146000615536+0.0307039484663i, -0.434586569506-0.828785256605i]}, {"Frequency"=5976592187.5, "S Parameters"=[-0.351984209287-0.870881086644i, 0.001302785185+0.0312685251694i, 0.00107339241764+0.0310575526924i, -0.440090416664-0.825431778248i]}, {"Frequency"=5981904625.0, "S Parameters"=[-0.358005388298-0.867830036325i, 0.000939298802059+0.0316561888397i, 0.000709736653+0.0314458973i, -0.44561004015-0.822080564707i]}, {"Frequency"=5987217062.5, "S Parameters"=[-0.364141398172-0.864856389493i, 0.000586168150495+0.0320468200512i, 0.000367462762568+0.0318184590417i, -0.451117310228-0.818633132691i]}, {"Frequency"=5992529500.0, "S Parameters"=[-0.370343210525-0.861635595579i, 0.000227694889369+0.0324274108119i, 2.5704901975e-05+0.0321961106784i, -0.456473624786-0.815230397837i]}, {"Frequency"=5997841937.5, "S Parameters"=[-0.37670956863-0.858751298131i, -0.000127892690167+0.032836995405i, -0.000322205753964+0.0326031923449i, -0.462003754666-0.812005425864i]}, {"Frequency"=6003154375.0, "S Parameters"=[-0.383135725503-0.855781449122i, -0.000487238930196+0.0332432918206i, -0.000664604768203+0.0329889286628i, -0.467477281886-0.808720042257i]}, {"Frequency"=6008466812.5, "S Parameters"=[-0.389421535513-0.852978328141i, -0.000862925082148+0.0336744886119i, -0.00100474323825+0.0334255419525i, -0.472764270057-0.805367790381i]}, {"Frequency"=6013779250.0, "S Parameters"=[-0.395778516585-0.850000267201i, -0.00119556517413+0.0341404043826i, -0.00134006562937+0.0338711984587i, -0.478119141805-0.802117645723i]}, {"Frequency"=6019091687.5, "S Parameters"=[-0.401934372494-0.847117768282i, -0.00154809205984+0.0346197375754i, -0.00167782853998+0.0343419328051i, -0.483429425163-0.798811114927i]}, {"Frequency"=6024404125.0, "S Parameters"=[-0.407947869572-0.844050216124i, -0.00186743629393+0.0351102132211i, -0.00200469075112+0.0348395421341i, -0.488501568279-0.795451014257i]}, {"Frequency"=6029716562.5, "S Parameters"=[-0.413965452925-0.84097613685i, -0.00218771992026+0.0356506121802i, -0.00231534436471+0.0353570113666i, -0.493578395032-0.792241890436i]}, {"Frequency"=6035029000.0, "S Parameters"=[-0.419798721487-0.837942958481i, -0.00246931325723+0.0362119439679i, -0.00260253086329+0.0358919104416i, -0.498585548062-0.788888114085i]}, {"Frequency"=6040341437.5, "S Parameters"=[-0.425403715374-0.834874472175i, -0.00271913714048+0.0367807151469i, -0.00286902970015+0.0364496054778i, -0.503418585141-0.785513959789i]}, {"Frequency"=6045653875.0, "S Parameters"=[-0.431056792811-0.831847820025i, -0.00295040097265+0.0373661922795i, -0.00310382178452+0.0370262219311i, -0.50808933357-0.782081706943i]}, {"Frequency"=6050966312.5, "S Parameters"=[-0.436513293849-0.828723709678i, -0.0031403638203+0.0379655661462i, -0.00330307768042+0.0376289203659i, -0.512707565979-0.778715358903i]}, {"Frequency"=6056278750.0, "S Parameters"=[-0.441875997533-0.825577458339i, -0.00329285041621+0.0385783865453i, -0.00345321348069+0.0382164928532i, -0.5172654743-0.775152294196i]}, {"Frequency"=6061591187.5, "S Parameters"=[-0.447052561921-0.8221638164i, -0.00339867627707+0.039159314611i, -0.00356937455185+0.0387831641603i, -0.521745889246-0.771511194045i]}, {"Frequency"=6066903625.0, "S Parameters"=[-0.452369171206-0.818531745439i, -0.00346884300875+0.039735936955i, -0.00365172664299+0.0393502074428i, -0.526346157365-0.767604920913i]}, {"Frequency"=6072216062.5, "S Parameters"=[-0.457652520815-0.814620916314i, -0.00348580416943+0.0402781559831i, -0.00367007337055+0.0398968272121i, -0.53074478201-0.763737837423i]}, {"Frequency"=6077528500.0, "S Parameters"=[-0.463220834619-0.810700336156i, -0.00349558309538+0.0407916324369i, -0.00365443664419+0.0403890716212i, -0.535346098785-0.759751268i]}, {"Frequency"=6082840937.5, "S Parameters"=[-0.469056611983-0.806845802382i, -0.00350740888569+0.0412488757112i, -0.00364020707483+0.0408397838618i, -0.540063428179-0.755618486907i]}, {"Frequency"=6088153375.0, "S Parameters"=[-0.474945825553-0.803066576427i, -0.00350969050617+0.0416848020987i, -0.00361513763146+0.0412899322974i, -0.544915612645-0.751442801329i]}, {"Frequency"=6093465812.5, "S Parameters"=[-0.480772472173-0.799471982139i, -0.00350605903418+0.0421084233642i, -0.00359116535703+0.0416997569282i, -0.549914193988-0.747384171523i]}, {"Frequency"=6098778250.0, "S Parameters"=[-0.486676554603-0.79590969445i, -0.00352227196169+0.0424887842721i, -0.00357938951186+0.0420998668829i, -0.555004601687-0.74358799277i]}, {"Frequency"=6104090687.5, "S Parameters"=[-0.492329348155-0.792453524823i, -0.00354758250871+0.0428513270597i, -0.00361559761881+0.042470210705i, -0.560047408621-0.739578383764i]}, {"Frequency"=6109403125.0, "S Parameters"=[-0.497967846187-0.788890849013i, -0.00360735188711+0.0432108230826i, -0.00365018125944+0.0428302045998i, -0.565110369752-0.735716679468i]}, {"Frequency"=6114715562.5, "S Parameters"=[-0.503480769488-0.78527265046i, -0.00367882710923+0.0435633759957i, -0.00371253837923+0.0431636650546i, -0.570174149039-0.731820131569i]}, {"Frequency"=6120028000.0, "S Parameters"=[-0.508876670759-0.781692105019i, -0.00376348607004+0.0439120239962i, -0.00379513753582+0.0435105286975i, -0.575213659265-0.727779551234i]}, {"Frequency"=6125340437.5, "S Parameters"=[-0.514358723547-0.778119055588i, -0.0038434312536+0.0442810436656i, -0.00388744529584+0.0438414227472i, -0.580307970417-0.723854222184i]}, {"Frequency"=6130652875.0, "S Parameters"=[-0.519647116603-0.774741141557i, -0.00393808041813+0.0446218402454i, -0.00397890441943+0.0441829907498i, -0.585282606892-0.719868905316i]}, {"Frequency"=6135965312.5, "S Parameters"=[-0.524892863677-0.771371377119i, -0.00406142201419+0.0449902131504i, -0.00412866784113+0.0445321278046i, -0.590303834524-0.715960587949i]}, {"Frequency"=6141277750.0, "S Parameters"=[-0.529962290658-0.768163615676i, -0.00419486162194+0.0453849976162i, -0.00425878295103+0.0448812462261i, -0.595050990893-0.712073220464i]}, {"Frequency"=6146590187.5, "S Parameters"=[-0.534733517509-0.764907659397i, -0.00431514303352+0.0457623183822i, -0.00440376525869+0.0452425968165i, -0.599659125428-0.708143047585i]}, {"Frequency"=6151902625.0, "S Parameters"=[-0.539330589534-0.761601741618i, -0.00448324479203+0.0461379060366i, -0.00458572152765+0.0456004535879i, -0.604192868381-0.704466814166i]}, {"Frequency"=6157215062.5, "S Parameters"=[-0.543872686212-0.757804207317i, -0.00468216068242+0.0465247538961i, -0.00477702540358+0.0459814807178i, -0.608536836632-0.700570882899i]}, {"Frequency"=6162527500.0, "S Parameters"=[-0.548412762362-0.753700308886i, -0.00488507230288+0.0469539202164i, -0.00496351112623+0.0463790144518i, -0.612888857735-0.696494647344i]}, {"Frequency"=6167839937.5, "S Parameters"=[-0.553376697945-0.749536916303i, -0.00508458558705+0.0473809530168i, -0.00514642440086+0.0468135998835i, -0.616998861206-0.692143330189i]}, {"Frequency"=6173152375.0, "S Parameters"=[-0.558616099395-0.745283525212i, -0.00529620846898+0.047816681143i, -0.00532096743827+0.0472786981074i, -0.62128976383-0.687630347116i]}, {"Frequency"=6178464812.5, "S Parameters"=[-0.563999915401-0.741105217907i, -0.00550285898204+0.0483155247311i, -0.00550523596152+0.0477993161374i, -0.625700378538-0.683077630406i]}, {"Frequency"=6183777250.0, "S Parameters"=[-0.569530964407-0.736835343898i, -0.00570894752342+0.0488698654357i, -0.00568195913671+0.0483573842728i, -0.630373857239-0.678628825057i]}, {"Frequency"=6189089687.5, "S Parameters"=[-0.574953639586-0.732565078052i, -0.00586882634424+0.0494559200719i, -0.00584555060683+0.0489663034362i, -0.634964476209-0.67403993093i]}, {"Frequency"=6194402125.0, "S Parameters"=[-0.580389726615-0.728187676584i, -0.00603943999227+0.0500651163533i, -0.00598981603732+0.0495762461941i, -0.639511251319-0.669561395678i]}, {"Frequency"=6199714562.5, "S Parameters"=[-0.585586233164-0.723637547911i, -0.00618795764203+0.0507114129499i, -0.00612555124268+0.0502271550915i, -0.643894710773-0.665098068231i]}, {"Frequency"=6205027000.0, "S Parameters"=[-0.590800091956-0.718980538299i, -0.00629916322464+0.0513784337073i, -0.00621443349177+0.0508957418044i, -0.648143557363-0.660591993912i]}, {"Frequency"=6210339437.5, "S Parameters"=[-0.596144763902-0.714034881788i, -0.00635818417103+0.0520529999424i, -0.00627333935268+0.0515588933974i, -0.65231287-0.655877371723i]}, {"Frequency"=6215651875.0, "S Parameters"=[-0.601404134325-0.70918838861i, -0.0063787341956+0.0527639881609i, -0.00627669443269+0.052266259491i, -0.65637258435-0.651198785328i]}, {"Frequency"=6220964312.5, "S Parameters"=[-0.606562552568-0.70424709663i, -0.00631893172025+0.0534707424448i, -0.00623419956332+0.0529501372002i, -0.660507595263-0.646428596279i]}, {"Frequency"=6226276750.0, "S Parameters"=[-0.611883378733-0.699632481919i, -0.00622944042351+0.054158676287i, -0.00614033497948+0.0536333502832i, -0.664654892852-0.641703190493i]}, {"Frequency"=6231589187.5, "S Parameters"=[-0.616845783095-0.69510465195i, -0.00609708597357+0.0548349243188i, -0.00602906257032+0.0542502481497i, -0.668633498804-0.637078800006i]}, {"Frequency"=6236901625.0, "S Parameters"=[-0.621499593978-0.690721045117i, -0.00595772527476+0.0554769592298i, -0.00588684335685+0.0548401178934i, -0.672796695899-0.632691566653i]}, {"Frequency"=6242214062.5, "S Parameters"=[-0.625834019257-0.686301898811i, -0.00584331007199+0.0560870717696i, -0.00576359496719+0.0554084329179i, -0.676686127052-0.628348399274i]}, {"Frequency"=6247526500.0, "S Parameters"=[-0.62986808775-0.681708752161i, -0.0057144829879+0.0567339537496i, -0.00565852638328+0.0559885178913i, -0.680389908919-0.623938696488i]}, {"Frequency"=6252838937.5, "S Parameters"=[-0.634002292238-0.676984717555i, -0.00555082524252+0.0573584778113i, -0.0054737066997+0.0566059521129i, -0.683826422669-0.619541945285i]}, {"Frequency"=6258151375.0, "S Parameters"=[-0.638352658663-0.672221024176i, -0.00534835042775+0.0579401941814i, -0.00524818488469+0.057194984597i, -0.687140172097-0.614744215628i]}, {"Frequency"=6263463812.5, "S Parameters"=[-0.642805017532-0.667456410348i, -0.00508765896555+0.0585152663006i, -0.00499905124907+0.0577727654463i, -0.690739018954-0.609637563767i]}, {"Frequency"=6268776250.0, "S Parameters"=[-0.647184664601-0.662841419218i, -0.00481340317386+0.0590497325423i, -0.0047245989015+0.0583472731337i, -0.694581951595-0.604558887467i]}, {"Frequency"=6274088687.5, "S Parameters"=[-0.651574417655-0.658363814845i, -0.00452713204901+0.0595700904225i, -0.0044149480688+0.058869081518i, -0.698468578282-0.599512119244i]}, {"Frequency"=6279401125.0, "S Parameters"=[-0.655825658304-0.653938617998i, -0.00423816356678+0.0600478154029i, -0.00412633202196+0.0593824317594i, -0.702401731001-0.594552846625i]}, {"Frequency"=6284713562.5, "S Parameters"=[-0.659901623838-0.649413185753i, -0.00394764415094+0.0604992486567i, -0.00381091076048+0.0598446054371i, -0.706322019157-0.589786647858i]}, {"Frequency"=6290026000.0, "S Parameters"=[-0.663809515539-0.644698238652i, -0.00366286736788+0.0609125440595i, -0.00350215359257+0.0603026934195i, -0.710048538332-0.584904746492i]}, {"Frequency"=6295338437.5, "S Parameters"=[-0.667765349731-0.63994181832i, -0.00333987989279+0.0613088861087i, -0.00317014298676+0.0607124202974i, -0.713677657856-0.579975613587i]}, {"Frequency"=6300650875.0, "S Parameters"=[-0.671735931893-0.635128258236i, -0.00303846697689+0.0616625868062i, -0.00285345279656+0.061070738178i, -0.717055740487-0.574989091489i]}, {"Frequency"=6305963312.5, "S Parameters"=[-0.675728752211-0.630245752752i, -0.00275367120839+0.0619384447679i, -0.00253902305691+0.0613763081154i, -0.720520441405-0.569986584803i]}, {"Frequency"=6311275750.0, "S Parameters"=[-0.6800392553-0.625482734395i, -0.0025159003857+0.0621999894396i, -0.0022878992706+0.0616311750074i, -0.724177263463-0.564921528189i]}, {"Frequency"=6316588187.5, "S Parameters"=[-0.684483361818-0.620804551435i, -0.00232083934106+0.0624013191605i, -0.00210411435515+0.0618201869212i, -0.727891530981-0.560014071459i]}, {"Frequency"=6321900625.0, "S Parameters"=[-0.688900812901-0.616042987379i, -0.00220473979556+0.0626257904727i, -0.00195865204528+0.0619978154846i, -0.731846564074-0.555124264987i]}, {"Frequency"=6327213062.5, "S Parameters"=[-0.693272258602-0.611472064446i, -0.00214744378273+0.0628472059489i, -0.00187461458932+0.0621595814922i, -0.735793099642-0.550367906878i]}, {"Frequency"=6332525500.0, "S Parameters"=[-0.697279765805-0.60676965724i, -0.00214295966893+0.0630825323389i, -0.0018376166543+0.0623593906672i, -0.739577170473-0.545809758375i]}, {"Frequency"=6337837937.5, "S Parameters"=[-0.701297163399-0.601647239142i, -0.00218362344957+0.063318385813i, -0.00185849441123+0.0625455098265i, -0.743223709088-0.541241203709i]}, {"Frequency"=6343150375.0, "S Parameters"=[-0.705580827281-0.596411597174i, -0.00228688956319+0.0636023855342i, -0.00191195588783+0.0627993675597i, -0.746589481388-0.536561406072i]}, {"Frequency"=6348462812.5, "S Parameters"=[-0.710106830624-0.591145198481i, -0.00242643871746+0.0639142664075i, -0.00205426256908+0.0631366100679i, -0.749925179901-0.531455454318i]}, {"Frequency"=6353775250.0, "S Parameters"=[-0.714724719662-0.585963409363i, -0.00256732775025+0.0643425270854i, -0.00221407638063+0.0635737512846i, -0.7535016992-0.526206461744i]}, {"Frequency"=6359087687.5, "S Parameters"=[-0.719403687096-0.581067482978i, -0.00271719471487+0.0648340947535i, -0.00238661025481+0.0640842840264i, -0.757258172396-0.520785558007i]}, {"Frequency"=6364400125.0, "S Parameters"=[-0.723905445158-0.576095790029i, -0.00282111230189+0.0654031563622i, -0.00252779304988+0.0646589319i, -0.761349785284-0.515306621715i]}, {"Frequency"=6369712562.5, "S Parameters"=[-0.7282417011-0.571102951582i, -0.00292912944342+0.0660071907517i, -0.00262748238656+0.0652790746962i, -0.765131888663-0.509979444995i]}, {"Frequency"=6375025000.0, "S Parameters"=[-0.73229861734-0.56625592034i, -0.00301293600061+0.0666380150823i, -0.0026957999159+0.0659432882865i, -0.768797893562-0.504665991024i]}, {"Frequency"=6380337437.5, "S Parameters"=[-0.736083312705-0.561134928926i, -0.00301997363912+0.0672963166468i, -0.00270891279212+0.066636603108i, -0.772202567304-0.499215849372i]}, {"Frequency"=6385649875.0, "S Parameters"=[-0.739751314451-0.555872019967i, -0.00301414103918+0.0680025122615i, -0.00264438734439+0.0673630727592i, -0.775447832738-0.493625956839i]}, {"Frequency"=6390962312.5, "S Parameters"=[-0.743359758695-0.550470728387i, -0.0029403795919+0.068735270945i, -0.00256376200451+0.0681303238496i, -0.778499662038-0.487760508308i]}, {"Frequency"=6396274750.0, "S Parameters"=[-0.746974659616-0.544960569113i, -0.0028604908686+0.0694653700539i, -0.00244021307975+0.0689099077529i, -0.781394936302-0.481833232423i]}, {"Frequency"=6401587187.5, "S Parameters"=[-0.750669327169-0.539616265483i, -0.00273758931244+0.0702294199264i, -0.00229746897187+0.0696561014607i, -0.784543844033-0.475827439104i]}, {"Frequency"=6406899625.0, "S Parameters"=[-0.754344205753-0.534368361339i, -0.00259733198458+0.0709673546816i, -0.00209536205562+0.0703777469184i, -0.787667706191-0.46975423381i]}, {"Frequency"=6412212062.5, "S Parameters"=[-0.758055892302-0.529185778417i, -0.00244023276213+0.0716921367947i, -0.00186741217196+0.0710881649795i, -0.790845191417-0.463669197001i]}, {"Frequency"=6417524500.0, "S Parameters"=[-0.761413119302-0.523801000406i, -0.00222573676665+0.0724247086495i, -0.00160558097704+0.0717753565654i, -0.794304352255-0.457791101625i]}, {"Frequency"=6422836937.5, "S Parameters"=[-0.764611725911-0.518178285621i, -0.00200970399025+0.0731480972606i, -0.00130810200545+0.0724365367948i, -0.797402282591-0.451783879892i]}, {"Frequency"=6428149375.0, "S Parameters"=[-0.767610444002-0.512123401725i, -0.00174651378077+0.0738850021498i, -0.000980423968528+0.0731063620212i, -0.800410283008-0.445721775352i]}, {"Frequency"=6433461812.5, "S Parameters"=[-0.770921162727-0.505771759806i, -0.00141067503536+0.0746423312306i, -0.000630082808287+0.0738523953064i, -0.803201052803-0.439438193522i]}, {"Frequency"=6438774250.0, "S Parameters"=[-0.774527040598-0.499367949893i, -0.00100774535553+0.0753722912606i, -0.000244060484727+0.0745650089539i, -0.806032361953-0.432874039604i]}, {"Frequency"=6444086687.5, "S Parameters"=[-0.778308399547-0.493026695375i, -0.000587430097639+0.076078221125i, 0.00011617676244+0.0752877536555i, -0.808973898084-0.426226833617i]}, {"Frequency"=6449399125.0, "S Parameters"=[-0.782295385239-0.486615407742i, -0.000168365933901+0.076781737534i, 0.000510192579987+0.0759699033459i, -0.812164837221-0.419640849445i]}, {"Frequency"=6454711562.5, "S Parameters"=[-0.786192644855-0.480543048106i, 0.000244206099687+0.077398289824i, 0.000881306526806+0.0766293182202i, -0.815436165558-0.413121871i]}, {"Frequency"=6460024000.0, "S Parameters"=[-0.790184751357-0.474335566347i, 0.00064709021197+0.0780122457792i, 0.00126159381643+0.0772583844123i, -0.818847881015-0.406889246647i]}, {"Frequency"=6465336437.5, "S Parameters"=[-0.793760126496-0.46802581501i, 0.00106968122283+0.0786070460757i, 0.00167419483587+0.0779021394419i, -0.821896899435-0.40085003304i]}, {"Frequency"=6470648875.0, "S Parameters"=[-0.797079977647-0.461581114222i, 0.0014824532281+0.0791939881478i, 0.00207391482379+0.0784961839752i, -0.824825867184-0.394766354383i]}, {"Frequency"=6475961312.5, "S Parameters"=[-0.800497281487-0.454815442664i, 0.00186662092197+0.0798179895349i, 0.00247303429494+0.0791888617623i, -0.827190599709-0.388651295246i]}, {"Frequency"=6481273750.0, "S Parameters"=[-0.803669834134-0.447993701164i, 0.00226524972009+0.0804460226839i, 0.00288154384964+0.0798482814187i, -0.829689165353-0.382461829043i]}, {"Frequency"=6486586187.5, "S Parameters"=[-0.807154668489-0.441127281885i, 0.00266872465997+0.0811376402419i, 0.00333053376206+0.0805740090412i, -0.831907778763-0.37594939223i]}, {"Frequency"=6491898625.0, "S Parameters"=[-0.810508996887-0.434473200459i, 0.00308831064096+0.0818302003428i, 0.00381880980408+0.081252015434i, -0.834193491157-0.369652112384i]}, {"Frequency"=6497211062.5, "S Parameters"=[-0.813902802795-0.428267529594i, 0.00350425280969+0.0825094168939i, 0.00429846681879+0.0819262175008i, -0.836583438701-0.363421308607i]}, {"Frequency"=6502523500.0, "S Parameters"=[-0.817079027931-0.422154108984i, 0.00390379653657+0.0832226018143i, 0.00479720916018+0.0825787331531i, -0.838988729174-0.357466809907i]}, {"Frequency"=6507835937.5, "S Parameters"=[-0.819829879649-0.416406620457i, 0.00437703633628+0.0839325222711i, 0.00535541099387+0.0832296114047i, -0.841438097234-0.351675273031i]}, {"Frequency"=6513148375.0, "S Parameters"=[-0.822280285098-0.41056986171i, 0.00487428599107+0.0846155940956i, 0.00596920824094+0.083871137104i, -0.843452957469-0.346019688896i]}, {"Frequency"=6518460812.5, "S Parameters"=[-0.824629607377-0.404557529257i, 0.00544173749637+0.0853323189625i, 0.00664601950659+0.0845477542762i, -0.845283536444-0.340365445145i]}, {"Frequency"=6523773250.0, "S Parameters"=[-0.826847916556-0.398522084589i, 0.00611409087807+0.0860248647458i, 0.00733177719423+0.0852084546998i, -0.846781065638-0.334439331281i]}, {"Frequency"=6529085687.5, "S Parameters"=[-0.82906504297-0.392612076267i, 0.00685011084173+0.0867117198402i, 0.00801169582098+0.085854916658i, -0.848390881603-0.328308110461i]}, {"Frequency"=6534398125.0, "S Parameters"=[-0.831557242428-0.386808179989i, 0.00759524983198+0.087354187989i, 0.00872181144564+0.0864664379891i, -0.850008363642-0.321978119859i]}, {"Frequency"=6539710562.5, "S Parameters"=[-0.834041528549-0.381394189294i, 0.00835616954398+0.0879704926289i, 0.00942034587191+0.0870846801827i, -0.85197223553-0.315722095711i]}, {"Frequency"=6545023000.0, "S Parameters"=[-0.836300190796-0.376332700801i, 0.00908889071593+0.0885820940436i, 0.0101395710909+0.0876859134475i, -0.854047446172-0.30998866729i]}, {"Frequency"=6550335437.5, "S Parameters"=[-0.838320266462-0.371362932903i, 0.00987937704431+0.0891364229731i, 0.0108797965699+0.0883045538608i, -0.85615065209-0.304350765176i]}, {"Frequency"=6555647875.0, "S Parameters"=[-0.839942535937-0.366540343309i, 0.0106650744987+0.0896683653891i, 0.0116590096582+0.0889114437879i, -0.857980236729-0.299150004583i]}, {"Frequency"=6560960312.5, "S Parameters"=[-0.841480254994-0.361300126446i, 0.0115431780572+0.0902122631066i, 0.0125256553616+0.0895216316879i, -0.859374057354-0.293919728437i]}, {"Frequency"=6566272750.0, "S Parameters"=[-0.842696888794-0.355735985915i, 0.0123934727919+0.0907328222765i, 0.0133709611168+0.0900756411646i, -0.860508631018-0.288857525108i]}, {"Frequency"=6571585187.5, "S Parameters"=[-0.844124381428-0.349890387783i, 0.0133515246983+0.0912503761767i, 0.0143453003009+0.0906340845824i, -0.861357653549-0.283499587807i]}, {"Frequency"=6576897625.0, "S Parameters"=[-0.84571036155-0.343727448955i, 0.0143027878132+0.0916976092158i, 0.0153561334612+0.0911128495129i, -0.862131457523-0.278247904886i]}, {"Frequency"=6582210062.5, "S Parameters"=[-0.847379719166-0.337866194647i, 0.0152463973268+0.0921331567675i, 0.0163222540681+0.0915361937502i, -0.862873184162-0.273028376986i]}, {"Frequency"=6587522500.0, "S Parameters"=[-0.8491988739-0.331970166704i, 0.0162112308434+0.0924864890462i, 0.0173430614755+0.0918800334153i, -0.863886949394-0.267863963514i]}, {"Frequency"=6592834937.5, "S Parameters"=[-0.850882214782-0.325954995976i, 0.0171778719835+0.0928394510687i, 0.0184476777979+0.0921629625344i, -0.864924532074-0.263191448763i]}, {"Frequency"=6598147375.0, "S Parameters"=[-0.852210764777-0.320244751198i, 0.0181992018489+0.093071906057i, 0.0195439194004+0.0923305847483i, -0.865816464347-0.258804410143i]}, {"Frequency"=6603459812.5, "S Parameters"=[-0.853451834415-0.3141939439i, 0.019202274806+0.0932187342391i, 0.0206359963385+0.0924461609057i, -0.866463468534-0.254680597969i]}, {"Frequency"=6608772250.0, "S Parameters"=[-0.854603681911-0.308006615408i, 0.0203049474853+0.0933113494501i, 0.0217394135108+0.0925152813551i, -0.866692696102-0.250386909472i]}, {"Frequency"=6614084687.5, "S Parameters"=[-0.855948456661-0.301643349169i, 0.0214271963537+0.0933000321031i, 0.0228338827127+0.0924501136729i, -0.866979725465-0.245940827211i]}, {"Frequency"=6619397125.0, "S Parameters"=[-0.857656421946-0.295270603575i, 0.0224833896568+0.0931685000796i, 0.0238293848846+0.0922800697929i, -0.867206256118-0.241236083472i]}, {"Frequency"=6624709562.5, "S Parameters"=[-0.859449899157-0.289210023493i, 0.0234320621054+0.092924994917i, 0.0246905102919+0.0920200167658i, -0.867839141808-0.236242033827i]}, {"Frequency"=6630022000.0, "S Parameters"=[-0.861703331466-0.283598068987i, 0.0242658276314+0.0925437989039i, 0.0254683073111+0.091671792811i, -0.868875832327-0.231205744664i]}, {"Frequency"=6635334437.5, "S Parameters"=[-0.864010637419-0.278223953724i, 0.0249374929323+0.0922140576539i, 0.0260848024224+0.091341103964i, -0.870383398398-0.226169588455i]}, {"Frequency"=6640646875.0, "S Parameters"=[-0.866111096542-0.273357187432i, 0.025460564898+0.0918456577377i, 0.0266152987098+0.0910613769954i, -0.872086504226-0.221169478308i]}, {"Frequency"=6645959312.5, "S Parameters"=[-0.868131406628-0.26845648193i, 0.025904116701+0.0915796856638i, 0.0270328586395+0.0908580644627i, -0.87378496515-0.216160651024i]}, {"Frequency"=6651271750.0, "S Parameters"=[-0.869634895862-0.263513995423i, 0.0262195395567+0.0913966892823i, 0.0273688365655+0.0907731453114i, -0.875127554943-0.211203227032i]}, {"Frequency"=6656584187.5, "S Parameters"=[-0.871204682942-0.258288469759i, 0.0265080348772+0.0913085563341i, 0.0276517462024+0.0907844121674i, -0.876264428773-0.205681967077i]}, {"Frequency"=6661896625.0, "S Parameters"=[-0.872813233457-0.252819722291i, 0.0267746664858+0.0913273896724i, 0.0279490152154+0.0908752192243i, -0.877263977742-0.199664958983i]}, {"Frequency"=6667209062.5, "S Parameters"=[-0.874441151653-0.247226252858i, 0.0270439815792+0.091413549631i, 0.0282774181201+0.0910155792696i, -0.878205775154-0.193154056496i]}, {"Frequency"=6672521500.0, "S Parameters"=[-0.876255288728-0.241664746991i, 0.0273438215962+0.0915940926371i, 0.028670588159+0.0912210967612i, -0.879424038364-0.18644039441i]}, {"Frequency"=6677833937.5, "S Parameters"=[-0.878013702969-0.236022821911i, 0.0276697746212+0.0917947065069i, 0.0291600352271+0.0914244292086i, -0.880798848375-0.179587575861i]}, {"Frequency"=6683146375.0, "S Parameters"=[-0.879526482894-0.230479787874i, 0.0280873818375+0.092009392696i, 0.0296781350533+0.0916413364787i, -0.882265423199-0.172865448216i]}, {"Frequency"=6688458812.5, "S Parameters"=[-0.880847790957-0.224990676301i, 0.028539348966+0.0922597916917i, 0.0302676492868+0.0919418768388i, -0.883515180406-0.166421816891i]}, {"Frequency"=6693771250.0, "S Parameters"=[-0.881733193845-0.219082224009i, 0.0291336279786+0.0925384704548i, 0.0309335234522+0.0921507326063i, -0.884618783515-0.160105075101i]}, {"Frequency"=6699083687.5, "S Parameters"=[-0.882633622122-0.212828343002i, 0.0297619589935+0.0927788424823i, 0.0315785835674+0.0923394737477i, -0.885277364348-0.153812195157i]}, {"Frequency"=6704396125.0, "S Parameters"=[-0.883661660756-0.206490551872i, 0.0304361304965+0.0930214093823i, 0.0322222644858+0.0925248772325i, -0.885756775788-0.147440414517i]}, {"Frequency"=6709708562.5, "S Parameters"=[-0.884841919561-0.199851956922i, 0.0311980219+0.0931785159111i, 0.0328769767235+0.092596618578i, -0.886309539749-0.14062848794i]}, {"Frequency"=6715021000.0, "S Parameters"=[-0.886595635298-0.193052294891i, 0.0319388668797+0.0932323689871i, 0.0335533107126+0.092582456609i, -0.887036070063-0.133717944339i]}, {"Frequency"=6720333437.5, "S Parameters"=[-0.888285384768-0.186417117428i, 0.0326508547754+0.0931879820627i, 0.0342013334729+0.0925055518653i, -0.888076635242-0.126944336988i]}, {"Frequency"=6725645875.0, "S Parameters"=[-0.889958450236-0.180075283832i, 0.0333715181747+0.0930781992225i, 0.0348477808813+0.0924102760162i, -0.88949140475-0.120275882729i]}, {"Frequency"=6730958312.5, "S Parameters"=[-0.891584778131-0.173871205548i, 0.0340241410142+0.0928962943711i, 0.0354590667573+0.0922606410279i, -0.890907081338-0.114102973396i]}, {"Frequency"=6736270750.0, "S Parameters"=[-0.89278830187-0.167681764758i, 0.0346120366888+0.092669280796i, 0.0359998037152+0.0921062841164i, -0.892269054613-0.108158069424i]}, {"Frequency"=6741583187.5, "S Parameters"=[-0.893980465311-0.161452537937i, 0.0350969800756+0.092474613382i, 0.0364464416631+0.0919744461819i, -0.893333715188-0.102556022026i]}, {"Frequency"=6746895625.0, "S Parameters"=[-0.895086866558-0.155106995819i, 0.0354411740425+0.092306228115i, 0.0368111622441+0.0918698877002i, -0.894106565092-0.096853985639i]}, {"Frequency"=6752208062.5, "S Parameters"=[-0.896326202928-0.148670661961i, 0.0357021792688+0.0921075748892i, 0.037098107103+0.0917599478263i, -0.894681886484-0.0909690037195i]}, {"Frequency"=6757520500.0, "S Parameters"=[-0.897935911493-0.142261863054i, 0.0358779681203+0.0919663609907i, 0.0373072921601+0.0917153428417i, -0.895323506775-0.0847201238968i]}, {"Frequency"=6762832937.5, "S Parameters"=[-0.899677545542-0.136056479324i, 0.0359631797499+0.0918827807116i, 0.0374716577396+0.0917124517416i, -0.896241805133-0.0782039627176i]}, {"Frequency"=6768145375.0, "S Parameters"=[-0.90146042042-0.130018847343i, 0.0359951453074+0.0918983918836i, 0.0376412910763+0.0917598057887i, -0.897606075267-0.0719369394059i]}, {"Frequency"=6773457812.5, "S Parameters"=[-0.902965117969-0.124034557455i, 0.0360527895944+0.0920121300354i, 0.0378132388692+0.0919510340725i, -0.898851280596-0.0656048851271i]}, {"Frequency"=6778770250.0, "S Parameters"=[-0.904210545788-0.118169292487i, 0.0360737926246+0.092218254722i, 0.0379728038285+0.0922401832563i, -0.899900228932-0.0596269608073i]}, {"Frequency"=6784082687.5, "S Parameters"=[-0.905127804065-0.112244547292i, 0.0362170280209+0.092630033933i, 0.038154654512+0.0926200753556i, -0.900802806755-0.0534485217863i]}, {"Frequency"=6789395125.0, "S Parameters"=[-0.905862175302-0.106049036846i, 0.0363781155545+0.0931245016884i, 0.0383769219155+0.0930702704713i, -0.901126687835-0.0473814495422i]}, {"Frequency"=6794707562.5, "S Parameters"=[-0.906649549163-0.100017061788i, 0.0366601723628+0.0937239610802i, 0.0386290207423+0.0936278761793i, -0.901273761481-0.0411494764387i]}, {"Frequency"=6800020000.0, "S Parameters"=[-0.907383230576-0.0937242993888i, 0.0370177326879+0.0943142457824i, 0.0389710660914+0.0941297636519i, -0.901131597285-0.0347323151471i]}, {"Frequency"=6805332437.5, "S Parameters"=[-0.908426303077-0.0873818347533i, 0.0374759738383+0.0948947734865i, 0.0394254758385+0.0946304362795i, -0.901210459723-0.0281863117432i]}, {"Frequency"=6810644875.0, "S Parameters"=[-0.909382594995-0.0814846444388i, 0.0380753700131+0.0954294102857i, 0.0398932883198+0.0951383765322i, -0.901495349479-0.0213543537947i]}, {"Frequency"=6815957312.5, "S Parameters"=[-0.910130395383-0.0757107647538i, 0.0386987540011+0.0959490741114i, 0.0405234112399+0.0956595148011i, -0.901814695553-0.0150390719428i]}, {"Frequency"=6821269750.0, "S Parameters"=[-0.910538747889-0.0700638103237i, 0.0394916064312+0.096416318837i, 0.0412501981291+0.0961755347125i, -0.902271781936-0.00876892353642i]}, {"Frequency"=6826582187.5, "S Parameters"=[-0.910656561916-0.0643375491678i, 0.0403394497093+0.0968581863598i, 0.0420199559158+0.0966777837716i, -0.902390929483-0.00276664388144i]}, {"Frequency"=6831894625.0, "S Parameters"=[-0.91027877402-0.0585312628006i, 0.0411971992366+0.0971944910673i, 0.0428693237721+0.0970891159258i, -0.902053189107+0.00316017411928i]}, {"Frequency"=6837207062.5, "S Parameters"=[-0.910047468104-0.0522986521166i, 0.0420747926244+0.0974632587802i, 0.0437768449846+0.0974189212903i, -0.901452818947+0.00911666727517i]}, {"Frequency"=6842519500.0, "S Parameters"=[-0.909763370959-0.0461161326469i, 0.0429317002647+0.097653248127i, 0.044642894993+0.0976769275835i, -0.900614289606+0.0152973054565i]}, {"Frequency"=6847831937.5, "S Parameters"=[-0.909916859412-0.0396975586792i, 0.0437633454335+0.0977540914289i, 0.0455675333057+0.0978920311449i, -0.899912027108+0.0217316631229i]}, {"Frequency"=6853144375.0, "S Parameters"=[-0.910056785113-0.0336235886035i, 0.0445411361938+0.0978012138976i, 0.0464238232676+0.0979597213882i, -0.89954686929+0.0280518749035i]}, {"Frequency"=6858456812.5, "S Parameters"=[-0.91024346649-0.02743842078i, 0.0452818707459+0.0977368142207i, 0.0473299315906+0.0979737928808i, -0.899303146394+0.0342805981886i]}, {"Frequency"=6863769250.0, "S Parameters"=[-0.91030730462-0.0212118717469i, 0.0460116102075+0.0975858658955i, 0.0481849405603+0.0979130561189i, -0.899266931552+0.0402580391357i]}, {"Frequency"=6869081687.5, "S Parameters"=[-0.910269440375-0.0148297604484i, 0.0466301554566+0.09743503884i, 0.0489384282471+0.0977930734722i, -0.899263073577+0.0459775056537i]}, {"Frequency"=6874394125.0, "S Parameters"=[-0.909920935679-0.00836315437312i, 0.0472083634749+0.0973258716847i, 0.049529305727+0.097662633579i, -0.899088571979+0.0517487776226i]}, {"Frequency"=6879706562.5, "S Parameters"=[-0.909830021768-0.00141154715741i, 0.0476704137424+0.0973027093345i, 0.0500262194011+0.0975707829382i, -0.898843065718+0.0574724910341i]}, {"Frequency"=6885019000.0, "S Parameters"=[-0.909680761048+0.00583301386298i, 0.0480835697393+0.0973148064358i, 0.0504195960368+0.0974794940915i, -0.898342180098+0.0634063022026i]}, {"Frequency"=6890331437.5, "S Parameters"=[-0.910005180279+0.0130557364752i, 0.0485042157438+0.0974156882751i, 0.0507078281162+0.0975082925397i, -0.898100304345+0.0696748440967i]}, {"Frequency"=6895643875.0, "S Parameters"=[-0.910606599242+0.0202424990018i, 0.0488733824227+0.0975329343562i, 0.0510034165737+0.0976010869827i, -0.898048487444+0.0759145579895i]}, {"Frequency"=6900956312.5, "S Parameters"=[-0.91129047582+0.0271905297288i, 0.0492710173056+0.0977263526896i, 0.0512879638673+0.0977976341761i, -0.898386294351+0.0822553393332i]}, {"Frequency"=6906268750.0, "S Parameters"=[-0.911796487443+0.0340785544905i, 0.0496583320118+0.0979585204335i, 0.0516010794285+0.098079485501i, -0.898732723788+0.0883735944496i]}, {"Frequency"=6911581187.5, "S Parameters"=[-0.9119729299+0.0406597185627i, 0.0500611075708+0.09821713801i, 0.0519160938082+0.0984175803799i, -0.899260000196+0.0941810034197i]}, {"Frequency"=6916893625.0, "S Parameters"=[-0.911753302314+0.0473187414048i, 0.0504912438125+0.0985220375749i, 0.0523146205429+0.0987986930065i, -0.899266144082+0.0998414909136i]}, {"Frequency"=6922206062.5, "S Parameters"=[-0.911494941144+0.0540989656716i, 0.0509464447727+0.0988534938685i, 0.0527293224476+0.0992333901522i, -0.898886528435+0.105503748085i]}, {"Frequency"=6927518500.0, "S Parameters"=[-0.911151749784+0.0610300564525i, 0.0513706029936+0.0991716515365i, 0.0531942896965+0.0996907361232i, -0.898120050363+0.111193464296i]}, {"Frequency"=6932830937.5, "S Parameters"=[-0.910823304279+0.0679093085384i, 0.0518689917812+0.0995567106761i, 0.0537065678865+0.100178714361i, -0.897189908913+0.117435332936i]}, {"Frequency"=6938143375.0, "S Parameters"=[-0.910860008192+0.0746441648612i, 0.0523975768703+0.0999178049052i, 0.0542931365011+0.100697709969i, -0.896165006481+0.123688414682i]}, {"Frequency"=6943455812.5, "S Parameters"=[-0.910807842806+0.0810361792874i, 0.0528858958964+0.100381601014i, 0.0549229884263+0.101210591857i, -0.895449177495+0.129996563981i]}, {"Frequency"=6948768250.0, "S Parameters"=[-0.910561800878+0.0871908599904i, 0.0534800983532+0.100821884265i, 0.0556617865494+0.101769226771i, -0.894812296185+0.136342633112i]}, {"Frequency"=6954080687.5, "S Parameters"=[-0.910133546646+0.0931416546889i, 0.0540721658411+0.101322617815i, 0.0563978280438+0.102290139877i, -0.894253502891+0.142395927538i]}, {"Frequency"=6959393125.0, "S Parameters"=[-0.90949282389+0.099204542631i, 0.0547454366413+0.1018457039i, 0.0572053673551+0.102833109859i, -0.893275577604+0.148430979497i]}, {"Frequency"=6964705562.5, "S Parameters"=[-0.908525784121+0.105172951269i, 0.0555379309014+0.102423130771i, 0.0580099094739+0.103356935969i, -0.89208558162+0.154480435319i]}, {"Frequency"=6970018000.0, "S Parameters"=[-0.907326067132+0.111443167707i, 0.056439303243+0.103044917545i, 0.0589086910193+0.103809341689i, -0.890561902524+0.160647308557i]}, {"Frequency"=6975330437.5, "S Parameters"=[-0.906254031831+0.118074659151i, 0.0574247348094+0.103616360585i, 0.0599082225575+0.104261243408i, -0.888854616447+0.166904375746i]}, {"Frequency"=6980642875.0, "S Parameters"=[-0.90516663883+0.124775147596i, 0.0585027098411+0.104084901408i, 0.0609464243501+0.104639261113i, -0.88704608035+0.17326006624i]}, {"Frequency"=6985955312.5, "S Parameters"=[-0.904448530049+0.131269167565i, 0.0596671234073+0.104477592952i, 0.0620212403185+0.104993573094i, -0.885407229783+0.179726764428i]}, {"Frequency"=6991267750.0, "S Parameters"=[-0.90348255636+0.137582962223i, 0.0608972930066+0.104805389275i, 0.0631509977073+0.105278395014i, -0.884214981879+0.186180680312i]}, {"Frequency"=6996580187.5, "S Parameters"=[-0.902375672392+0.143626026964i, 0.0621329748415+0.104943711789i, 0.0642933046699+0.105486614555i, -0.883043074922+0.192238454411i]}, {"Frequency"=7001892625.0, "S Parameters"=[-0.900997320918+0.149359023027i, 0.0632890950585+0.104988453372i, 0.0653572377914+0.105604035527i, -0.881777405506+0.197837998094i]}, {"Frequency"=7007205062.5, "S Parameters"=[-0.89947317041+0.155164163283i, 0.0643983488444+0.104899379094i, 0.0663605032661+0.105619939483i, -0.880300253986+0.203165870018i]}, {"Frequency"=7012517500.0, "S Parameters"=[-0.897681804482+0.16121242373i, 0.0653720708141+0.10470557793i, 0.067302795874+0.105500209881i, -0.878622779393+0.208605094211i]}, {"Frequency"=7017829937.5, "S Parameters"=[-0.896288974598+0.167366728745i, 0.0661870975537+0.104481964838i, 0.0680969665116+0.105390054361i, -0.876917037194+0.214135388821i]}, {"Frequency"=7023142375.0, "S Parameters"=[-0.895229091894+0.173748023696i, 0.0668955009157+0.104249805771i, 0.0688306217715+0.10535081356i, -0.875037786071+0.219980541508i]}, {"Frequency"=7028454812.5, "S Parameters"=[-0.894178215379+0.180047851548i, 0.0675459329442+0.104133674311i, 0.0694810486633+0.105323034969i, -0.873307136187+0.226199942225i]}, {"Frequency"=7033767250.0, "S Parameters"=[-0.893392665191+0.186331416501i, 0.0681014169564+0.104107040963i, 0.0701468438193+0.105423178558i, -0.871865935352+0.232519051539i]}, {"Frequency"=7039079687.5, "S Parameters"=[-0.892587591296+0.192434763699i, 0.0686258419813+0.104225565353i, 0.0707737443093+0.10562991011i, -0.87067866587+0.238846290984i]}, {"Frequency"=7044392125.0, "S Parameters"=[-0.891639098778+0.198465977965i, 0.0692499268802+0.104455564297i, 0.0714311041015+0.105905776467i, -0.869272288664+0.245203608343i]}, {"Frequency"=7049704562.5, "S Parameters"=[-0.890573527761+0.204489245426i, 0.0698589740038+0.104761864694i, 0.0721065172686+0.106292673307i, -0.867747279908+0.251384468502i]}, {"Frequency"=7055017000.0, "S Parameters"=[-0.889116359814+0.210405278385i, 0.0704849532809+0.105159434343i, 0.072857474419+0.106607856134i, -0.865960408244+0.257585289567i]}, {"Frequency"=7060329437.5, "S Parameters"=[-0.887470536721+0.216475843568i, 0.071231839814+0.105569347232i, 0.0736496914751+0.106920743178i, -0.863895258162+0.26384419255i]}, {"Frequency"=7065641875.0, "S Parameters"=[-0.886002701129+0.222792056452i, 0.0720956403419+0.106004421727i, 0.0745546307014+0.10726681178i, -0.861539232279+0.270192480537i]}, {"Frequency"=7070954312.5, "S Parameters"=[-0.884579292239+0.229193999109i, 0.0730832252191+0.106415566978i, 0.0754768731844+0.107576115161i, -0.859267365487+0.276895529492i]}, {"Frequency"=7076266750.0, "S Parameters"=[-0.883186141764+0.235694077166i, 0.074113528354+0.106815892105i, 0.0764865385066+0.107902119552i, -0.857211506914+0.283572206829i]}, {"Frequency"=7081579187.5, "S Parameters"=[-0.881692697842+0.241915669156i, 0.0752020179064+0.107177025592i, 0.0775269291295+0.108263388311i, -0.8553905396+0.290231571441i]}, {"Frequency"=7086891625.0, "S Parameters"=[-0.880127778217+0.248091772298i, 0.0763250702538+0.107515916609i, 0.0785858310404+0.108578283457i, -0.853608425372+0.296616200927i]}, {"Frequency"=7092204062.5, "S Parameters"=[-0.87812568117+0.254321865027i, 0.0774390176779+0.107735005002i, 0.0796924415391+0.108877741138i, -0.851650594491+0.30254230411i]}, {"Frequency"=7097516500.0, "S Parameters"=[-0.876012476082+0.260522872498i, 0.0785642324134+0.10794731055i, 0.0807416512095+0.109160815277i, -0.849593418485+0.308312583511i]}, {"Frequency"=7102828937.5, "S Parameters"=[-0.873722036931+0.266840251237i, 0.0796487488214+0.108104619037i, 0.0818276137455+0.109460321868i, -0.847259030448+0.31395239093i]}, {"Frequency"=7108141375.0, "S Parameters"=[-0.871556645102+0.27329671421i, 0.0807678972627+0.108236946039i, 0.0828736253584+0.109702711397i, -0.844581059357+0.319736578236i]}, {"Frequency"=7113453812.5, "S Parameters"=[-0.869353119741+0.279863893418i, 0.0819355762152+0.108315638339i, 0.0840407298581+0.109890415124i, -0.841841448968+0.325650403105i]}, {"Frequency"=7118766250.0, "S Parameters"=[-0.867259259452+0.286415822281i, 0.0830963638091+0.108379108896i, 0.085234396177+0.110057960928i, -0.839116896689+0.331656787527i]}, {"Frequency"=7124078687.5, "S Parameters"=[-0.865221404883+0.292722466647i, 0.0842543858056+0.108397601237i, 0.0863807617548+0.110245341386i, -0.836464424863+0.337744381021i]}, {"Frequency"=7129391125.0, "S Parameters"=[-0.863242259201+0.298948782506i, 0.0854246720487+0.108406167749i, 0.0875940007358+0.110412151444i, -0.833910729135+0.343786872425i]}, {"Frequency"=7134703562.5, "S Parameters"=[-0.861041787362+0.304829117606i, 0.0866023186964+0.108473135577i, 0.0887671854795+0.110512476277i, -0.831175881061+0.349706523829i]}, {"Frequency"=7140016000.0, "S Parameters"=[-0.858882058807+0.310627848081i, 0.0877079250038+0.108546059798i, 0.0899554379168+0.110597854656i, -0.828434230972+0.355482101027i]}, {"Frequency"=7145328437.5, "S Parameters"=[-0.85665183806+0.316180214743i, 0.0888568031048+0.108629729882i, 0.0911282337224+0.110716184982i, -0.825392608395+0.36127738166i]}, {"Frequency"=7150640875.0, "S Parameters"=[-0.854391292046+0.321708344243i, 0.0900352670389+0.108758594701i, 0.0922946934382+0.110824090652i, -0.822254254507+0.367220468797i]}, {"Frequency"=7155953312.5, "S Parameters"=[-0.852053607386+0.32727632969i, 0.0912272093942+0.108908564353i, 0.0935229274754+0.110876846476i, -0.819006660394+0.373035320957i]}, {"Frequency"=7161265750.0, "S Parameters"=[-0.849792702183+0.332787762542i, 0.0925634388796+0.109021908358i, 0.094799514976+0.110877371989i, -0.815669225741+0.379204282334i]}, {"Frequency"=7166578187.5, "S Parameters"=[-0.847580867682+0.338377965847i, 0.0938593523469+0.109071141291i, 0.0960762844218+0.11089262812i, -0.812517525717+0.385344382998i]}, {"Frequency"=7171890625.0, "S Parameters"=[-0.845259388946+0.343859788758i, 0.0952684494411+0.109085196424i, 0.097426821228+0.110872234662i, -0.809385238505+0.391566094117i]}, {"Frequency"=7177203062.5, "S Parameters"=[-0.84255500152+0.349269363981i, 0.0966568738647+0.109039427638i, 0.0987354171291+0.110775040224i, -0.80643375207+0.397495678308i]}, {"Frequency"=7182515500.0, "S Parameters"=[-0.839753728474+0.354807085462i, 0.0980984250013+0.108933792029i, 0.100090026624+0.110702439311i, -0.803369804272+0.40322145693i]}, {"Frequency"=7187827937.5, "S Parameters"=[-0.836764749566+0.360516596238i, 0.09948247327+0.108774656385i, 0.101471695819+0.110569681873i, -0.800148033779+0.408748987013i]}, {"Frequency"=7193140375.0, "S Parameters"=[-0.833504941388+0.366361868045i, 0.100904305921+0.108558222231i, 0.102820506975+0.110392982665i, -0.796937351705+0.41424146872i]}, {"Frequency"=7198452812.5, "S Parameters"=[-0.830419433612+0.372379826205i, 0.102277390641+0.108274997189i, 0.104213193035+0.110226403863i, -0.793486544492+0.41971597659i]}, {"Frequency"=7203765250.0, "S Parameters"=[-0.827185664228+0.378372639275i, 0.103641757445+0.107983064745i, 0.105551719561+0.110014995855i, -0.79011190876+0.425261530681i]}, {"Frequency"=7209077687.5, "S Parameters"=[-0.824136231461+0.384537614983i, 0.104976424824+0.107601909129i, 0.106929808722+0.10979689083i, -0.786718595619+0.430602686102i]}, {"Frequency"=7214390125.0, "S Parameters"=[-0.820995111868+0.390507503832i, 0.106355441556+0.107172630566i, 0.108262793862+0.10951989478i, -0.783410172993+0.436056509973i]}, {"Frequency"=7219702562.5, "S Parameters"=[-0.817936365419+0.396410072659i, 0.107662196631+0.106703228248i, 0.109660491554+0.10921856318i, -0.780092722763+0.44128728013i]}, {"Frequency"=7225015000.0, "S Parameters"=[-0.814904297625+0.402180157126i, 0.108960994706+0.106246959617i, 0.11098196079+0.108851354757i, -0.776754240611+0.446566121904i]}, {"Frequency"=7230327437.5, "S Parameters"=[-0.811805792292+0.407685042819i, 0.110210747651+0.105762760872i, 0.112341617801+0.108466330843i, -0.773249977682+0.451710895502i]}, {"Frequency"=7235639875.0, "S Parameters"=[-0.808928491554+0.413041915692i, 0.111475087303+0.105273586614i, 0.113667215496+0.108013821684i, -0.769678109665+0.456862800524i]}, {"Frequency"=7240952312.5, "S Parameters"=[-0.805968242292+0.418213422351i, 0.112701203252+0.104752808276i, 0.114954808621+0.10746727791i, -0.76605331301+0.461891704837i]}, {"Frequency"=7246264750.0, "S Parameters"=[-0.803215844232+0.423215120238i, 0.113898230676+0.104241739824i, 0.116201726301+0.106872352304i, -0.762236277184+0.466959235228i]}, {"Frequency"=7251577187.5, "S Parameters"=[-0.800622126869+0.42787576775i, 0.115058795016+0.103733107038i, 0.117339510125+0.106332869627i, -0.758616889349+0.472043136188i]}, {"Frequency"=7256889625.0, "S Parameters"=[-0.79804701203+0.432422525301i, 0.116175348798+0.103217605779i, 0.118431646581+0.105676009544i, -0.755066369091+0.47713903636i]}, {"Frequency"=7262202062.5, "S Parameters"=[-0.795461133435+0.436700963974i, 0.117215080701+0.102615504748i, 0.11942126836+0.105018515873i, -0.751731130451+0.482225145953i]}, {"Frequency"=7267514500.0, "S Parameters"=[-0.792804538518+0.440979670873i, 0.118235500033+0.101999577173i, 0.120362889012+0.104322247603i, -0.748378342521+0.487218526685i]}, {"Frequency"=7272826937.5, "S Parameters"=[-0.789987028294+0.445411436739i, 0.1191769925+0.101367188854i, 0.1212017424+0.103627318839i, -0.74508277719+0.492244181221i]}, {"Frequency"=7278139375.0, "S Parameters"=[-0.78720940871+0.449993105108i, 0.12007211407+0.100810203946i, 0.122051146978+0.103057326826i, -0.741778468089+0.497244701934i]}, {"Frequency"=7283451812.5, "S Parameters"=[-0.784200472913+0.454795495342i, 0.120980188867+0.100298200446i, 0.122852252785+0.102545342882i, -0.738377824712+0.502429243833i]}, {"Frequency"=7288764250.0, "S Parameters"=[-0.781165212227+0.45990908834i, 0.121835939443+0.0998602904496i, 0.123650491481+0.102168118288i, -0.73513902367+0.507523042765i]}, {"Frequency"=7294076687.5, "S Parameters"=[-0.778062115507+0.46513691531i, 0.122752176569+0.0994414647498i, 0.124482440379+0.101843729218i, -0.731756921493+0.512803536137i]}, {"Frequency"=7299389125.0, "S Parameters"=[-0.774751573968+0.470670256543i, 0.123660559511+0.0991304433947i, 0.125338031109+0.101616210963i, -0.728563882409+0.518026118398i]}, {"Frequency"=7304701562.5, "S Parameters"=[-0.771345167673+0.476456612612i, 0.124558742401+0.0988398986718i, 0.126273348021+0.101480967795i, -0.725348328088+0.523307547874i]}, {"Frequency"=7310014000.0, "S Parameters"=[-0.767687579517+0.482361904434i, 0.12557663628+0.098554676665i, 0.12726568859+0.101386698275i, -0.721969186146+0.528393492346i]}, {"Frequency"=7315326437.5, "S Parameters"=[-0.76405105697+0.488261582019i, 0.126594544592+0.098272587884i, 0.128299050574+0.101249070361i, -0.718353663372+0.533454475843i]}, {"Frequency"=7320638875.0, "S Parameters"=[-0.760288543634+0.494306191706i, 0.127661249472+0.0979802286186i, 0.129439415218+0.101111502374i, -0.714707892114+0.53850421582i]}, {"Frequency"=7325951312.5, "S Parameters"=[-0.756432080316+0.500321456435i, 0.128789730674+0.0977122483096i, 0.130661645993+0.100989720405i, -0.710918979701+0.543491202524i]}, {"Frequency"=7331263750.0, "S Parameters"=[-0.752546237531+0.506065871769i, 0.13000322132+0.0974620017281i, 0.131893321493+0.100801963759i, -0.706973408954+0.54836091447i]}, {"Frequency"=7336576187.5, "S Parameters"=[-0.748717605995+0.51171636438i, 0.131207654161+0.0972289626234i, 0.133192324125+0.100597185521i, -0.70290216571+0.553086524116i]}, {"Frequency"=7341888625.0, "S Parameters"=[-0.745113035778+0.517169106806i, 0.132459883295+0.0970505434555i, 0.134540482986+0.100328734876i, -0.698861666277+0.557841141149i]}, {"Frequency"=7347201062.5, "S Parameters"=[-0.741412831981+0.522276607044i, 0.133819448108+0.0967739866643i, 0.135878137621+0.0999856498083i, -0.6945992901+0.562368098493i]}, {"Frequency"=7352513500.0, "S Parameters"=[-0.737797150445+0.527213053405i, 0.135173258276+0.0964835908147i, 0.137265829353+0.0995269683657i, -0.69048380088+0.566656868425i]}, {"Frequency"=7357825937.5, "S Parameters"=[-0.73412894605+0.531888631865i, 0.136672726197+0.0960190919513i, 0.138619536676+0.0989831925519i, -0.686145877271+0.571105853702i]}, {"Frequency"=7363138375.0, "S Parameters"=[-0.730491864958+0.536492721106i, 0.138152639507+0.0954675776354i, 0.140043911547+0.0983382854813i, -0.681828830632+0.575331786144i]}, {"Frequency"=7368450812.5, "S Parameters"=[-0.726726669611+0.540797401157i, 0.139672441052+0.0947734925467i, 0.141444432949+0.0975782828621i, -0.677397414393+0.579517679864i]}, {"Frequency"=7373763250.0, "S Parameters"=[-0.722934153001+0.544954864622i, 0.141207134924+0.0940181714448i, 0.142791696621+0.0967872972253i, -0.672977619149+0.583761694552i]}, {"Frequency"=7379075687.5, "S Parameters"=[-0.719096486186+0.549034341467i, 0.14271233038+0.0931635828539i, 0.144186531598+0.0959142201161i, -0.668558255552+0.587928441813i]}, {"Frequency"=7384388125.0, "S Parameters"=[-0.715152389155+0.553011229928i, 0.144222836771+0.0922349976296i, 0.145566808541+0.0950072481133i, -0.6641069685+0.592066229408i]}, {"Frequency"=7389700562.5, "S Parameters"=[-0.711036874543+0.556994029715i, 0.145614230808+0.0912674050734i, 0.1468859402+0.0940894438598i, -0.659734811632+0.596161158776i]}, {"Frequency"=7395013000.0, "S Parameters"=[-0.706897873361+0.561032242191i, 0.146983101947+0.0902413578418i, 0.148192164516+0.0931168243908i, -0.655398814469+0.600191549948i]}, {"Frequency"=7400325437.5, "S Parameters"=[-0.702688914471+0.565019610091i, 0.148288350741+0.0891193491312i, 0.149434268413+0.0921542082537i, -0.651022742655+0.604183462317i]}, {"Frequency"=7405637875.0, "S Parameters"=[-0.698375464091+0.569162493214i, 0.149505232286+0.08790753002i, 0.150663917286+0.0911253696247i, -0.646684884684+0.608138152276i]}, {"Frequency"=7410950312.5, "S Parameters"=[-0.693976246213+0.573373423529i, 0.150695822338+0.0866523836473i, 0.151838548309+0.0900971465343i, -0.642332913102+0.612115723099i]}, {"Frequency"=7416262750.0, "S Parameters"=[-0.689603806902+0.57774253662i, 0.151707443846+0.0854013571101i, 0.15296324516+0.0890179628469i, -0.637968959913+0.615997578489i]}, {"Frequency"=7421575187.5, "S Parameters"=[-0.685266661455+0.582047864727i, 0.152651946699+0.0841177086954i, 0.154015086502+0.0878635078056i, -0.63371708684+0.619946082518i]}, {"Frequency"=7426887625.0, "S Parameters"=[-0.680978894276+0.586312467108i, 0.153533166107+0.0828494363303i, 0.155034533449+0.0867241826932i, -0.629419920759+0.623823888062i]}, {"Frequency"=7432200062.5, "S Parameters"=[-0.676693517731+0.590594702802i, 0.154315886769+0.0816428134598i, 0.155913930265+0.0855471493522i, -0.625206793257+0.627592339236i]}, {"Frequency"=7437512500.0, "S Parameters"=[-0.672513320016+0.594824646045i, 0.155044562434+0.0804727074977i, 0.156728730812+0.0842719618452i, -0.620993923221+0.631216069351i]}, {"Frequency"=7442824937.5, "S Parameters"=[-0.668481710063+0.599123492267i, 0.155722492712+0.0792685835707i, 0.157438810738+0.0830031875693i, -0.616850277281+0.634765864015i]}, {"Frequency"=7448137375.0, "S Parameters"=[-0.664621332604+0.603340779412i, 0.156297508254+0.0781341188478i, 0.157996238794+0.0817779052597i, -0.612776155645+0.638451333801i]}, {"Frequency"=7453449812.5, "S Parameters"=[-0.661173140981+0.607561614193i, 0.156893735519+0.0770138918575i, 0.15849665632+0.0805616019548i, -0.608759730868+0.642153151992i]}, {"Frequency"=7458762250.0, "S Parameters"=[-0.65775878831+0.611676190464i, 0.157496352765+0.0759338573676i, 0.158917936032+0.0793528636489i, -0.604737747213+0.646061342934i]}, {"Frequency"=7464074687.5, "S Parameters"=[-0.654434593031+0.615591122778i, 0.157948440849+0.0748836842857i, 0.159239436568+0.0783097769394i, -0.600828556755+0.649859815771i]}, {"Frequency"=7469387125.0, "S Parameters"=[-0.651219490795+0.619533221989i, 0.158508597615+0.0738580159512i, 0.159578020922+0.0772068685216i, -0.596883806911+0.653674450097i]}, {"Frequency"=7474699562.5, "S Parameters"=[-0.647846108721+0.623329095886i, 0.159015488579+0.0728708937941i, 0.159899640136+0.0761633219868i, -0.592961033572+0.657503217814i]}, {"Frequency"=7480012000.0, "S Parameters"=[-0.644447645309+0.627061288708i, 0.159469670655+0.0719473882841i, 0.160260440206+0.0752580982259i, -0.589037717138+0.661196850844i]}, {"Frequency"=7485324437.5, "S Parameters"=[-0.640931481814+0.630952639424i, 0.159925861601+0.0709585415271i, 0.160575908971+0.0743589708009i, -0.585072630982+0.66495945282i]}, {"Frequency"=7490636875.0, "S Parameters"=[-0.637305962622+0.634905110732i, 0.160280614174+0.0700478417837i, 0.160863878215+0.0735255605475i, -0.581022322772+0.668651994701i]}, {"Frequency"=7495949312.5, "S Parameters"=[-0.633658772261+0.638897101836i, 0.160593192103+0.0691863228739i, 0.161137016935+0.0728188392284i, -0.577073799648+0.672556067431i]}, {"Frequency"=7501261750.0, "S Parameters"=[-0.629969071364+0.643106626104i, 0.160852770229+0.0684424238156i, 0.16139289729+0.0722202468333i, -0.57315204111+0.676412046481i]}, {"Frequency"=7506574187.5, "S Parameters"=[-0.626186758404+0.647368842626i, 0.161052922526+0.0678103621363i, 0.161613903299+0.0717852099266i, -0.569252129555+0.680402691973i]}, {"Frequency"=7511886625.0, "S Parameters"=[-0.622191692645+0.651705361723i, 0.16121940181+0.0673232912448i, 0.161867995597+0.0713925993159i, -0.56513665008+0.684455086603i]}, {"Frequency"=7517199062.5, "S Parameters"=[-0.618045095239+0.656150892908i, 0.16144838185+0.0669470638792i, 0.162246671921+0.071072121414i, -0.561166678116+0.688582590056i]}, {"Frequency"=7522511500.0, "S Parameters"=[-0.613530234729+0.660692397509i, 0.161721036619+0.0666458853203i, 0.162642950542+0.0707398605247i, -0.55690580916+0.692628006847i]}, {"Frequency"=7527823937.5, "S Parameters"=[-0.608796936029+0.665539774538i, 0.162069204619+0.0663770240969i, 0.163126691084+0.0704438448722i, -0.552423184262+0.696535005219i]}, {"Frequency"=7533136375.0, "S Parameters"=[-0.604113034582+0.670616668566i, 0.162604191975+0.0661130091236i, 0.163686906764+0.0701275083518i, -0.547718676662+0.700500062066i]}, {"Frequency"=7538448812.5, "S Parameters"=[-0.599529655685+0.675832692031i, 0.163187327854+0.0659218705151i, 0.164333743817+0.0698290553017i, -0.542827538759+0.704637076674i]}, {"Frequency"=7543761250.0, "S Parameters"=[-0.595070913866+0.680855384567i, 0.163884622087+0.0656734351046i, 0.164947734108+0.0695137854529i, -0.537879635276+0.708841014333i]}, {"Frequency"=7549073687.5, "S Parameters"=[-0.590826006767+0.685836919202i, 0.16470050779+0.0654729610465i, 0.165621965137+0.0692377628681i, -0.533094176949+0.713090704268i]}, {"Frequency"=7554386125.0, "S Parameters"=[-0.586647577019+0.690384624397i, 0.165526809952+0.0652200665011i, 0.166276242895+0.0689286814104i, -0.528297903741+0.717243071913i]}, {"Frequency"=7559698562.5, "S Parameters"=[-0.582518320304+0.694881130957i, 0.166470404864+0.0648884158619i, 0.167012449103+0.0685536106517i, -0.523296275803+0.721380399527i]}, {"Frequency"=7565011000.0, "S Parameters"=[-0.57822225232+0.699044250647i, 0.167412328081+0.0645244217626i, 0.167754645868+0.0681414096578i, -0.518238673528+0.725317794824i]}, {"Frequency"=7570323437.5, "S Parameters"=[-0.57413644422+0.703162619297i, 0.16838410822+0.0641413061303i, 0.168614845621+0.0677795210578i, -0.513034024832+0.729148589458i]}, {"Frequency"=7575635875.0, "S Parameters"=[-0.569926020159+0.70717078387i, 0.169392996935+0.0636427910283i, 0.169536834864+0.0673433925479i, -0.507632661218+0.732961586534i]}, {"Frequency"=7580948312.5, "S Parameters"=[-0.565693772202+0.710968040868i, 0.17043102307+0.0631424966085i, 0.170457181566+0.0669721320115i, -0.502099311588+0.736910785894i]}, {"Frequency"=7586260750.0, "S Parameters"=[-0.561508296089+0.714763725872i, 0.171483163109+0.0626283255104i, 0.171475287845+0.0665883081825i, -0.496548109668+0.740734501487i]}, {"Frequency"=7591573187.5, "S Parameters"=[-0.55726654607+0.718408438776i, 0.172560027174+0.0620670600321i, 0.172488681347+0.0661878782054i, -0.490997918432+0.744628666184i]}, {"Frequency"=7596885625.0, "S Parameters"=[-0.553054270857+0.72200712534i, 0.173622126619+0.0615902776934i, 0.17359322142+0.065771134183i, -0.485535698183+0.748451344692i]}, {"Frequency"=7602198062.5, "S Parameters"=[-0.548626884934+0.72523746284i, 0.174611048511+0.0610014787816i, 0.174665009485+0.0653141111461i, -0.480044720696+0.752142050441i]}, {"Frequency"=7607510500.0, "S Parameters"=[-0.543857823462+0.72842298451i, 0.175631676266+0.0604450243775i, 0.17583816501+0.0647612523746i, -0.474646053229+0.755533878066i]}, {"Frequency"=7612822937.5, "S Parameters"=[-0.538573451613+0.731618366441i, 0.176653832716+0.0598266180672i, 0.177054457726+0.0640821010447i, -0.469168503031+0.758808745933i]}, {"Frequency"=7618135375.0, "S Parameters"=[-0.532990965236+0.735065521526i, 0.177775254003+0.0591217455699i, 0.178260998231+0.0632787334764i, -0.463407361228+0.761976820075i]}, {"Frequency"=7623447812.5, "S Parameters"=[-0.527104312811+0.738747622804i, 0.178897094554+0.0583583660831i, 0.179488962969+0.0623978878067i, -0.457506407688+0.765116158674i]}, {"Frequency"=7628760250.0, "S Parameters"=[-0.52140541173+0.742557742957i, 0.180003491559+0.0575232717793i, 0.180636206023+0.0614610060724i, -0.451636562846+0.768174507773i]}, {"Frequency"=7634072687.5, "S Parameters"=[-0.515664627504+0.746553525832i, 0.181164634695+0.0566660858739i, 0.181732714506+0.0604492206138i, -0.445850668839+0.771406356361i]}, {"Frequency"=7639385125.0, "S Parameters"=[-0.510001213454+0.75038695844i, 0.182310337115+0.0557253798704i, 0.182737906017+0.0594421484066i, -0.44026393196+0.774740330514i]}, {"Frequency"=7644697562.5, "S Parameters"=[-0.504517050801+0.754024759482i, 0.183376087323+0.0547828424662i, 0.183661890021+0.058407461532i, -0.43480698881+0.777815536798i]}, {"Frequency"=7650010000.0, "S Parameters"=[-0.499002002899+0.757497922767i, 0.184405287612+0.0538105020869i, 0.184511783582+0.0573779557367i, -0.429567038854+0.780816740234i]}, {"Frequency"=7655322437.5, "S Parameters"=[-0.4935824012+0.760940601948i, 0.18541871624+0.0527919341388i, 0.185325057781+0.056367268565i, -0.424463257228+0.78360751324i]}, {"Frequency"=7660634875.0, "S Parameters"=[-0.488084952527+0.764407035486i, 0.186356883427+0.0517741314801i, 0.186115199232+0.0553631641577i, -0.419172893608+0.786183515947i]}, {"Frequency"=7665947312.5, "S Parameters"=[-0.482812029481+0.7678321451i, 0.187322352729+0.0507098859159i, 0.186893255358+0.0544481810452i, -0.413773770845+0.788766549643i]}, {"Frequency"=7671259750.0, "S Parameters"=[-0.47768743827+0.771366874505i, 0.188265863837+0.0496694128318i, 0.187691738494+0.0535656513647i, -0.408287778715+0.791357484418i]}, {"Frequency"=7676572187.5, "S Parameters"=[-0.472768986662+0.774793069162i, 0.189239876612+0.0486509700687i, 0.188480353027+0.0527105556626i, -0.402759762196+0.794070838149i]}, {"Frequency"=7681884625.0, "S Parameters"=[-0.467962794235+0.778032483466i, 0.190121446408+0.0476566656508i, 0.189219626913+0.0518821034143i, -0.397235815803+0.796778233121i]}, {"Frequency"=7687197062.5, "S Parameters"=[-0.463604086345+0.781038257302i, 0.190990274759+0.0466570434206i, 0.190063668177+0.0510623426702i, -0.391767708408+0.799518273073i]}, {"Frequency"=7692509500.0, "S Parameters"=[-0.459073406755+0.783626927153i, 0.191814107903+0.0457409714994i, 0.190899332596+0.0502475618586i, -0.386545282116+0.802160950252i]}, {"Frequency"=7697821937.5, "S Parameters"=[-0.454579597307+0.785941177709i, 0.192618018748+0.0447854347329i, 0.191793524636+0.0494297469195i, -0.381194047273+0.804529886546i]}, {"Frequency"=7703134375.0, "S Parameters"=[-0.449660830033+0.788250694117i, 0.193441306853+0.0438505458524i, 0.192794743246+0.0485641617752i, -0.375791123227+0.806611362624i]}, {"Frequency"=7708446812.5, "S Parameters"=[-0.444567151716+0.790717142379i, 0.194329020427+0.042944328598i, 0.193806407031+0.0475597733546i, -0.370180972353+0.808690170581i]}, {"Frequency"=7713759250.0, "S Parameters"=[-0.439371818686+0.793473187905i, 0.195224646089+0.0419282763311i, 0.194876700341+0.0464940018515i, -0.364194264457+0.81086114657i]}, {"Frequency"=7719071687.5, "S Parameters"=[-0.434035785349+0.796382577793i, 0.196158904582+0.0409655043901i, 0.195865378956+0.0453220191046i, -0.358288582482+0.813222527639i]}, {"Frequency"=7724384125.0, "S Parameters"=[-0.428708821461+0.79935901409i, 0.19716184019+0.0399161777992i, 0.196884829584+0.0441180049966i, -0.352137050087+0.815686227282i]}, {"Frequency"=7729696562.5, "S Parameters"=[-0.423363099884+0.802078839046i, 0.198217368608+0.0388759707341i, 0.197801468359+0.042888562042i, -0.346322224762+0.818241876382i]}, {"Frequency"=7735009000.0, "S Parameters"=[-0.417899336432+0.804821738569i, 0.199247234705+0.0377991447274i, 0.198740637815+0.0416548156116i, -0.340582038318+0.820711782686i]}, {"Frequency"=7740321437.5, "S Parameters"=[-0.412136892031+0.807445422206i, 0.200211183801+0.0366534388959i, 0.199647302322+0.0403851464649i, -0.334998757176+0.82298324623i]}, {"Frequency"=7745633875.0, "S Parameters"=[-0.406029698508+0.809996058895i, 0.201137187572+0.0354692186191i, 0.200452854153+0.0391582625141i, -0.329377391076+0.825051466458i]}, {"Frequency"=7750946312.5, "S Parameters"=[-0.400035019732+0.812664767283i, 0.202050849902+0.0342476193403i, 0.201302749058+0.0380081093086i, -0.32360143168+0.826790501739i]}, {"Frequency"=7756258750.0, "S Parameters"=[-0.39379510093+0.815419380626i, 0.203000988556+0.0330185811204i, 0.202101336334+0.0368228211625i, -0.317751550291+0.828719208802i]}, {"Frequency"=7761571187.5, "S Parameters"=[-0.387666580716+0.818444531677i, 0.203858637325+0.0317424474711i, 0.202844211925+0.0357315955028i, -0.311730291903+0.830536534874i]}, {"Frequency"=7766883625.0, "S Parameters"=[-0.38155443031+0.821505268213i, 0.204703368427+0.0304327849661i, 0.203559700452+0.034595605846i, -0.305680102154+0.832599431161i]}, {"Frequency"=7772196062.5, "S Parameters"=[-0.375784865297+0.824425180373i, 0.205501569066+0.0291865096487i, 0.204217837609+0.0334820230473i, -0.299818863029+0.834703946065i]}, {"Frequency"=7777508500.0, "S Parameters"=[-0.370256397219+0.827225774926i, 0.20623447772+0.0279050849061i, 0.204956226586+0.0323811312428i, -0.293876997768+0.836673442795i]}, {"Frequency"=7782820937.5, "S Parameters"=[-0.364773202278+0.829484493677i, 0.206890127574+0.0266329205099i, 0.205684198353+0.0312121119078i, -0.288176681643+0.838594511846i]}, {"Frequency"=7788133375.0, "S Parameters"=[-0.359298680882+0.831490747162i, 0.207590516236+0.025356748281i, 0.206453366128+0.0300491805327i, -0.282337956418+0.840289992076i]}, {"Frequency"=7793445812.5, "S Parameters"=[-0.353739780352+0.833431756121i, 0.208265866919+0.0241256464499i, 0.207240061493+0.0288297294807i, -0.276406568271+0.84168653272i]}, {"Frequency"=7798758250.0, "S Parameters"=[-0.34847584026+0.835587657184i, 0.208989664334+0.0229253778909i, 0.208082055386+0.0275919536705i, -0.270339490575+0.843076787996i]}, {"Frequency"=7804070687.5, "S Parameters"=[-0.343237569487+0.837839654919i, 0.209707344693+0.0217376680182i, 0.208878450297+0.0262616791647i, -0.264071690622+0.844468786677i]}, {"Frequency"=7809383125.0, "S Parameters"=[-0.338317437191+0.840109672836i, 0.210537894847+0.0204875123762i, 0.209714663105+0.0248964984459i, -0.257502286593+0.845954734375i]}, {"Frequency"=7814695562.5, "S Parameters"=[-0.333555846137+0.8421174247i, 0.211339167309+0.0192217118218i, 0.210496427203+0.0233992176904i, -0.251176206181+0.847696849381i]}, {"Frequency"=7820008000.0, "S Parameters"=[-0.328821435524+0.844080513006i, 0.212201371048+0.0179345112443i, 0.211303238757+0.0218686627833i, -0.244994399564+0.849374508348i]}, {"Frequency"=7825320437.5, "S Parameters"=[-0.324254651986+0.84561964862i, 0.21299150682+0.0165853945735i, 0.212053122176+0.0203231729573i, -0.238786356282+0.850972007029i]}, {"Frequency"=7830632875.0, "S Parameters"=[-0.319187346308+0.8468502331i, 0.213809098376+0.0151449466527i, 0.212781594576+0.0187393176538i, -0.232753527009+0.852363912053i]}, {"Frequency"=7835945312.5, "S Parameters"=[-0.314004314448+0.848097377352i, 0.21456055647+0.0136105974274i, 0.213536698843+0.0171933192116i, -0.226599463722+0.853594359323i]}, {"Frequency"=7841257750.0, "S Parameters"=[-0.308606847658+0.849331376756i, 0.215305391358+0.0121341510157i, 0.214248149506+0.0157029861335i, -0.220459547764+0.854524980244i]}, {"Frequency"=7846570187.5, "S Parameters"=[-0.302873594894+0.850865970089i, 0.215992456978+0.0105771356307i, 0.214880647411+0.0142242928228i, -0.214265567636+0.855495306675i]}, {"Frequency"=7851882625.0, "S Parameters"=[-0.297209967995+0.852461351289i, 0.216644630469+0.00905611587265i, 0.215391459752+0.0127858355458i, -0.20802453068+0.856573262112i]}, {"Frequency"=7857195062.5, "S Parameters"=[-0.291456796019+0.854130851618i, 0.217190586633+0.00753212279697i, 0.215804983996+0.0113264646692i, -0.201815605677+0.85771840045i]}, {"Frequency"=7862507500.0, "S Parameters"=[-0.285543786785+0.85602367488i, 0.217648416087+0.00601875739789i, 0.216229306208+0.00990962186459i, -0.195662480082+0.859041509057i]}, {"Frequency"=7867819937.5, "S Parameters"=[-0.279608427596+0.857733588228i, 0.21804769627+0.00447060013252i, 0.216627354482+0.00847655414883i, -0.189740020624+0.860438969234i]}, {"Frequency"=7873132375.0, "S Parameters"=[-0.273572864399+0.859117046466i, 0.218421248319+0.00299920748833i, 0.216966125504+0.00713216033947i, -0.183777851168+0.861758841691i]}, {"Frequency"=7878444812.5, "S Parameters"=[-0.267251125161+0.860644053187i, 0.218818227565+0.00158789691544i, 0.217326392551+0.00576426797651i, -0.177923100255+0.862934577445i]}, {"Frequency"=7883757250.0, "S Parameters"=[-0.260686668208+0.862283865944i, 0.219198408002+0.000211840951326i, 0.217747629606+0.00442181015961i, -0.171877629931+0.863849165049i]}, {"Frequency"=7889069687.5, "S Parameters"=[-0.254047988526+0.864295520198i, 0.219691933328-0.00112291049298i, 0.218213562561+0.0030556571159i, -0.165639256324+0.864775141348i]}, {"Frequency"=7894382125.0, "S Parameters"=[-0.247554032435+0.866446257649i, 0.220176029158-0.00244258829887i, 0.218664838189+0.00168154567573i, -0.159345095074+0.865702551545i]}, {"Frequency"=7899694562.5, "S Parameters"=[-0.241241731971+0.868580574382i, 0.220728349002-0.00374937777478i, 0.21911271781+0.000248026444413i, -0.152897088074+0.86699208725i]}, {"Frequency"=7905007000.0, "S Parameters"=[-0.23541079145+0.870849082258i, 0.221298737078-0.00509744477039i, 0.219604729291-0.00120578162494i, -0.146587203928+0.86814782424i]}, {"Frequency"=7910319437.5, "S Parameters"=[-0.229790602225+0.872607238771i, 0.221824804509-0.00651186843314i, 0.220088277247-0.00278668656208i, -0.140433843562+0.869471491382i]}, {"Frequency"=7915631875.0, "S Parameters"=[-0.224284599909+0.874195863115i, 0.222384594786-0.00795273504647i, 0.220596054843-0.00435624376095i, -0.134507453372+0.870552049755i]}, {"Frequency"=7920944312.5, "S Parameters"=[-0.218878382297+0.875337425029i, 0.222942890776-0.00944900343318i, 0.221075532463-0.0059072645821i, -0.12867334463+0.871452599464i]}, {"Frequency"=7926256750.0, "S Parameters"=[-0.213244707999+0.876367699306i, 0.223452453181-0.0109761340586i, 0.221596377891-0.0073716905906i, -0.12275995351+0.87193261873i]}, {"Frequency"=7931569187.5, "S Parameters"=[-0.207572262377+0.877475774101i, 0.223969578523-0.0124880209544i, 0.222013681945-0.00885775173094i, -0.116747642389+0.872224320694i]}, {"Frequency"=7936881625.0, "S Parameters"=[-0.201826376827+0.878516225008i, 0.224421261955-0.0139360356793i, 0.222415285729-0.0103395223507i, -0.110730668653+0.872583757152i]}, {"Frequency"=7942194062.5, "S Parameters"=[-0.196266920567+0.879755585094i, 0.224890668431-0.0154178873062i, 0.222741161085-0.011783557357i, -0.104493936108+0.872895510337i]}, {"Frequency"=7947506500.0, "S Parameters"=[-0.190842879167+0.881005394409i, 0.225232097201-0.0168383774708i, 0.223147859807-0.0131699244733i, -0.0984744143333+0.873291969212i]}, {"Frequency"=7952818937.5, "S Parameters"=[-0.185474526299+0.881936094547i, 0.225586823464-0.018263730135i, 0.223448182582-0.0145647067932i, -0.092442788594+0.873926917031i]}, {"Frequency"=7958131375.0, "S Parameters"=[-0.180083451124+0.882781319285i, 0.225973170482-0.0196408254628i, 0.223805969755-0.0159577642271i, -0.0866318342023+0.874470880873i]}, {"Frequency"=7963443812.5, "S Parameters"=[-0.174539037282+0.883436518859i, 0.226318714622-0.0210853759806i, 0.224224926308-0.0173399529788i, -0.0807434059798+0.874782438744i]}, {"Frequency"=7968756250.0, "S Parameters"=[-0.168609909241+0.883920036026i, 0.22674050529-0.0225413784761i, 0.224602120983-0.0187889620709i, -0.0748941800483+0.875083377935i]}, {"Frequency"=7974068687.5, "S Parameters"=[-0.162317924205+0.884473243632i, 0.227150337637-0.023999682304i, 0.225049295986-0.0202840788762i, -0.0687904330092+0.874973420425i]}, {"Frequency"=7979381125.0, "S Parameters"=[-0.155912445985+0.885441514444i, 0.22766089319-0.0254936641613i, 0.225498674766-0.0218351099215i, -0.0623696484166+0.874987064227i]}, {"Frequency"=7984693562.5, "S Parameters"=[-0.149393686704+0.886674938873i, 0.228189648943-0.0270069366272i, 0.225954408391-0.0234848021306i, -0.0559098263111+0.875112944058i]}, {"Frequency"=7990006000.0, "S Parameters"=[-0.143281633342+0.887819400798i, 0.228719962216-0.0285465525622i, 0.226376136811-0.0251503722336i, -0.0493609167534+0.87530135665i]}, {"Frequency"=7995318437.5, "S Parameters"=[-0.137480277533+0.889026302783i, 0.229212456959-0.0301400641717i, 0.226781604022-0.0268369312894i, -0.0431437096755+0.875663041772i]}, {"Frequency"=8000630875.0, "S Parameters"=[-0.131879777031+0.890042361479i, 0.229664336059-0.0317698648761i, 0.227192591468-0.0285415076872i, -0.037138933877+0.876033085834i]}, {"Frequency"=8005943312.5, "S Parameters"=[-0.126332698484+0.890486398993i, 0.230055077963-0.0334734022341i, 0.227538586224-0.0302603407288i, -0.0312932889588+0.876299587234i]}, {"Frequency"=8011255750.0, "S Parameters"=[-0.12055528001+0.891009994336i, 0.230443611536-0.0351642494578i, 0.227899211177-0.0319720270197i, -0.0256321120356+0.876105056333i]}, {"Frequency"=8016568187.5, "S Parameters"=[-0.114891180279+0.891215053567i, 0.230840775002-0.0369438801072i, 0.228109408906-0.0336554221687i, -0.0198383983762+0.875643734201i]}, {"Frequency"=8021880625.0, "S Parameters"=[-0.10904737969+0.891574537309i, 0.231156678965-0.0386619817589i, 0.228350460347-0.0353067299173i, -0.0140005430172+0.875071354036i]}, {"Frequency"=8027193062.5, "S Parameters"=[-0.103240978576+0.891954307627i, 0.231388335883-0.040399751146i, 0.228534068626-0.036958210158i, -0.00805366716683+0.8743784829i]}, {"Frequency"=8032505500.0, "S Parameters"=[-0.0974256787455+0.892511464689i, 0.231590825641-0.042129740107i, 0.228683015763-0.0386757160234i, -0.00198843478851+0.873828110042i]}, {"Frequency"=8037817937.5, "S Parameters"=[-0.0919226087517+0.892908141033i, 0.231718362854-0.0438383908181i, 0.228842417335-0.0404057608133i, 0.00401648692684+0.873390770304i]}, {"Frequency"=8043130375.0, "S Parameters"=[-0.0863929368077+0.893267936069i, 0.231829197439-0.0455681391268i, 0.228975436055-0.0420553151543i, 0.00988283595785+0.873039887273i]}, {"Frequency"=8048442812.5, "S Parameters"=[-0.0811787071223+0.893291493582i, 0.231958746873-0.0472234368143i, 0.229116180709-0.0437102904396i, 0.0157616233823+0.87262008166i]}, {"Frequency"=8053755250.0, "S Parameters"=[-0.0757246317479+0.89311800783i, 0.232037559439-0.0488360233603i, 0.229200648666-0.0453209943294i, 0.0215760891631+0.872150629909i]}, {"Frequency"=8059067687.5, "S Parameters"=[-0.0700964784333+0.89290632593i, 0.232172951323-0.0504601851351i, 0.229382574966-0.0469874677942i, 0.0274320763357+0.8714812778i]}, {"Frequency"=8064380125.0, "S Parameters"=[-0.0640922710922+0.892822648476i, 0.2322642244-0.0520851601719i, 0.229531469312-0.0487047161532i, 0.0335979003678+0.870681106905i]}, {"Frequency"=8069692562.5, "S Parameters"=[-0.0578753011959+0.892998190614i, 0.232391050637-0.0537286383804i, 0.22970719867-0.0504109294376i, 0.0400993673501+0.869783633304i]}, {"Frequency"=8075005000.0, "S Parameters"=[-0.0514560720843+0.8934041687i, 0.232510408018-0.0553780898434i, 0.229832294045-0.0521842442332i, 0.0468700690798+0.869307864255i]}, {"Frequency"=8080317437.5, "S Parameters"=[-0.0451785267813+0.893878792486i, 0.232677937681-0.0570937229704i, 0.229985707833-0.0540243505857i, 0.0536834687765+0.868741648762i]}, {"Frequency"=8085629875.0, "S Parameters"=[-0.0390287103702+0.894582669036i, 0.23280989902-0.058819861341i, 0.230189339303-0.0558433542986i, 0.0604338437284+0.86852117725i]}, {"Frequency"=8090942312.5, "S Parameters"=[-0.0329778583123+0.894846034807i, 0.23293390452-0.0605382814927i, 0.230356900269-0.0575927173116i, 0.0670948075849+0.868180510119i]}, {"Frequency"=8096254750.0, "S Parameters"=[-0.0270419328753+0.894964936724i, 0.233134056888-0.06225637537i, 0.230494373022-0.0593366580405i, 0.0734455354655+0.867809863368i]}, {"Frequency"=8101567187.5, "S Parameters"=[-0.0210447854406+0.894816420498i, 0.233234782724-0.0639517525815i, 0.230571253895-0.0610094622829i, 0.0796462567144+0.867343961732i]}, {"Frequency"=8106879625.0, "S Parameters"=[-0.0148555246835+0.894520810473i, 0.233277546851-0.065661559169i, 0.230532837901-0.0627212945422i, 0.0857717816494+0.866432851925i]}, {"Frequency"=8112192062.5, "S Parameters"=[-0.00861854737604+0.894460925734i, 0.233298502809-0.0673120474619i, 0.230438279943-0.0643920465972i, 0.0920468939646+0.865406076452i]}, {"Frequency"=8117504500.0, "S Parameters"=[-0.00241650301655+0.894442660606i, 0.233302656666-0.0689884986942i, 0.230343237951-0.0661165921176i, 0.0984813235892+0.864384789186i]}, {"Frequency"=8122816937.5, "S Parameters"=[0.00372955157129+0.894555012795i, 0.233241776029-0.0707299469973i, 0.230235785896-0.0678682948241i, 0.104867994272+0.863222839188i]}, {"Frequency"=8128129375.0, "S Parameters"=[0.00955568580329+0.894539181746i, 0.233176316758-0.0724786996985i, 0.230094822144-0.0696092821478i, 0.111392409635+0.862243958515i]}, {"Frequency"=8133441812.5, "S Parameters"=[0.0152799634827+0.894418954321i, 0.233163258815-0.0741278041012i, 0.230004030973-0.0712926578518i, 0.117642995476+0.861377350043i]}, {"Frequency"=8138754250.0, "S Parameters"=[0.0207069818479+0.894085440982i, 0.233194866673-0.0757714816956i, 0.229993329943-0.0729340739089i, 0.123661450008+0.860322942986i]}, {"Frequency"=8144066687.5, "S Parameters"=[0.0260668927369+0.893532040571i, 0.233240558346-0.0773785339125i, 0.229946663397-0.0745961984717i, 0.129679519588+0.859281296302i]}, {"Frequency"=8149379125.0, "S Parameters"=[0.0315957180506+0.89272202758i, 0.233374890954-0.0790977023376i, 0.23004040101-0.0762659136563i, 0.135641372361+0.857924976491i]}, {"Frequency"=8154691562.5, "S Parameters"=[0.037236356867+0.891998305515i, 0.233507056119-0.0807752900372i, 0.230107466371-0.0779978589684i, 0.141486775659+0.856358959282i]}, {"Frequency"=8160004000.0, "S Parameters"=[0.0430265467287+0.891177273622i, 0.233622085163-0.0825441209637i, 0.230258721413-0.0798188317902i, 0.147467757506+0.854622464775i]}, {"Frequency"=8165316437.5, "S Parameters"=[0.0491135937028+0.890750322319i, 0.233719070801-0.0843943854796i, 0.230423784554-0.081776913146i, 0.153806041765+0.852951888704i]}, {"Frequency"=8170628875.0, "S Parameters"=[0.0552910481839+0.89021813398i, 0.233751268811-0.0863223521812i, 0.230565961029-0.0837789826786i, 0.160194364716+0.851432086775i]}, {"Frequency"=8175941312.5, "S Parameters"=[0.0610444140188+0.889641116826i, 0.23384555353-0.0882835797474i, 0.230694679831-0.085809168151i, 0.166493739979+0.850044053042i]}, {"Frequency"=8181253750.0, "S Parameters"=[0.067062909148+0.888853099268i, 0.233778490736-0.0903208930053i, 0.230696568572-0.0878379126515i, 0.17260756363+0.848541377011i]}, {"Frequency"=8186566187.5, "S Parameters"=[0.073080833977+0.887767433567i, 0.233718703285-0.0922758004292i, 0.23064569871-0.0897887972063i, 0.178457679262+0.847179275792i]}, {"Frequency"=8191878625.0, "S Parameters"=[0.0792622559659+0.886671401192i, 0.233581622315-0.0942438839049i, 0.230481446987-0.0918115108587i, 0.184175341406+0.845486464484i]}, {"Frequency"=8197191062.5, "S Parameters"=[0.0856637707251+0.885407603736i, 0.233317685096-0.0962184190081i, 0.230222962314-0.093752545503i, 0.189677324477+0.843578742409i]}, {"Frequency"=8202503500.0, "S Parameters"=[0.0921944948357+0.88420011249i, 0.233005812894-0.0980580220939i, 0.229886049445-0.0957277789016i, 0.195397582869+0.841661286408i]}, {"Frequency"=8207815937.5, "S Parameters"=[0.0986444665616+0.883171859326i, 0.232633772082-0.0999896438987i, 0.229481182883-0.097682443145i, 0.201183261131+0.839476183908i]}, {"Frequency"=8213128375.0, "S Parameters"=[0.105134554383+0.882286564237i, 0.232222442895-0.101905118726i, 0.229014872653-0.0996505681702i, 0.207139587245+0.837315504857i]}, {"Frequency"=8218440812.5, "S Parameters"=[0.111452494377+0.88144527721i, 0.231875328794-0.103728465599i, 0.228551544587-0.101640535895i, 0.213309844112+0.835207947005i]}, {"Frequency"=8223753250.0, "S Parameters"=[0.117358918318+0.880677574259i, 0.231451781623-0.105581521698i, 0.228043941733-0.103589071945i, 0.219377776588+0.833191053428i]}, {"Frequency"=8229065687.5, "S Parameters"=[0.122881498571+0.879755207246i, 0.231126183234-0.107386551729i, 0.227508280907-0.105511502768i, 0.225292900984+0.83127337668i]}, {"Frequency"=8234378125.0, "S Parameters"=[0.128220960464+0.878681918001i, 0.23075828027-0.109225215666i, 0.227078987375-0.1074060308i, 0.231233996995+0.829205877581i]}, {"Frequency"=8239690562.5, "S Parameters"=[0.133367592126+0.877461834053i, 0.230501227071-0.111071201636i, 0.226696316082-0.109217420509i, 0.237072953959+0.827039963073i]}, {"Frequency"=8245003000.0, "S Parameters"=[0.138310502008+0.876244392812i, 0.230217800029-0.112896144205i, 0.226350935005-0.111131888987i, 0.242774405603+0.824464656903i]}, {"Frequency"=8250315437.5, "S Parameters"=[0.14323629693+0.875229095073i, 0.229954461994-0.114796870161i, 0.226133119049-0.113029634514i, 0.248598117423+0.822069518403i]}, {"Frequency"=8255627875.0, "S Parameters"=[0.147913190451+0.874441582422i, 0.229715566134-0.116699836466i, 0.225899430245-0.114996161181i, 0.254517024351+0.819650373708i]}, {"Frequency"=8260940312.5, "S Parameters"=[0.15235022126+0.873446464542i, 0.229457849909-0.11874818827i, 0.225691467409-0.116991131066i, 0.260384047524+0.817180970856i]}, {"Frequency"=8266252750.0, "S Parameters"=[0.156689229+0.872239223083i, 0.229096378724-0.120857043323i, 0.225425122163-0.119029419683i, 0.266144961259+0.815001406659i]}, {"Frequency"=8271565187.5, "S Parameters"=[0.161056576389+0.870779922221i, 0.228758691692-0.122925309372i, 0.225106202758-0.121014219282i, 0.27170799816+0.812748718265i]}, {"Frequency"=8276877625.0, "S Parameters"=[0.165646319756+0.869017524754i, 0.228320315541-0.125022337912i, 0.224687866523-0.123145703734i, 0.277139860703+0.810471451527i]}, {"Frequency"=8282190062.5, "S Parameters"=[0.170520844344+0.866979628037i, 0.227811273921-0.127156606922i, 0.224126755889-0.125216048647i, 0.282120460448+0.8079377686i]}, {"Frequency"=8287502500.0, "S Parameters"=[0.17570944905+0.86471781254i, 0.227205560352-0.129260759523i, 0.223487203672-0.127356893465i, 0.287115209032+0.805249522192i]}, {"Frequency"=8292814937.5, "S Parameters"=[0.181412267497+0.862501414185i, 0.226505059107-0.131422924867i, 0.222799604771-0.129541378235i, 0.292025425041+0.802402351321i]}, {"Frequency"=8298127375.0, "S Parameters"=[0.18737745497+0.860139660603i, 0.225733910862-0.133591581107i, 0.222067956085-0.131774314513i, 0.296923217395+0.799551536247i]}, {"Frequency"=8303439812.5, "S Parameters"=[0.193544250005+0.857999004337i, 0.224992580515-0.135747505854i, 0.221227261928-0.133916934056i, 0.301914873543+0.796478094915i]}, {"Frequency"=8308752250.0, "S Parameters"=[0.19980219537+0.855929177186i, 0.224108460476-0.137857306511i, 0.220297324256-0.136056529193i, 0.306968904036+0.793477302273i]}, {"Frequency"=8314064687.5, "S Parameters"=[0.206228923739+0.853819649533i, 0.223197315653-0.139927698167i, 0.219327448857-0.138205633222i, 0.312118326854+0.790562733913i]}, {"Frequency"=8319377125.0, "S Parameters"=[0.212524093393+0.85160364303i, 0.222182354652-0.141958786192i, 0.218285468541-0.140323068567i, 0.317218423369+0.787635585232i]}, {"Frequency"=8324689562.5, "S Parameters"=[0.218654821624+0.849262514842i, 0.221211231451-0.144042287069i, 0.217246403132-0.142392970324i, 0.322393581519+0.784799144534i]}, {"Frequency"=8330002000.0, "S Parameters"=[0.224782832839+0.846976154584i, 0.220138620813-0.146133906658i, 0.216233870412-0.14444279438i, 0.327329077303+0.78180035137i]}, {"Frequency"=8335314437.5, "S Parameters"=[0.230805972937+0.84472250682i, 0.219069637036-0.148169705366i, 0.215238983995-0.146520617691i, 0.332344679952+0.778611587362i]}, {"Frequency"=8340626875.0, "S Parameters"=[0.236719803338+0.842905275526i, 0.218001444565-0.15020810626i, 0.214296601817-0.148590212962i, 0.337448203593+0.775318932481i]}, {"Frequency"=8345939312.5, "S Parameters"=[0.242113873197+0.841249382967i, 0.216853894836-0.152251420183i, 0.213342182151-0.150637758016i, 0.342732662504+0.772090686707i]}, {"Frequency"=8351251750.0, "S Parameters"=[0.247008485164+0.839802092386i, 0.215687289396-0.154242394555i, 0.212286948981-0.152615447426i, 0.348008088027+0.768998907945i]}, {"Frequency"=8356564187.5, "S Parameters"=[0.251398708016+0.838434619292i, 0.214471828619-0.156176186828i, 0.211170979562-0.15457999969i, 0.353125700838+0.76621665688i]}, {"Frequency"=8361876625.0, "S Parameters"=[0.255445535268+0.8366823661i, 0.213104332698-0.158075329654i, 0.209840634308-0.156516032854i, 0.358147804121+0.763419507213i]}, {"Frequency"=8367189062.5, "S Parameters"=[0.259272725599+0.834880328194i, 0.211676048506-0.159934176445i, 0.208415781925-0.158452758861i, 0.362667840602+0.760736824015i]}, {"Frequency"=8372501500.0, "S Parameters"=[0.262982987366+0.832785384699i, 0.210105852139-0.161747524801i, 0.206887104521-0.160392848207i, 0.366995073579+0.757961195587i]}, {"Frequency"=8377813937.5, "S Parameters"=[0.26682965315+0.830620718633i, 0.208527151032-0.16356898167i, 0.20527813731-0.16226799892i, 0.371030432793+0.755136417521i]}, {"Frequency"=8383126375.0, "S Parameters"=[0.270732937477+0.828314282893i, 0.206869389706-0.165223365944i, 0.203594135171-0.164106378889i, 0.374917290475+0.75204814268i]}, {"Frequency"=8388438812.5, "S Parameters"=[0.274960963278+0.826018980842i, 0.205157025298-0.166895334022i, 0.201835105889-0.165832054815i, 0.378817861283+0.749166973755i]}, {"Frequency"=8393751250.0, "S Parameters"=[0.279245657719+0.823917558888i, 0.203483452633-0.168436701068i, 0.19998623039-0.167491823302i, 0.382680049784+0.746221754063i]}, {"Frequency"=8399063687.5, "S Parameters"=[0.283529429659+0.821733007694i, 0.201735874943-0.16974715482i, 0.198085159636-0.169006716355i, 0.38640825158+0.743591764416i]}, {"Frequency"=8404376125.0, "S Parameters"=[0.288032605657+0.81959900083i, 0.199989340898-0.170998064108i, 0.196182164977-0.170301170221i, 0.390218859769+0.741083042487i]}, {"Frequency"=8409688562.5, "S Parameters"=[0.292561094466+0.817530514442i, 0.198263452454-0.172125698284i, 0.194268357246-0.171455563124i, 0.393968963596+0.738753770047i]}, {"Frequency"=8415001000.0, "S Parameters"=[0.297328528566+0.815106567069i, 0.196560651552-0.173152050617i, 0.192402561845-0.172405866957i, 0.397856842119+0.736589685857i]}, {"Frequency"=8420313437.5, "S Parameters"=[0.302410570308+0.812685506365i, 0.194871625422-0.174076414127i, 0.19069129914-0.173220647403i, 0.401657090974+0.734292019988i]}, {"Frequency"=8425625875.0, "S Parameters"=[0.307827982484+0.810670189237i, 0.193296307497-0.174934715828i, 0.189137851294-0.173936957695i, 0.405779332436+0.73208183386i]}, {"Frequency"=8430938312.5, "S Parameters"=[0.313339416705+0.808777179901i, 0.191735043811-0.175674097355i, 0.187846230125-0.174596298379i, 0.410110132654+0.729703851764i]}, {"Frequency"=8436250750.0, "S Parameters"=[0.318859163475+0.807222901657i, 0.190381395788-0.176375457727i, 0.186696126623-0.175195119331i, 0.414963338938+0.727232456429i]}, {"Frequency"=8441563187.5, "S Parameters"=[0.324224538979+0.806023410692i, 0.189148800063-0.177017025453i, 0.185647857668-0.175799947142i, 0.420148966973+0.724913040518i]}, {"Frequency"=8446875625.0, "S Parameters"=[0.329249136526+0.80489932443i, 0.18803249954-0.177596612155i, 0.184671775463-0.17645293979i, 0.425398842154+0.722712945791i]}, {"Frequency"=8452188062.5, "S Parameters"=[0.333932677146+0.803551288509i, 0.186905599746-0.178233024475i, 0.183671983215-0.177102180088i, 0.43061302444+0.720643754073i]}, {"Frequency"=8457500500.0, "S Parameters"=[0.338592643966+0.802032753611i, 0.185828067839-0.178893291136i, 0.182653684205-0.177952701621i, 0.435755373278+0.718350739256i]}, {"Frequency"=8462812937.5, "S Parameters"=[0.342932623587+0.80053784819i, 0.184793106738-0.179599028836i, 0.181654786582-0.178854669597i, 0.44077729177+0.716028746623i]}, {"Frequency"=8468125375.0, "S Parameters"=[0.347396334169+0.798663088575i, 0.183746809675-0.180368834887i, 0.180654375229-0.179731067903i, 0.44587496131+0.713463991453i]}, {"Frequency"=8473437812.5, "S Parameters"=[0.351841274421+0.796913909646i, 0.182797015894-0.181038993021i, 0.179634077269-0.180658671201i, 0.450771766739+0.710800340684i]}, {"Frequency"=8478750250.0, "S Parameters"=[0.356466732808+0.795004495698i, 0.181908796083-0.181757939454i, 0.178609289602-0.181589755314i, 0.455736966101+0.708111424748i]}, {"Frequency"=8484062687.5, "S Parameters"=[0.361082299867+0.793309363004i, 0.180991610742-0.18248967394i, 0.1776375173-0.18248928046i, 0.460837972978+0.70531450292i]}, {"Frequency"=8489375125.0, "S Parameters"=[0.365699542465+0.79141675515i, 0.18018570137-0.183194777687i, 0.17665157191-0.183402095765i, 0.465897093156+0.702656721369i]}, {"Frequency"=8494687562.5, "S Parameters"=[0.370266286601+0.789446011853i, 0.179522229951-0.183979545188i, 0.175770086068-0.18429453748i, 0.470940544708+0.700046164432i]}, {"Frequency"=8500000000.0, "S Parameters"=[0.374956595262+0.787187137689i, 0.178885529921-0.184740049498i, 0.174930510092-0.185161329175i, 0.475586261097+0.697516156764i]}]
  out "Series Resistance":cluster{"Frequencies (Hz)":dbl[], dbl[]}(graph)
  in  "S_Par_Filename":path=path "C:/temp/ESR_probe.s2p"
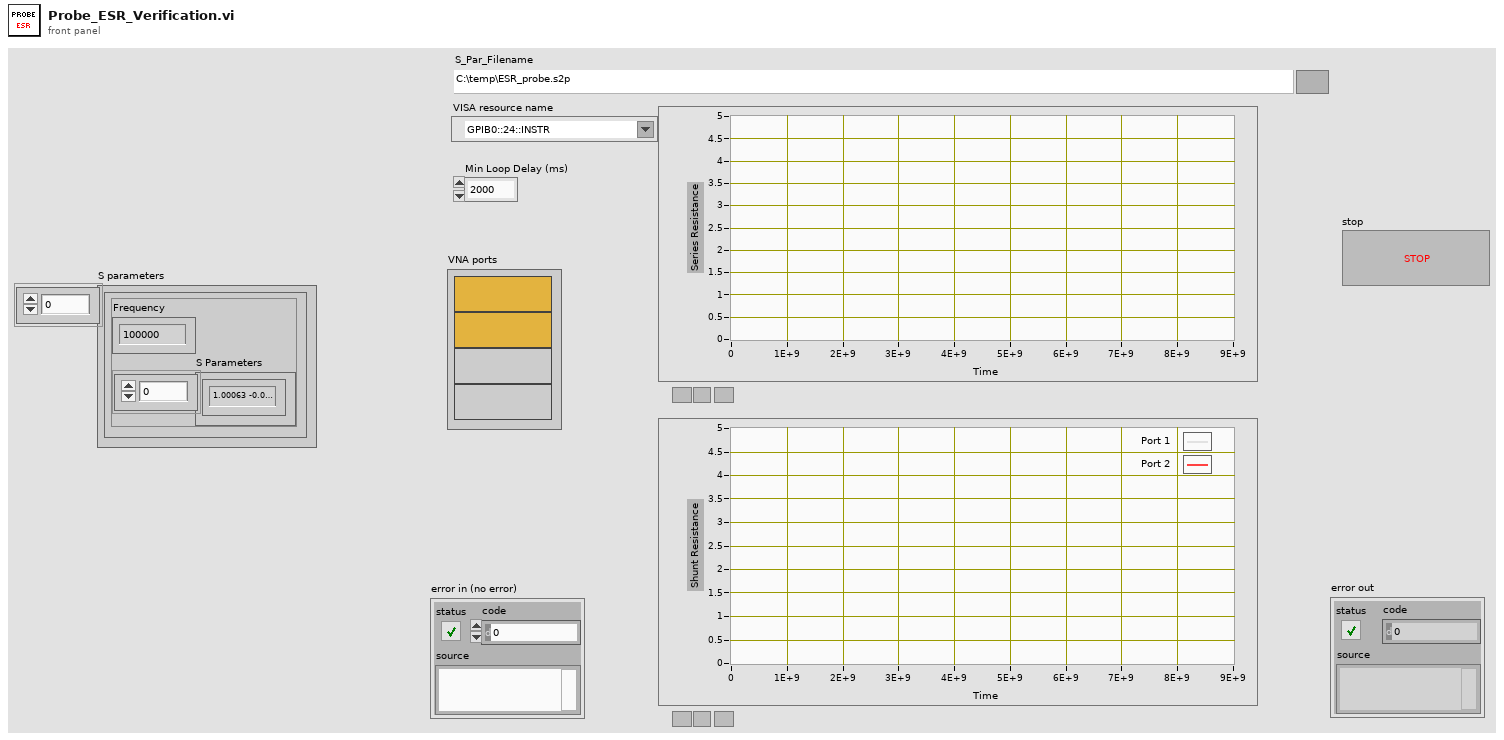
[diagram p1: front panel]
types:
  T1 = typedef "Vector Network Analyzer.lvclass/Sparameter cluster.ctl" = cluster{"Frequency":dbl, "S Parameters":cdb[]}
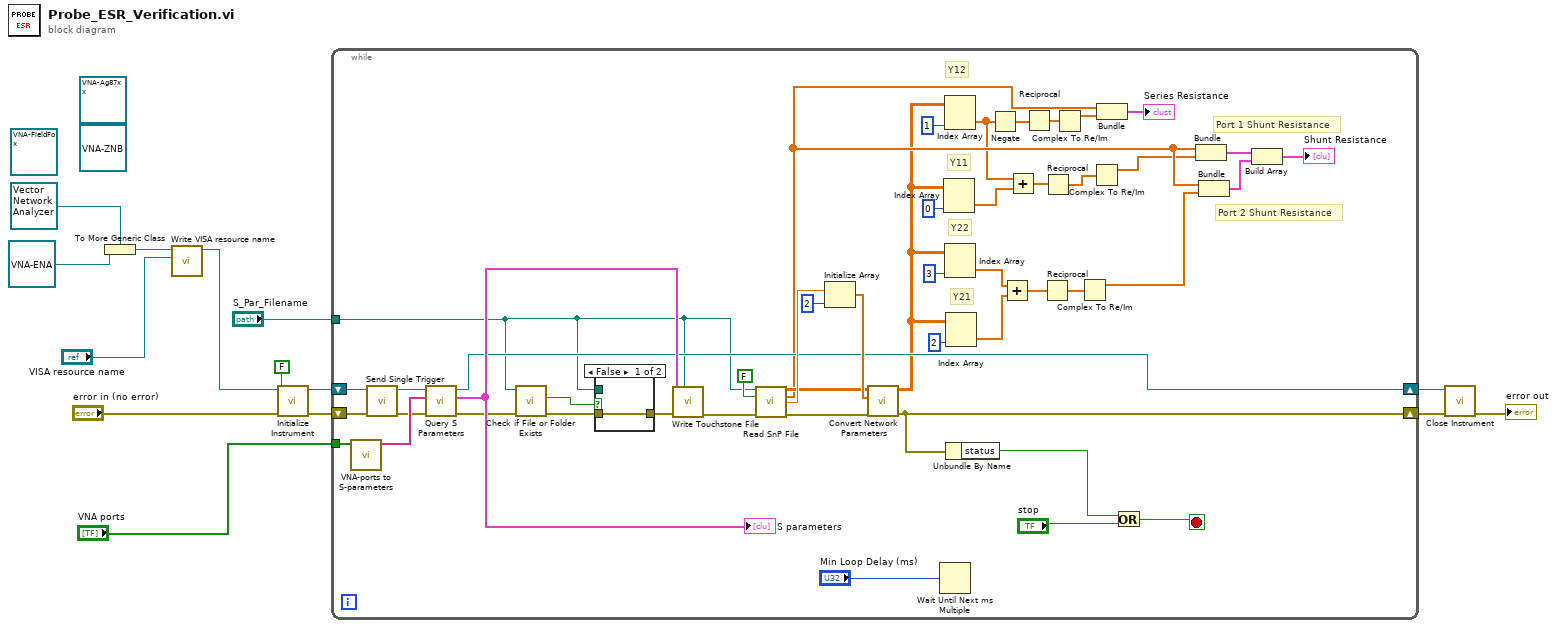
[diagram p0: block diagram]
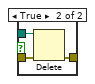
[diagram p2: hidden frame]
diagram:
  (unwired) refnum<class "VNA-FieldFox.lvclass"> refnum ("VNA-FieldFox.lvclass")
  (unwired) refnum<class "VNA-Ag87xx.lvclass"> refnum ("VNA-Ag87xx.lvclass")
  (unwired) refnum<class "VNA-ZNB.lvclass"> refnum ("VNA-ZNB.lvclass")
  n1 = To More Generic Class(target class=refnum<class "Vector Network Analyzer.lvclass"> refnum ("Vector Network Analyzer.lvclass"), reference=refnum<class "VNA-ENA.lvclass"> refnum ("VNA-ENA.lvclass")) -> (generic class reference=w12:refnum<class "Vector Network Analyzer.lvclass">)
  n2 = call "Write VISA resource name.vi"("VISA resource name"="VISA resource name", "Instrument in"=w12) -> ("Instrument out"=w14:refnum<class "Vector Network Analyzer.lvclass">)  [unwired: 9 in]
  n3 = call-dynamic "Initialize Instrument.vi"("error in (no error)"="error in (no error)", "Reset"=FALSE, "Instrument in"=w14) -> ("error out"=w6:errorcluster, "Instrument out"=w5:refnum<class "Vector Network Analyzer.lvclass">)  [unwired: 7 in]
  n4 = while {
    tunnel: "VNA ports" -> [w53]
    tunnel: "S_Par_Filename" -> [w40]
    shift-right: [w39] -> w2
    shift-left: w6 -> [w47]
    shift-right: [w44] -> w3
    shift-left: w5 -> [w46]
    stop <- w36 stop-if-true
    # "Port 2 Shunt Resistance"
    # "Port 1 Shunt Resistance"
    # "Y21"
    # "Y22"
    # "Y11"
    # "Y12"
    n5 = call "VNA-ports to S-parameters.vi"("VNA ports"=w53) -> ("Sparameters (string)"=w52:string[])  [unwired: 6 in, 4 out]
    n6 = call-dynamic "Send Single Trigger.vi"("error in (no error)"=w47, "Vector Network Analyzer in"=w46) -> ("error out"=w49:errorcluster, "Vector Network Analyzer out"=w50:refnum<class "Vector Network Analyzer.lvclass">)  [unwired: 8 in]
    n7 = call-dynamic "Query S Parameters.vi"("error in (no error)"=w49, "Sparameters (string)"=w52, "Vector Network Analyzer in"=w50) -> ("error out"=w41:errorcluster, "S parameters"=w51:T1[], "Vector Network Analyzer out"=w44:refnum<class "Vector Network Analyzer.lvclass">)  [unwired: 6 in]
    "S parameters" <- w51
    n8 = call <vilib>:"Check if File or Folder Exists.vi"("error in (no error)"=w41, "path"=w40) -> ("error out"=w35:errorcluster, "file or folder exists?"=w34:bool)  [unwired: 7 in, 1 out]
    n9 = case shown="False" w34 {
      tunnel: [w63 w66] -> w42
      tunnel: w40 -> [_ w65]
      tunnel: w35 -> [w63 w64]
      frame False {
      }
      frame True {
        n10 = Delete(path (use dialog)=w65, error in=w64) -> (error out=w66:errorcluster)  [unwired: 3 in, 2 out]
      }
    }
    n11 = call "Write Touchstone File.vi"("File Path"=w40, "Error In"=w42, "Sparameters"=w51) -> ("Error Out"=w48:errorcluster)  [unwired: 8 in]
    n12 = call-poly <vilib>:"Read SnP File.vi"("SnP File Path"=w40, "Swap Ports (False)"=FALSE, "Error In"=w48) -> ("S-parameters"=w58:cdb[][], "Frequencies (Hz)"=w32:dbl[], "Z0 (Ohm)"=w59:cdb, "Error Out"=w45:errorcluster)  [unwired: 9 in]
    n13 = Initialize Array(w59, 2 ("dimension size")) -> (w60:cdb[])
    n14 = call "Convert Network Parameters.vi"("error in (no error)"=w45, "Zc (Ohm)"=w60, "S-par Array In"=w58) -> ("error out"=w39:errorcluster, "Y/Z Array Out"=w20:cdb[][])  [unwired: 6 in, 1 out]
    n15 = Wait Until Next ms Multiple(millisecond multiple="Min Loop Delay (ms)") -> ()  [unwired: 1 out]
    n16 = Index Array(array=w20, index (col)=0 ("disabled index (col)")) -> (element=w26:cdb[])  [unwired: 1 in]
    n17 = Index Array(array=w20, index (col)=1 ("disabled index (col)")) -> (element=w27:cdb[])  [unwired: 1 in]
    n18 = Index Array(array=w20, index (col)=3 ("disabled index (col)")) -> (element=w19:cdb[])  [unwired: 1 in]
    n19 = Index Array(array=w20, index (col)=2 ("disabled index (col)")) -> (element=w18:cdb[])  [unwired: 1 in]
    n20 = Unbundle By Name(w39) -> ("status"=w38:bool)
    n21 = Negate(x=w27) -> (-x=w33:cdb[])
    n22 = Add(x=w19, y=w18) -> (x+y=w17:cdb[])
    n23 = Add(x=w27, y=w26) -> (x+y=w25:cdb[])
    n24 = Reciprocal(x=w33) -> (1/x=w56:cdb[])
    n25 = Reciprocal(x=w17) -> (1/x=w16:cdb[])
    n26 = Reciprocal(x=w25) -> (1/x=w24:cdb[])
    n27 = Complex To Re/Im(x + iy=w56) -> (x=w55:dbl[])  [unwired: 1 out]
    n28 = Complex To Re/Im(x + iy=w16) -> (x=w15:dbl[])  [unwired: 1 out]
    n29 = Complex To Re/Im(x + iy=w24) -> (x=w23:dbl[])  [unwired: 1 out]
    n30 = Bundle("Frequencies (Hz)"=w32, w55) -> (→"Series Resistance":cluster{"Frequencies (Hz)":dbl[], dbl[]})  [unwired: 1 in]
    n31 = Or(x=w38, y="stop") -> (x .or. y?=w36:bool)
    n32 = Bundle("Frequencies (Hz)"=w32, w23) -> (w31:cluster{"Frequencies (Hz)":dbl[], dbl[]})  [unwired: 1 in]
    n33 = Bundle("Frequencies (Hz)"=w32, w15) -> (w30:cluster{"Frequencies (Hz)":dbl[], dbl[]})  [unwired: 1 in]
    n34 = Build Array(w31, w30) -> (→"Shunt Resistance":cluster{"Frequencies (Hz)":dbl[], dbl[]}[])
  }
  n35 = call-dynamic "Close Instrument.vi"("error in (no error)"=w2, "Instrument in"=w3) -> ("error out"=→"error out":errorcluster)  [unwired: 8 in, 1 out]
